vi "PLC_comm.vi"() -> ()   [LabVIEW 2017]
uses:
  <vilib>/Utility/error.llb/DialogType.ctl
  Control/PLC_Comm_State.ctl
  <vilib>/DATA AHEAD/SP7/typedefs/PLC Type.ctl
  <vilib>/DATA AHEAD/SP7/typedefs/S7 Connection.ctl
  f53d9a16-31ea-4c58-9ec6-4ab155e6634a.vi
  b767813d-b0bc-4642-82b7-59e8eeaf8486.vi
  cf2a4f70-d875-4391-b4be-4b1ea527ec99.vi
  f2e501b8-8033-40fd-b99e-90a89dd29cf5.vi
  a17ecfbb-e8aa-4e6f-9723-a9b27e8c0652.vi
  adc7d8b8-ea76-443b-992e-07ffa118bf03.vi
  3deaaee4-0312-4209-8b7c-ccc637c44985.vi
  <vilib>/addons/database/Connection.llb/DB Tools Open Connec (String).vi
  <vilib>/DATA AHEAD/SP7/functions/write/write Dint array.vi
  Global/DATA LOG.vi
  <vilib>/DATA AHEAD/SP7/functions/read/read String.vi
  <vilib>/DATA AHEAD/SP7/functions/read/read Dint array.vi
  Global/Global 1.vi
  <vilib>/DATA AHEAD/SP7/functions/write/writeString.vi
  <vilib>/DATA AHEAD/SP7/functions/read/read real array.vi
  <vilib>/addons/database/NI_Database_API.lvlib
  <vilib>/DATA AHEAD/SP7/SP7.lvlib
  84f8396c-11e3-4f6e-927f-d6cb52f8486f.vi
  edb3f7e3-deb4-4efd-b63a-82a20ab466dd.vi
  737c4a97-5810-4f09-bfe1-7e6a970161fd.vi
  98a23aa7-5d76-4ce5-89a1-7ffa2d6e86d6.vi
  065602cd-1ec6-46a4-aff5-3b00a0c776c3.vi
panel:
  out "error out 4":errorcluster
  out "error out 3":errorcluster
  out "IP1 8":string
  out "PLC 8":bool
  out "IP1 7":string
  out "PLC 7":bool
  out "IP1 6":string
  out "PLC 6":bool
  out "IP1 5":string
  out "PLC 5":bool
  out "PLC 4":bool
  out "PLC 3":bool
  out "PLC 1":bool
  out "IP1 4":string
  out "IP1 3":string
  out "IP1 2":string
  out "IP1":string
  in  "stop":bool
  out "error out":errorcluster
  in  "error in (no error)":errorcluster
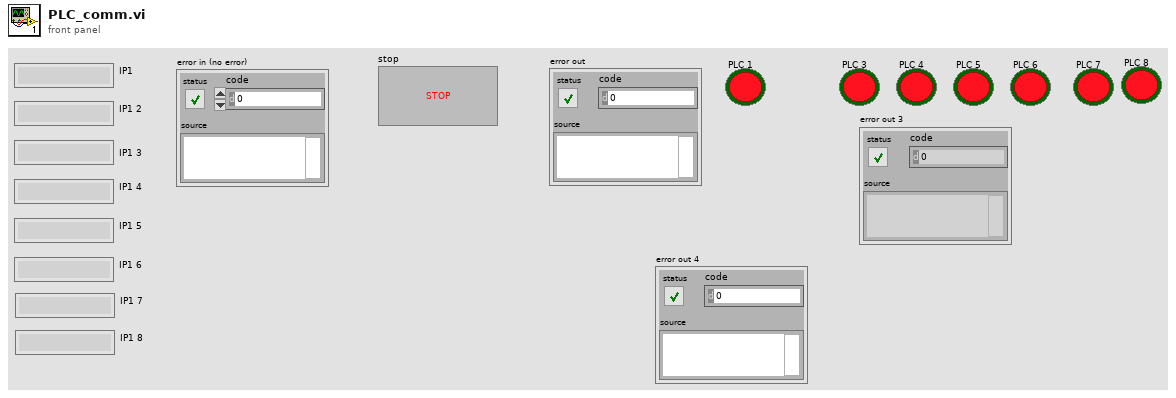
[diagram p1: front panel]
types:
  T1 = typedef "PLC_Comm_State.ctl" = enum16{"Int", "Connect", "Write", "Write2", "Write3", "Read", "Read2", "Read3", "Error", "Disconnect"}
  T2 = typedef "DialogType.ctl" = u16
  T3 = typedef "NI_Database_API.lvlib/Conn ObjectReference.ctl" = refnum<k1>
  T4 = typedef "SP7.lvlib/PLC Type.ctl" = enum16{"S7 200", "S7 300/400", "S7 1200", "S7 1500", "LOGO!8"}
  T5 = typedef "SP7.lvlib/S7 Connection.ctl" = cluster{"TCP Connection Ref":refnum<k5>, "IP address":string, "timeout ms":i32, "Connected?":bool, "PLC Type":T4, "Rack S7 400":u8, "Slot S7 400":u8, "PDU Size":u16, "connection semaphore":T6}
  T6 = typedef "Semaphore RefNum" = refnum<k1>
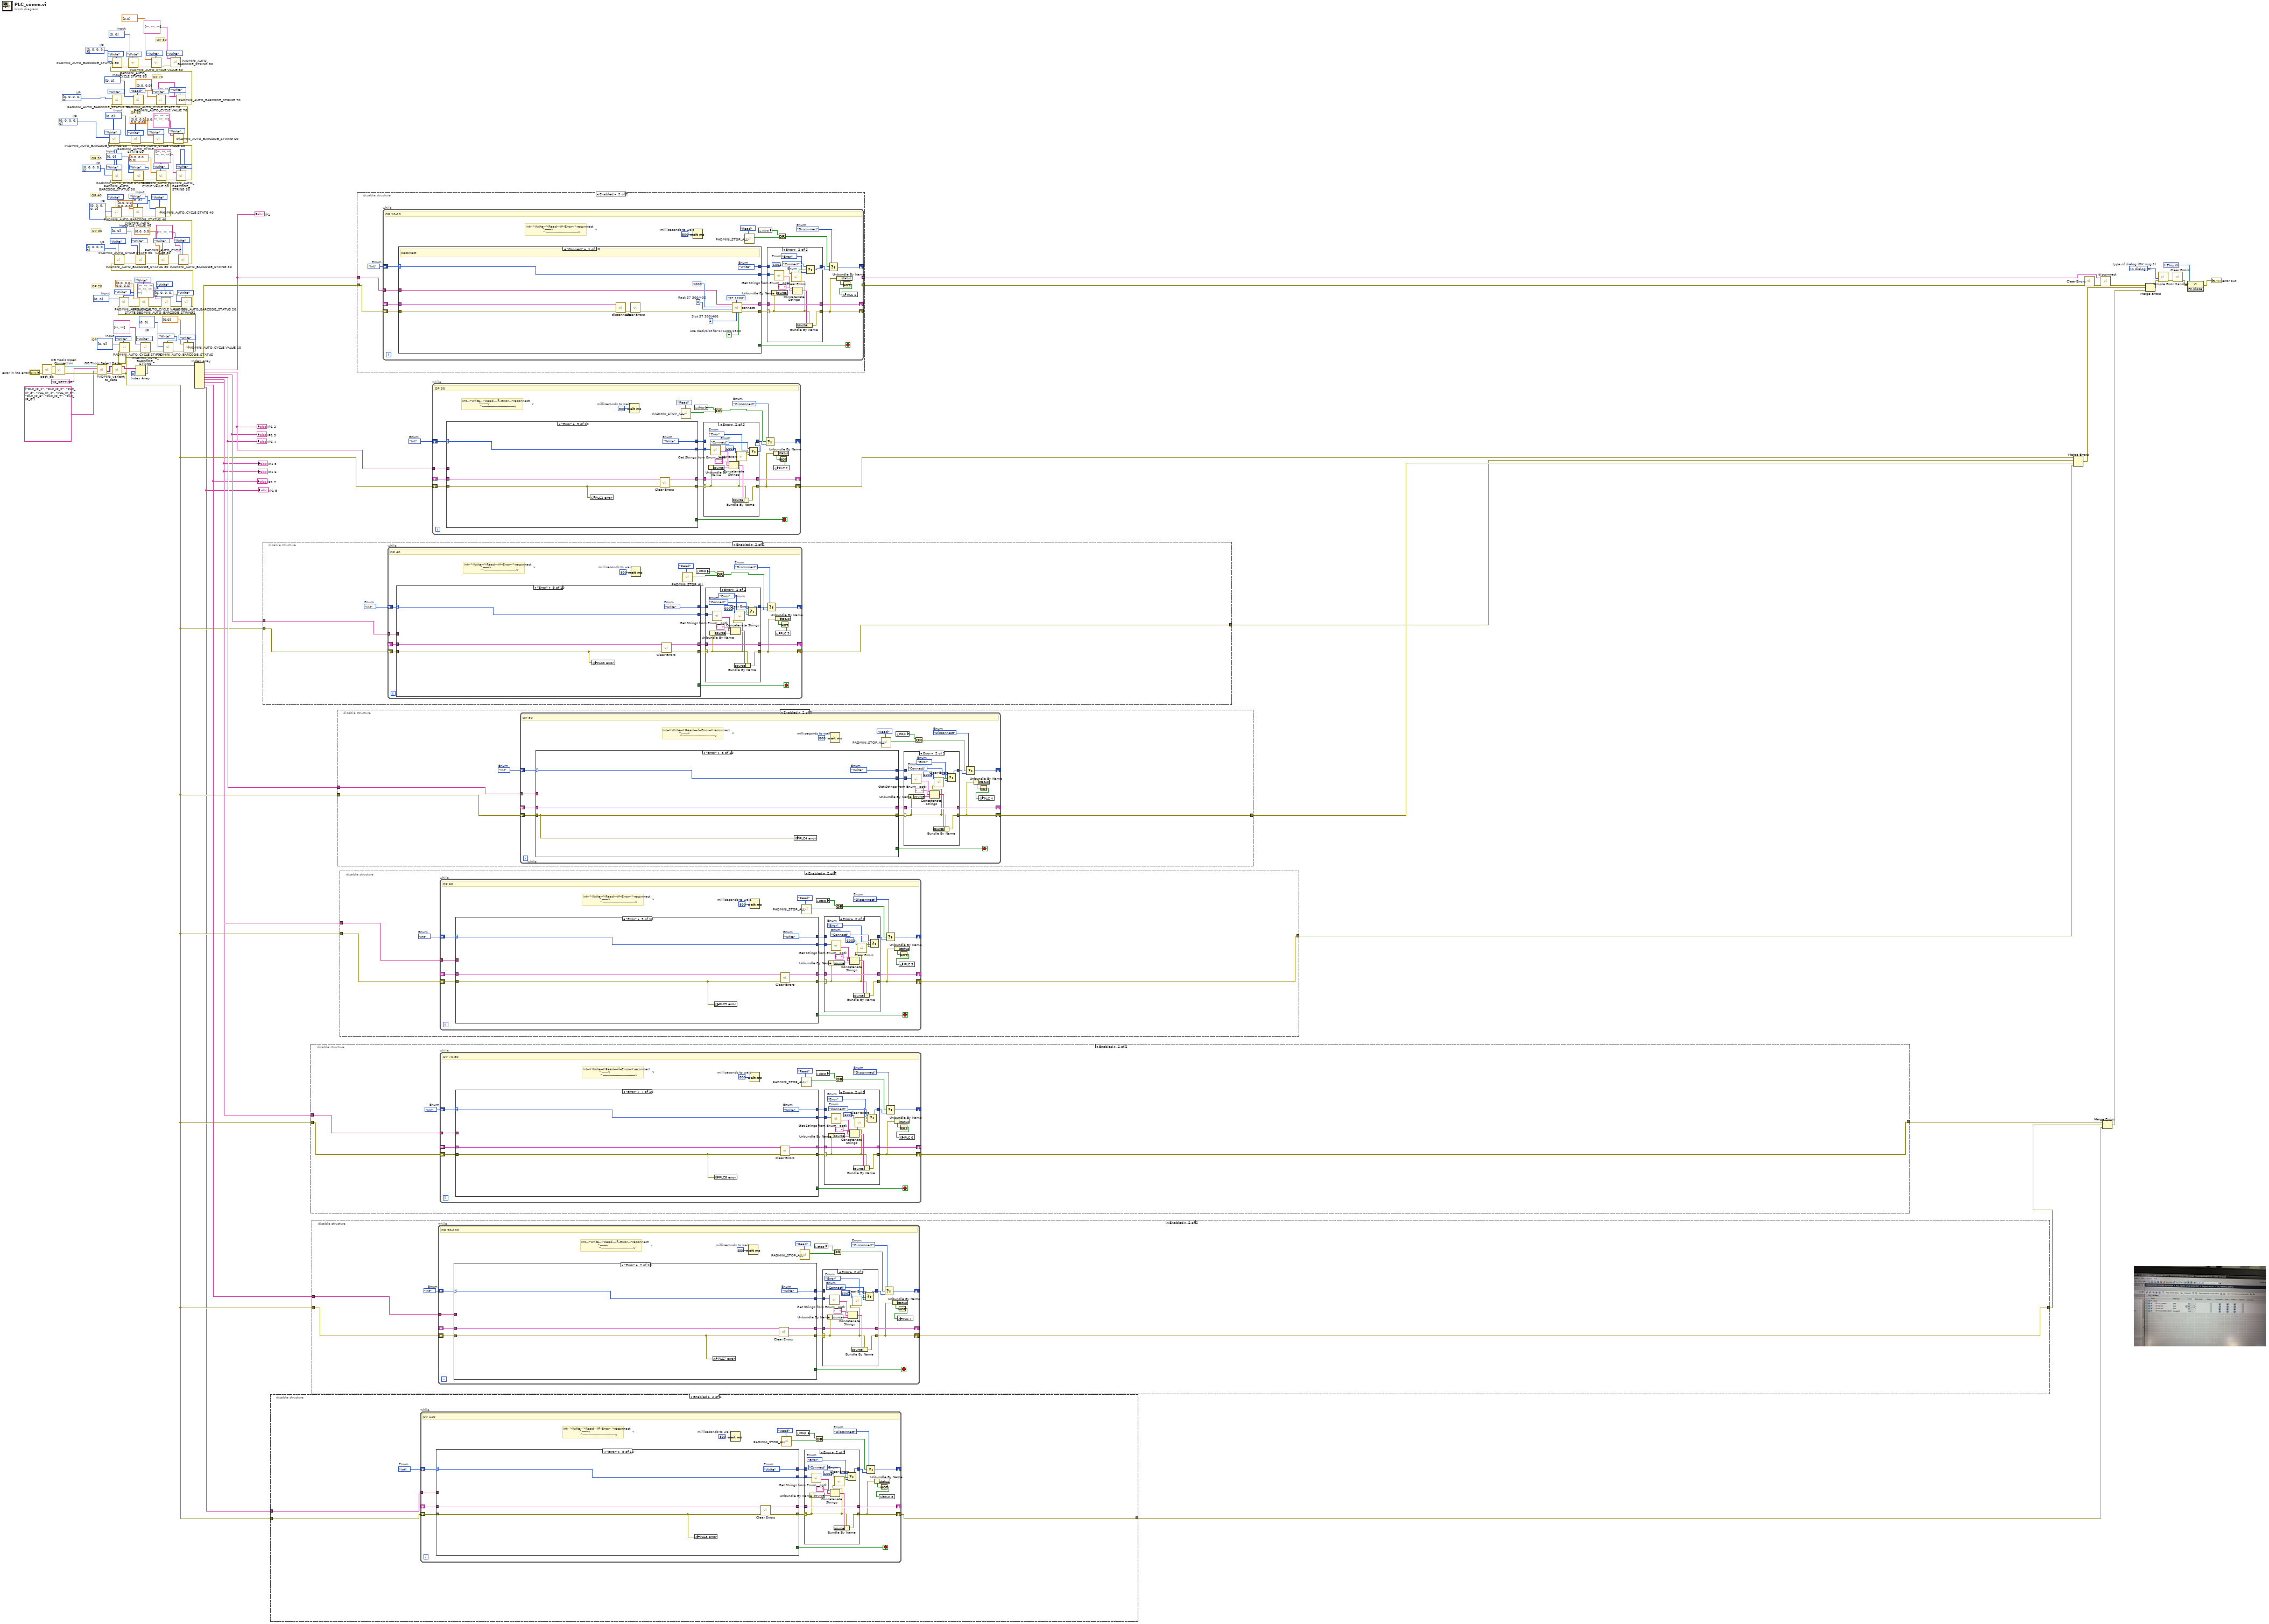
[diagram p0: block diagram]
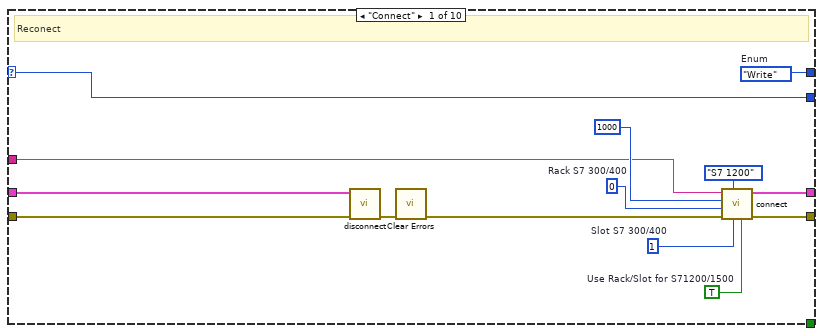
[diagram p3: hidden frame]
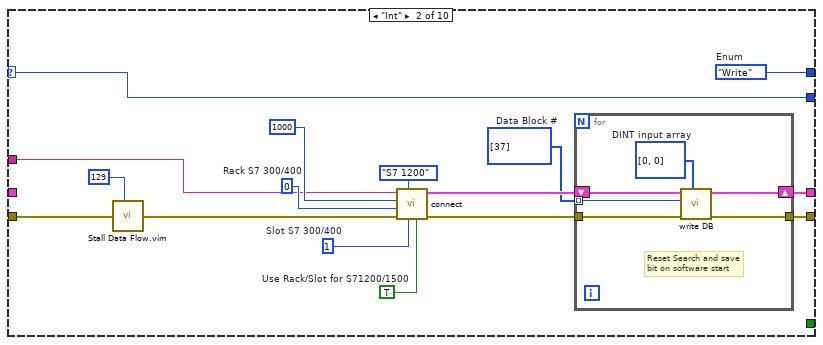
[diagram p4: hidden frame]
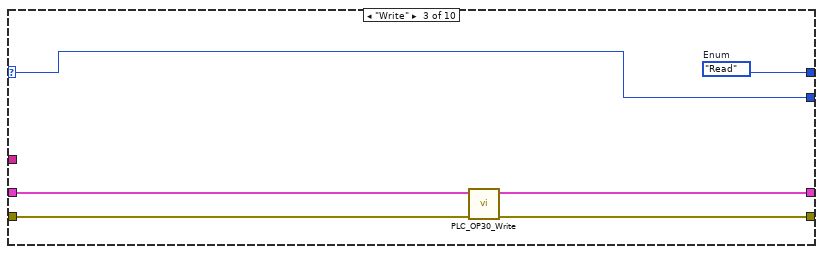
[diagram p5: hidden frame]
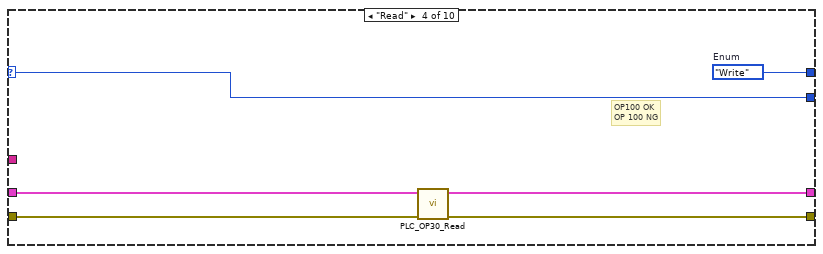
[diagram p6: hidden frame]
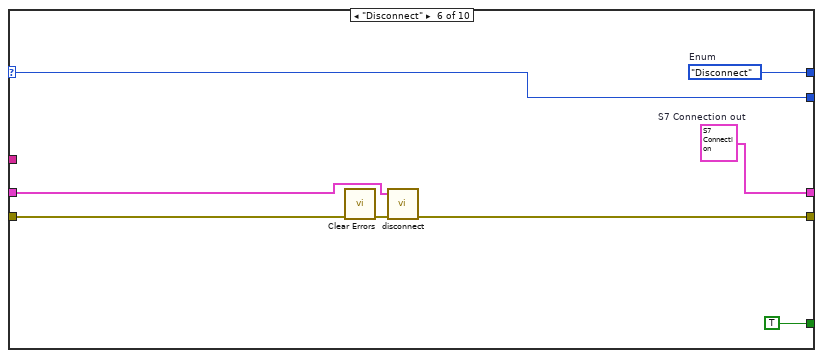
[diagram p7: hidden frame]
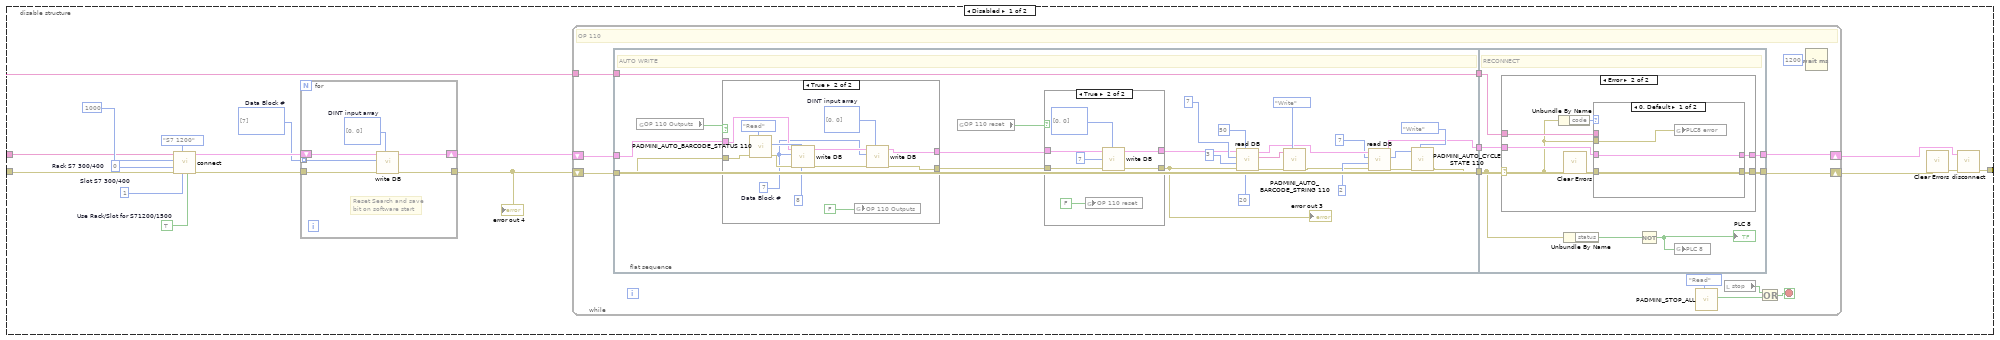
[diagram p12: hidden frame]
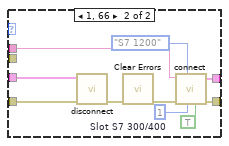
[diagram p16: hidden frame]
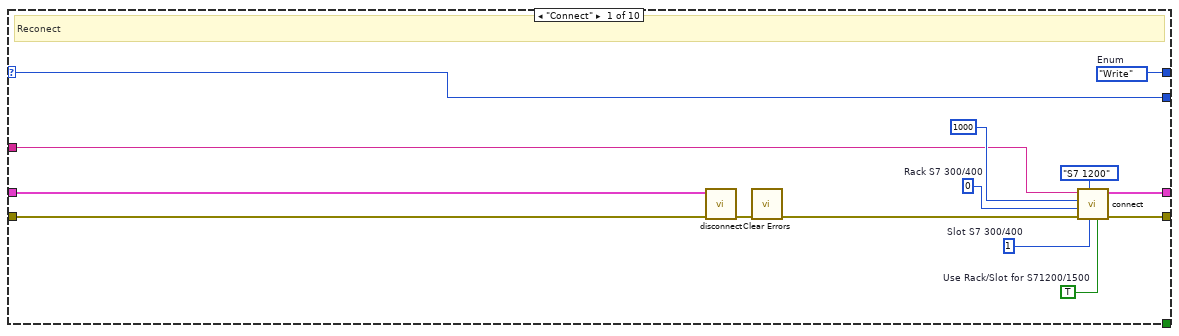
[diagram p18: hidden frame]
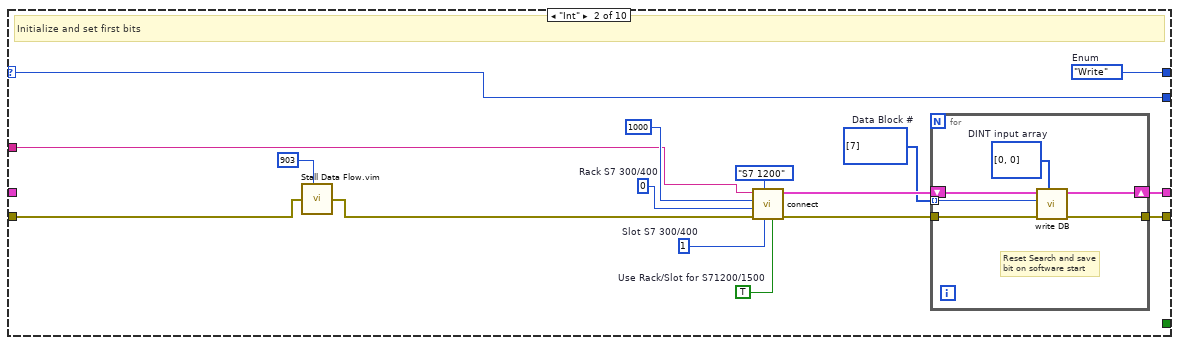
[diagram p19: hidden frame]
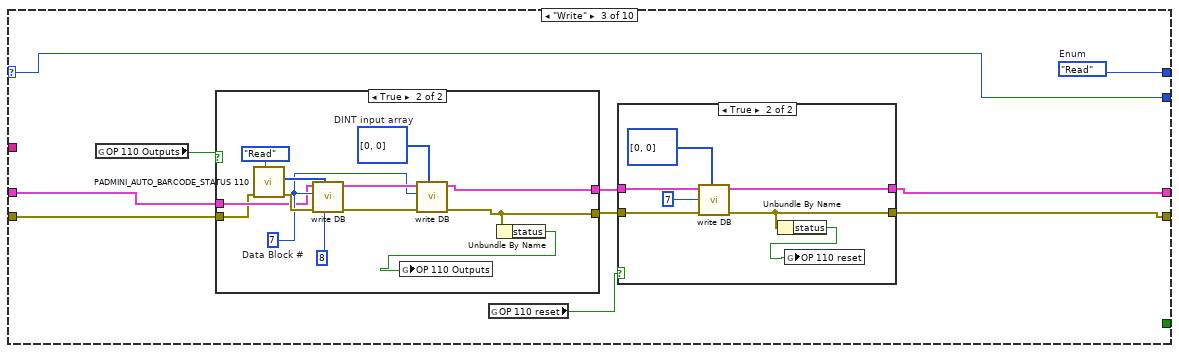
[diagram p20: hidden frame]
diagram:
  w1 = PLC_Comm_State."Int"  # Enum
  w10 = T2 0 items=["no dialog", "OK message", "continue or stop message", "OK message + warnings", "continue/stop + warnings"]  # type of dialog (OK msg:1)
  w12 = i32[] [0, 0, 0, 0, 0]  # I/P
  w13 = i32[] [0, 0]  # Input
  w15 = i32[] [0, 0]  # Input
  w16 = i32[] [0, 0]  # Input
  w18 = i32[] [0, 0]  # Input
  w14 = i32[] [0, 0, 0, 0, 0]  # I/P
  w17 = i32[] [0, 0, 0, 0, 0]  # I/P
  w19 = i32[] [0, 0, 0, 0, 0]  # I/P
  w20 = i32[] [0, 0, 0, 0, 0]  # I/P
  w21 = i32[] [0, 0]  # Input
  w22 = i32[] [0, 0]  # Input
  w23 = i32[] [0, 0, 0, 0, 0]  # I/P
  w24 = i32[] [0, 0, 0, 0, 0]  # I/P
  w25 = i32[] [0, 0]  # Input
  w26 = i32[] [0, 0]  # I/P
  w27 = i32[] [0, 0]  # Input
  # "OP 80"
  # "OP 70"
  # "OP 60"
  # "OP 50"
  # "OP 40"
  # "OP 30"
  # "OP 20"
  # "OP 10"
  n1 = call "path_db.vi"("error in"="error in (no error)") -> ("error out"=w128:errorcluster, "resulting string"=w133:string)  [unwired: 9 in]
  n2 = call-poly <vilib>:"DB Tools Open Connection.vi"("error in (no error)"=w128, "connection information"=w133) -> ("error out"=w132:errorcluster, "connection reference"=w131:T3)  [unwired: 6 in]
  n3 = call <vilib>:"DB Tools Select Data.vi"("error in (no error)"=w132, "columns"=string[] ["PLC_IP_1", "PLC_IP_2", "PLC_IP_3", "PLC_IP_4", "PLC_IP_5", "PLC_IP_6", "PLC_IP_7", "PLC_IP_8"], "table"="IP_SETTING", "connection reference"=w131) -> ("error out"=w130:errorcluster, "data"=w129:variant[][])  [unwired: 2 in, 1 out]
  n4 = call "PADMINI_varient_to_data.vi"("error in (no error)"=w130, "data"=w129) -> ("error out"=w9:errorcluster, "Array"=w124:string[][])  [unwired: 8 in]
  n5 = call "PADMINI_AUTO_CYCLE STATE.vi"("Enum"=enum16{"Read", "Write"}."Write", "error in (no error)"=w9, "Input"=w27) -> ("error out"=w114:errorcluster)  [unwired: 7 in, 1 out]
  n6 = Index Array(array=w124, index (row)=0) -> (element=w123:string[])  [unwired: 1 in]
  n7 = call "PADMINI_AUTO_BARCODE_STRING.vi"("Enum"=enum16{"Read", "Write"}."Write", "error in (no error)"=w114, "Input"=string[] ["", ""]) -> ("error out"=w111:errorcluster)  [unwired: 7 in, 1 out]
  n8 = call "PADMINI_AUTO_BARCODE_STATUS.vi"("Enum"=enum16{"Read", "Write"}."Write", "error in (no error)"=w111, "I/P"=w26) -> ("error out"=w109:errorcluster)  [unwired: 7 in, 1 out]
  n9 = call "PADMINI_AUTO_CYCLE VALUE 10.vi"("Enum"=enum16{"Read", "Write"}."Write", "error in (no error)"=w109, "Input"=dbl[] [0.0]) -> ("error out"=w103:errorcluster)  [unwired: 7 in, 1 out]
  n10 = call "PADMINI_AUTO_CYCLE STATE 20.vi"("Enum"=enum16{"Read", "Write"}."Write", "error in (no error)"=w103, "Input"=w13) -> ("error out"=w101:errorcluster)  [unwired: 7 in, 1 out]
  n11 = call "PADMINI_AUTO_CYCLE VALUE 20.vi"("Enum"=enum16{"Read", "Write"}."Write", "error in (no error)"=w101, "Input"=dbl[] [0.0, 0.0, 0.0, 0.0]) -> ("error out"=w97:errorcluster)  [unwired: 7 in, 1 out]
  n12 = call "PADMINI_AUTO_BARCODE_STRING2.vi"("Enum"=enum16{"Read", "Write"}."Write", "error in (no error)"=w97, "Input"=string[] ["", "", "", "", "", "", ""]) -> ("error out"=w95:errorcluster)  [unwired: 7 in, 1 out]
  n13 = call "PADMINI_AUTO_BARCODE_STATUS 20.vi"("Enum"=enum16{"Read", "Write"}."Write", "error in (no error)"=w95, "I/P"=w12) -> ("error out"=w93:errorcluster)  [unwired: 7 in, 1 out]
  n14 = call "PADMINI_AUTO_BARCODE_STATUS 30.vi"("Enum"=enum16{"Read", "Write"}."Write", "error in (no error)"=w93, "I/P"=w14) -> ("error out"=w90:errorcluster)  [unwired: 7 in, 1 out]
  n15 = call "PADMINI_AUTO_CYCLE STATE 30.vi"("Enum"=enum16{"Read", "Write"}."Write", "error in (no error)"=w90, "Input"=w15) -> ("error out"=w89:errorcluster)  [unwired: 7 in, 1 out]
  n16 = call "PADMINI_AUTO_CYCLE VALUE 30.vi"("Enum"=enum16{"Read", "Write"}."Write", "error in (no error)"=w89, "Input"=dbl[] [0.0, 0.0]) -> ("error out"=w86:errorcluster)  [unwired: 7 in, 1 out]
  n17 = call "PADMINI_AUTO_BARCODE_STRING 30.vi"("Enum"=enum16{"Read", "Write"}."Write", "error in (no error)"=w86, "Input"=string[] ["", "", ""]) -> ("error out"=w76:errorcluster)  [unwired: 7 in, 1 out]
  n18 = call "PADMINI_AUTO_BARCODE_STATUS 40.vi"("Enum"=enum16{"Read", "Write"}."Write", "error in (no error)"=w76, "I/P"=w17) -> ("error out"=w75:errorcluster)  [unwired: 7 in, 1 out]
  n19 = call "PADMINI_AUTO_CYCLE VALUE 40.vi"("Enum"=enum16{"Read", "Write"}."Write", "error in (no error)"=w75, "Input"=dbl[] [0.0, 0.0, 0.0, 0.0]) -> ("error out"=w74:errorcluster)  [unwired: 7 in, 1 out]
  n20 = call "PADMINI_AUTO_CYCLE STATE 40.vi"("Enum"=enum16{"Read", "Write"}."Write", "error in (no error)"=w74, "Input"=w16) -> ("error out"=w73:errorcluster)  [unwired: 7 in, 1 out]
  n21 = call "PADMINI_AUTO_BARCODE_STATUS 50.vi"("Enum"=enum16{"Read", "Write"}."Write", "error in (no error)"=w73, "I/P"=w19) -> ("error out"=w65:errorcluster)  [unwired: 7 in, 1 out]
  n22 = call "PADMINI_AUTO_CYCLE STATE 50.vi"("Enum"=enum16{"Read", "Write"}."Write", "error in (no error)"=w65, "Input"=w18) -> ("error out"=w69:errorcluster)  [unwired: 7 in, 1 out]
  n23 = call "PADMINI_AUTO_CYCLE VALUE 50.vi"("Enum"=enum16{"Read", "Write"}."Write", "error in (no error)"=w69, "Input"=dbl[] [0.0, 0.0, 0.0]) -> ("error out"=w66:errorcluster)  [unwired: 7 in, 1 out]
  n24 = call "PADMINI_AUTO_BARCODE_STRING 50.vi"("Enum"=enum16{"Read", "Write"}."Write", "error in (no error)"=w66, "Input"=string[] ["", "", "", "", "", ""]) -> ("error out"=w51:errorcluster)  [unwired: 7 in, 1 out]
  n25 = call "PADMINI_AUTO_BARCODE_STATUS 60.vi"("Enum"=enum16{"Read", "Write"}."Write", "error in (no error)"=w51, "I/P"=w20) -> ("error out"=w55:errorcluster)  [unwired: 7 in, 1 out]
  n26 = call "PADMINI_AUTO_CYCLE STATE 60.vi"("Enum"=enum16{"Read", "Write"}."Write", "error in (no error)"=w55, "Input"=w21) -> ("error out"=w57:errorcluster)  [unwired: 7 in, 1 out]
  n27 = call "PADMINI_AUTO_CYCLE VALUE 60.vi"("Enum"=enum16{"Read", "Write"}."Write", "error in (no error)"=w57, "Input"=dbl[] [0.0, 0.0, 0.0, 0.0, 0.0]) -> ("error out"=w60:errorcluster)  [unwired: 7 in, 1 out]
  n28 = call "PADMINI_AUTO_BARCODE_STRING 60.vi"("Enum"=enum16{"Read", "Write"}."Write", "error in (no error)"=w60, "Input"=string[] ["", "", "", "", "", ""]) -> ("error out"=w34:errorcluster)  [unwired: 7 in, 1 out]
  n29 = call "PADMINI_AUTO_BARCODE_STATUS 70.vi"("Enum"=enum16{"Read", "Write"}."Write", "error in (no error)"=w34, "I/P"=w23) -> ("error out"=w37:errorcluster)  [unwired: 7 in, 1 out]
  n30 = call "PADMINI_AUTO_CYCLE STATE 70.vi"("Enum"=enum16{"Read", "Write"}."Read", "error in (no error)"=w37, "Input"=w22) -> ("error out"=w49:errorcluster)  [unwired: 7 in, 1 out]
  n31 = call "PADMINI_AUTO_CYCLE VALUE 70.vi"("Enum"=enum16{"Read", "Write"}."Write", "error in (no error)"=w49, "Input"=dbl[] [0.0, 0.0]) -> ("error out"=w46:errorcluster)  [unwired: 7 in, 1 out]
  n32 = call "PADMINI_AUTO_BARCODE_STRING 70.vi"("Enum"=enum16{"Read", "Write"}."Write", "error in (no error)"=w46, "Input"=string[] ["", ""]) -> ("error out"=w31:errorcluster)  [unwired: 7 in, 1 out]
  n33 = call "PADMINI_AUTO_BARCODE_STATUS 80.vi"("Enum"=enum16{"Read", "Write"}."Write", "error in (no error)"=w31, "I/P"=w24) -> ("error out"=w38:errorcluster)  [unwired: 7 in, 1 out]
  n34 = call "PADMINI_AUTO_CYCLE STATE 80.vi"("Enum"=enum16{"Read", "Write"}."Write", "error in (no error)"=w38, "Input"=w25) -> ("error out"=w42:errorcluster)  [unwired: 7 in, 1 out]
  n35 = call "PADMINI_AUTO_CYCLE VALUE 80.vi"("Enum"=enum16{"Read", "Write"}."Write", "error in (no error)"=w42, "Input"=sgl[] [0.0]) -> ("error out"=w45:errorcluster)  [unwired: 7 in, 1 out]
  n36 = call "PADMINI_AUTO_BARCODE_STRING 80.vi"("Enum"=enum16{"Read", "Write"}."Write", "error in (no error)"=w45, "Input"=string[] ["", "", ""]) -> ()  [unwired: 7 in, 2 out]
  n37 = Index Array(array=w123) -> (element #1=w82:string, element #2=w83:string, element #3=w81:string, element #4=w71:string, element #5=w61:string, element #6=w30:string, element #7=w29:string, element #8=w8:string)  [unwired: 8 in]
  "IP1" <- w82
  "IP1 2" <- w83
  "IP1 3" <- w81
  "IP1 4" <- w71
  "IP1 5" <- w61
  "IP1 6" <- w30
  "IP1 7" <- w29
  "IP1 8" <- w8
  n38 = disable-structure shown="Enabled" {
    disable-tunnel: w81 -> [w148 w270]
    disable-tunnel: w9 -> [w139 w269]
    disable-tunnel: [w134 w268] -> w3
    frame Disabled {
      w136 = TRUE  # Use Rack/Slot for S71200/1500
      w137 = u8 0  # Rack S7 300/400
      w138 = u8 1  # Slot S7 300/400
      w144 = i32[] [0, 0]  # DINT input array
      # "Reset Search and save \nbit on software start"
      n39 = call <vilib>:"connect.vi"("Use Rack/Slot for S71200/1500"=w136, "Slot S7 300/400"=w138, "PLC Type"=PLC_Type."S7 1200" ("PLC Type 2"), "error in (no error)"=w139, "Rack S7 300/400"=w137, "timeout [ms]"=1000 ("timeout [ms] 2"), "IP address"=w148) -> ("error out"=w141:errorcluster, "S7 Connection out"=w140:T5)  [unwired: 3 in]
      n40 = call-poly <vilib>:"write DB.vi"("DINT input array"=w144, "error in (no error)"=w141, "Data Block #"=u16 56, "S7 Connection in"=w140) -> ("error out"=w143:errorcluster, "S7 Connection out"=w142:T5)  [unwired: 4 in, 2 out]
      n41 = while {
        shift-right: [w153] -> w146
        shift-left: w142 -> [w163]
        shift-right: [w161] -> w147
        shift-left: w143 -> [w162]
        tunnel: w148 -> [w152]
        stop <- w155 stop-if-true
        # "OP 40"
        n42 = flat-sequence {
          tunnel: [w165] -> w159
          tunnel: [w168] -> w154
          tunnel: w162 -> [w213]
          tunnel: w163 -> [w212]
          tunnel: w152 -> [w200]
          tunnel: [w200] -> w151
          tunnel: [w241] -> w161
          tunnel: [w240] -> w153
          tunnel: w159 -> [w243]
          tunnel: w154 -> [w242]
          tunnel: w151 -> [w239]
          frame #0 {
            w193 = u16 57 ("Data Block #")
            w164 = u16 56 ("Data Block #")
            # "AUTO WRITE"
            n43 = global read "DATA LOG.vi" "OP 40 Outputs"() -> (w211:bool)
            n44 = case shown="True" w211 {
              tunnel: w212 -> [w224 w237]
              tunnel: [w225 w229] -> w198
              tunnel: [w224 w231] -> w199
              tunnel: w213 -> [w225 w234]
              frame False {
              }
              frame True {
                w238 = u16 57  # Data Block #
                n45 = call "PADMINI_AUTO_BARCODE_STATUS 40.vi"("Enum"=enum16{"Read", "Write"}."Read", "error in (no error)"=w234) -> ("error out"=w233:errorcluster, "O/P"=w235:i32[])  [unwired: 8 in]
                n46 = global write "DATA LOG.vi" "OP 40 Outputs"(FALSE) -> ()
                n47 = call-poly <vilib>:"write DB.vi"("DINT input array"=w235, "error in (no error)"=w233, "Data Block #"=w238, "S7 Connection in"=w237) -> ("error out"=w228:errorcluster, "S7 Connection out"=w230:T5)  [unwired: 4 in, 2 out]
                n48 = call-poly <vilib>:"write DB.vi"("DINT input array"=i32[] [0], "error in (no error)"=w228, "Data Block #"=u16 56, "S7 Connection in"=w230) -> ("error out"=w229:errorcluster, "S7 Connection out"=w231:T5)  [unwired: 4 in, 2 out]
              }
            }
            n49 = global read "DATA LOG.vi" "OP 40 reset"() -> (w197:bool)
            n50 = global read "DATA LOG.vi" "Auto Cycle On"() -> (w175:bool)
            n51 = case shown="True" w197 {
              tunnel: w198 -> [w214 w223]
              tunnel: [w214 w222] -> w186
              tunnel: w199 -> [w215 w221]
              tunnel: [w215 w220] -> w187
              frame False {
              }
              frame True {
                n52 = global write "DATA LOG.vi" "OP 40 reset"(FALSE) -> ()
                n53 = call-poly <vilib>:"write DB.vi"("Item offset [byte]"=u16 4 ("Data Block #"), "DINT input array"=i32[] [0], "error in (no error)"=w223, "Data Block #"=u16 56, "S7 Connection in"=w221) -> ("error out"=w222:errorcluster, "S7 Connection out"=w220:T5)  [unwired: 3 in, 2 out]
              }
            }
            n54 = Boolean To (0,1)(Boolean=w175) -> (0, 1=w174:i16)
            n55 = Build Array(w174) -> (w173:i16[])
            n56 = global read "Global 1.vi" "Filtered BARCODE selected"() -> (w196:string[])
            n57 = call-poly <vilib>:"write DB.vi"("Item offset [byte]"=u32 20, "DINT input array"=w173, "error in (no error)"=w186, "Data Block #"=w193, "S7 Connection in"=w187) -> ("error out"=w191:errorcluster, "S7 Connection out"=w190:T5)  [unwired: 3 in, 2 out]
            n58 = call-poly <vilib>:"write DB.vi"("Item offset [byte]"=u32 24, "Input STRINGS"=w196, "error in (no error)"=w191, "String length reserved in DB (default=254)"=u16 15, "Data Block #"=w193, "S7 Connection in"=w190) -> ("error out"=w188:errorcluster, "S7 Connection out"=w189:T5)  [unwired: 2 in, 2 out]
            n59 = call-poly <vilib>:"read DB.vi"("Item offset [byte]"=u32 8, "error in (no error)"=w188, "items #"=u16 4 ("Items # [byte]"), "Data Block #"=w164, "S7 Connection in"=w189) -> ("error out"=w203:errorcluster, "REAL result array"=w201:sgl[], "S7 Connection out"=w209:T5)  [unwired: 4 in]
            n60 = call "PADMINI_AUTO_CYCLE VALUE 40.vi"("Enum"=enum16{"Read", "Write"}."Write", "error in (no error)"=w203, "Input"=w201) -> ("error out"=w202:errorcluster)  [unwired: 7 in, 1 out]
            n61 = call-poly <vilib>:"read DB.vi"("Item offset [byte]"=u32 24, "String length reserved in DB (default=254)"=u16 50, "error in (no error)"=w202, "items #"=u16 1 ("Items # [byte]"), "Data Block #"=w164, "S7 Connection in"=w209) -> ("error out"=w185:errorcluster, "STRING result Array"=w178:string[], "S7 Connection out"=w183:T5)  [unwired: 2 in, 1 out]
            n62 = call-poly <vilib>:"read DB.vi"("Item offset [byte]"=u32 76, "String length reserved in DB (default=254)"=u16 10, "error in (no error)"=w185, "items #"=u16 4 ("Items # [byte]"), "Data Block #"=w164, "S7 Connection in"=w183) -> ("error out"=w184:errorcluster, "STRING result Array"=w177:string[], "S7 Connection out"=w166:T5)  [unwired: 2 in, 1 out]
            n63 = Build Array (concatenate)(w178, w177) -> (w176:string[])
            n64 = call "PADMINI_AUTO_BARCODE_STRING 40.vi"("Enum"=enum16{"Read", "Write"}."Write", "error in (no error)"=w184, "Input"=w176) -> ("error out"=w167:errorcluster)  [unwired: 7 in, 1 out]
            n65 = call-poly <vilib>:"read DB.vi"("error in (no error)"=w167, "items #"=u16 2 ("Items # [byte]"), "Data Block #"=w164, "S7 Connection in"=w166) -> ("error out"=w172:errorcluster, "DINT result array"=w171:i32[], "S7 Connection out"=w165:T5)  [unwired: 5 in]
            n66 = call "PADMINI_AUTO_CYCLE STATE 40.vi"("Enum"=enum16{"Read", "Write"}."Write", "error in (no error)"=w172, "Input"=w171) -> ("error out"=w168:errorcluster)  [unwired: 7 in, 1 out]
          }
          frame #1 {
            # "RECONNECT"
            n67 = case shown="Error" w242 {
              selector: w242 -> [w247 w248]
              tunnel: [w246 w252] -> w240
              tunnel: [w247 w253] -> w241
              tunnel: w243 -> [w246 w251]
              tunnel: w239 -> [_ w250]
              frame No Error {
              }
              frame Error {
                n68 = Unbundle By Name(w248) -> ("code"=w249:i32)
                n69 = call <vilib>:"Clear Errors.vi"("error in (no error)"=w248) -> ("error out"=w254:errorcluster)  [unwired: 5 in, 1 out]
                n70 = case shown="0, Default" w249 {
                  tunnel: w254 -> [w256 w267]
                  tunnel: [w256 w265] -> w253
                  tunnel: [w257 w264] -> w252
                  tunnel: w251 -> [w257 w261]
                  tunnel: w250 -> [_ w260]
                  tunnel: w248 -> [w255 _]
                  frame 0, Default {
                    n71 = global write "Global 1.vi" "PLC3 error"(w255) -> ()
                  }
                  frame 1 {
                    n72 = call <vilib>:"disconnect.vi"("error in (no error)"=w267, "S7 Connection in"=w261) -> ("error out"=w266:errorcluster)  [unwired: 8 in, 1 out]
                    n73 = call <vilib>:"Clear Errors.vi"("error in (no error)"=w266) -> ("error out"=w263:errorcluster)  [unwired: 5 in, 1 out]
                    n74 = call <vilib>:"connect.vi"("Use Rack/Slot for S71200/1500"=TRUE, "Slot S7 300/400"=u8 1, "PLC Type"=PLC_Type."S7 1200" ("PLC Type 2"), "error in (no error)"=w263, "IP address"=w260) -> ("error out"=w265:errorcluster, "S7 Connection out"=w264:T5)  [unwired: 5 in]
                  }
                }
              }
            }
            n75 = Unbundle By Name(w242) -> ("status"=w245:bool)
            n76 = Not(x=w245) -> (.not. x?=w244:bool)
            "PLC 3" <- w244
            n77 = global write "Global 1.vi" "PLC 3"(w244) -> ()
          }
        }
        n78 = call "PADMINI_STOP_ALL.vi"("Enum"=enum16{"Read", "Write"}."Read") -> ("Boolean 2"=w157:bool)  [unwired: 9 in, 1 out]
        n79 = local read "stop"() -> (w156:bool)
        n80 = Or(x=w156, y=w157) -> (x .or. y?=w155:bool)
        n81 = Wait (ms)(milliseconds to wait=u32 1200) -> ()  [unwired: 1 out]
      }
      n82 = call <vilib>:"Clear Errors.vi"("error in (no error)"=w147) -> ("error out"=w135:errorcluster)  [unwired: 5 in, 1 out]
      n83 = call <vilib>:"disconnect.vi"("error in (no error)"=w135, "S7 Connection in"=w146) -> ("error out"=w134:errorcluster)  [unwired: 8 in, 1 out]
    }
    frame Enabled {
      w271 = PLC_Comm_State."Int"  # Enum
      n84 = while {
        shift-right: [w282] -> _
        shift-left: w271 -> [w291]
        shift-right: [w272] -> w268
        shift-left: w269 -> [w290]
        shift-right: [w285] -> _
        shift-left: _ -> [w289]
        tunnel: w270 -> [w288]
        stop <- w283 stop-if-true
        w279 = PLC_Comm_State."Disconnect"  # Enum
        w287 = u32 800  # milliseconds to wait
        # "Int-->Write-->Read---if--Error-->reconnect\n               ^------v                                       v\n                ^------------------------------v"
        # "OP 40"
        n85 = case shown="\"Error\"" w291 {
          selector: w291 -> [w310 w328 w366 w419 w431 w435 _ _ _ _]
          tunnel: [w315 w330 w347 w394 w432 w440 w442 w445 w447 w449] -> w292
          tunnel: [w316 w326 w345 w392 w433 w437 w443 w444 w446 w448] -> w284
          tunnel: w290 -> [w313 w324 w348 w395 w429 w438 w442 w445 w447 w449]
          tunnel: w289 -> [w311 _ w346 w393 w433 w439 w443 w444 w446 w448]
          tunnel: w288 -> [w317 w329 _ _ _ _ _ _ _ _]
          tunnel: [w309 w327 w365 w418 w430 w434 _ _ _ _] -> w286
          tunnel: [_ _ _ _ _ TRUE _ _ _ _] -> w283
          tunnel: [w310 w328 w366 w419 w431 w435 _ _ _ _] -> w280
          frame "Connect" {
            w309 = PLC_Comm_State."Write"  # Enum
            w322 = TRUE  # Use Rack/Slot for S71200/1500
            w321 = u8 1  # Slot S7 300/400
            w319 = u8 0  # Rack S7 300/400
            # "Reconect"
            n86 = call <vilib>:"disconnect.vi"("error in (no error)"=w313, "S7 Connection in"=w311) -> ("error out"=w314:errorcluster)  [unwired: 8 in, 1 out]
            n87 = call <vilib>:"Clear Errors.vi"("error in (no error)"=w314) -> ("error out"=w312:errorcluster)  [unwired: 5 in, 1 out]
            n88 = call <vilib>:"connect.vi"("Use Rack/Slot for S71200/1500"=w322, "Slot S7 300/400"=w321, "PLC Type"=PLC_Type."S7 1200" ("PLC Type 2"), "error in (no error)"=w312, "Rack S7 300/400"=w319, "timeout [ms]"=1000 ("timeout [ms] 2"), "IP address"=w317) -> ("error out"=w315:errorcluster, "S7 Connection out"=w316:T5)  [unwired: 3 in]
          }
          frame "Int" {
            w327 = PLC_Comm_State."Write"  # Enum
            w331 = TRUE  # Use Rack/Slot for S71200/1500
            w332 = u8 1  # Slot S7 300/400
            w333 = u8 0  # Rack S7 300/400
            w334 = u16[] [56]  # Data Block #
            n89 = call "Stall Data Flow.vim"("value in"=w324, "milliseconds to wait"=u32 258) -> ("value out"=w323:errorcluster)  [unwired: 1 out]
            n90 = call <vilib>:"connect.vi"("Use Rack/Slot for S71200/1500"=w331, "Slot S7 300/400"=w332, "PLC Type"=PLC_Type."S7 1200" ("PLC Type 2"), "error in (no error)"=w323, "Rack S7 300/400"=w333, "timeout [ms]"=1000 ("timeout [ms] 2"), "IP address"=w329) -> ("error out"=w336:errorcluster, "S7 Connection out"=w335:T5)  [unwired: 3 in]
            n91 = for {
              tunnel: w334 -> [w344] mode=indexing
              shift-right: [w342] -> w326
              shift-left: w335 -> [w340]
              tunnel: w336 -> [w341]
              tunnel: [w339] -> w330
              w343 = i32[] [0, 0]  # DINT input array
              # "Reset Search and save \nbit on software start"
              n92 = call-poly <vilib>:"write DB.vi"("DINT input array"=w343, "error in (no error)"=w341, "Data Block #"=w344, "S7 Connection in"=w340) -> ("error out"=w339:errorcluster, "S7 Connection out"=w342:T5)  [unwired: 4 in, 2 out]
            }
          }
          frame "Write" {
            w350 = u16 57 ("Data Block #")
            w365 = PLC_Comm_State."Read"  # Enum
            n93 = global read "DATA LOG.vi" "OP 40 Outputs"() -> (w364:bool)
            n94 = case shown="True" w364 {
              tunnel: w346 -> [w377 w379]
              tunnel: [w378 w381] -> w362
              tunnel: [w377 w386] -> w363
              tunnel: w348 -> [w378 w388]
              frame False {
              }
              frame True {
                w391 = u16 57  # Data Block #
                n95 = call "PADMINI_AUTO_BARCODE_STATUS 40.vi"("Enum"=enum16{"Read", "Write"}."Read", "error in (no error)"=w388) -> ("error out"=w387:errorcluster, "O/P"=w389:i32[])  [unwired: 8 in]
                n96 = call-poly <vilib>:"write DB.vi"("DINT input array"=w389, "error in (no error)"=w387, "Data Block #"=w391, "S7 Connection in"=w379) -> ("error out"=w384:errorcluster, "S7 Connection out"=w385:T5)  [unwired: 4 in, 2 out]
                n97 = call-poly <vilib>:"write DB.vi"("DINT input array"=i32[] [0], "error in (no error)"=w384, "Data Block #"=u16 56, "S7 Connection in"=w385) -> ("error out"=w381:errorcluster, "S7 Connection out"=w386:T5)  [unwired: 4 in, 2 out]
                n98 = Unbundle By Name(w381) -> ("status"=w380:bool)
                n99 = global write "DATA LOG.vi" "OP 40 Outputs"(w380) -> ()
              }
            }
            n100 = global read "DATA LOG.vi" "OP 40 reset"() -> (w361:bool)
            n101 = case shown="True" w361 {
              tunnel: w362 -> [w367 w376]
              tunnel: [w367 w371] -> w356
              tunnel: w363 -> [w368 w375]
              tunnel: [w368 w369] -> w357
              frame False {
              }
              frame True {
                n102 = call-poly <vilib>:"write DB.vi"("Item offset [byte]"=u16 4 ("Data Block #"), "DINT input array"=i32[] [0], "error in (no error)"=w376, "Data Block #"=u16 56, "S7 Connection in"=w375) -> ("error out"=w371:errorcluster, "S7 Connection out"=w369:T5)  [unwired: 3 in, 2 out]
                n103 = Unbundle By Name(w371) -> ("status"=w370:bool)
                n104 = global write "DATA LOG.vi" "OP 40 reset"(w370) -> ()
              }
            }
            n105 = global read "DATA LOG.vi" "Auto Cycle On"() -> (w355:bool)
            n106 = global read "Global 1.vi" "Filtered BARCODE selected"() -> (w360:string[])
            n107 = Boolean To (0,1)(Boolean=w355) -> (0, 1=w354:i16)
            n108 = Build Array(w354) -> (w353:i16[])
            n109 = call-poly <vilib>:"write DB.vi"("Item offset [byte]"=u32 20, "DINT input array"=w353, "error in (no error)"=w356, "Data Block #"=w350, "S7 Connection in"=w357) -> ("error out"=w359:errorcluster, "S7 Connection out"=w358:T5)  [unwired: 3 in, 2 out]
            n110 = call-poly <vilib>:"write DB.vi"("Item offset [byte]"=u32 24, "Input STRINGS"=w360, "error in (no error)"=w359, "String length reserved in DB (default=254)"=u16 15, "Data Block #"=w350, "S7 Connection in"=w358) -> ("error out"=w347:errorcluster, "S7 Connection out"=w345:T5)  [unwired: 2 in, 2 out]
          }
          frame "Read" {
            w404 = u16 56 ("Data Block #")
            w418 = PLC_Comm_State."Write"  # Enum
            n111 = call-poly <vilib>:"read DB.vi"("Item offset [byte]"=u32 8, "error in (no error)"=w395, "items #"=u16 4 ("Items # [byte]"), "Data Block #"=w404, "S7 Connection in"=w393) -> ("error out"=w414:errorcluster, "REAL result array"=w417:sgl[], "S7 Connection out"=w415:T5)  [unwired: 4 in]
            n112 = call-poly <vilib>:"read DB.vi"("Item offset [byte]"=u32 24, "String length reserved in DB (default=254)"=u16 50, "error in (no error)"=w414, "items #"=u16 1 ("Items # [byte]"), "Data Block #"=w404, "S7 Connection in"=w415) -> ("error out"=w413:errorcluster, "STRING result Array"=w410:string[], "S7 Connection out"=w411:T5)  [unwired: 2 in, 1 out]
            n113 = call-poly <vilib>:"read DB.vi"("Item offset [byte]"=u32 76, "String length reserved in DB (default=254)"=u16 10, "error in (no error)"=w413, "items #"=u16 4 ("Items # [byte]"), "Data Block #"=w404, "S7 Connection in"=w411) -> ("error out"=w412:errorcluster, "STRING result Array"=w409:string[], "S7 Connection out"=w406:T5)  [unwired: 2 in, 1 out]
            n114 = Build Array (concatenate)(w410, w409) -> (w416:string[])
            n115 = call-poly <vilib>:"read DB.vi"("error in (no error)"=w412, "items #"=u16 2 ("Items # [byte]"), "Data Block #"=w404, "S7 Connection in"=w406) -> ("error out"=w408:errorcluster, "DINT result array"=w407:i32[], "S7 Connection out"=w392:T5)  [unwired: 5 in]
            n116 = case shown="No Error" w408 {
              selector: w408 -> [w423 w428]
              tunnel: w407 -> [w427 _]
              tunnel: w416 -> [w425 _]
              tunnel: w417 -> [w421 _]
              tunnel: [w420 w428] -> w394
              frame No Error {
                w422 = enum16{"Read", "Write"}."Write" ("Enum")
                n117 = call "PADMINI_AUTO_CYCLE VALUE 40.vi"("Enum"=w422, "error in (no error)"=w423, "Input"=w421) -> ("error out"=w424:errorcluster)  [unwired: 7 in, 1 out]
                n118 = call "PADMINI_AUTO_BARCODE_STRING 40.vi"("Enum"=w422, "error in (no error)"=w424, "Input"=w425) -> ("error out"=w426:errorcluster)  [unwired: 7 in, 1 out]
                n119 = call "PADMINI_AUTO_CYCLE STATE 40.vi"("Enum"=w422, "error in (no error)"=w426, "Input"=w427) -> ("error out"=w420:errorcluster)  [unwired: 7 in, 1 out]
              }
              frame Error {
              }
            }
          }
          frame "Error" {
            w430 = PLC_Comm_State."Write"  # Enum
            n120 = global write "Global 1.vi" "PLC3 error"(w429) -> ()
            n121 = call <vilib>:"Clear Errors.vi"("error in (no error)"=w429) -> ("error out"=w432:errorcluster)  [unwired: 5 in, 1 out]
          }
          frame "Disconnect" {
            w434 = PLC_Comm_State."Disconnect"  # Enum
            w437 = T5 {"TCP Connection Ref"=refnum, "IP address"="", "timeout ms"=5000, "Connected?"=FALSE, "PLC Type"=enum."S7 1200", "Rack S7 400"=0, "Slot S7 400"=0, "PDU Size"=0, "connection semaphore"=refnum}  # S7 Connection out
            n122 = call <vilib>:"Clear Errors.vi"("error in (no error)"=w438) -> ("error out"=w441:errorcluster)  [unwired: 5 in, 1 out]
            n123 = call <vilib>:"disconnect.vi"("error in (no error)"=w441, "S7 Connection in"=w439) -> ("error out"=w440:errorcluster)  [unwired: 8 in, 1 out]
          }
          frame "Write2" {
            # "No Use"
          }
          frame "Write3" {
            # "No Use"
          }
          frame "Read2" {
            # "No Use"
          }
          frame "Read3" {
            # "No Use"
          }
        }
        n124 = Wait (ms)(milliseconds to wait=w287) -> ()  [unwired: 1 out]
        n125 = call "PADMINI_STOP_ALL.vi"("Enum"=enum16{"Read", "Write"}."Read") -> ("Boolean 2"=w278:bool)  [unwired: 9 in, 1 out]
        n126 = local read "stop"() -> (w277:bool)
        n127 = case shown="Error" w292 {
          selector: w292 -> [w295 w298]
          tunnel: [w295 w302] -> w272
          tunnel: [w294 w297] -> w281
          tunnel: w286 -> [w294 _]
          tunnel: [w293 w308] -> w285
          tunnel: w284 -> [w293 w308]
          tunnel: w280 -> [_ w306]
          frame No Error {
          }
          frame Error {
            w299 = PLC_Comm_State."Connect"  # Enum
            w296 = PLC_Comm_State."Error"  # Enum
            n128 = Unbundle By Name(w298) -> ("source"=w307:string)
            n129 = call <userlib>:"Get Strings from Enum__ogtk.vi"("Enum"=w306) -> ("String Value"=w305:string)  [unwired: 7 in, 3 out]
            n130 = Concatenate Strings(w305, "    " ("string"), w307) -> (w303:string)
            n131 = Bundle By Name(cluster=w298, "source"=w303) -> (w302:errorcluster)
            n132 = call <vilib>:"Clear Errors.vi"("error in (no error)"=w298, "specific error code to clear (0: all)"=6002) -> ("specific error cleared?"=w301:bool)  [unwired: 4 in, 1 out]
            n133 = Select(t=w299, s=w301, f=w296) -> (s? t:f=w297:T1)
          }
        }
        n134 = Or(x=w277, y=w278) -> (x .or. y?=w275:bool)
        n135 = Select(t=w279, s=w275, f=w281) -> (s? t:f=w282:T1)
        n136 = Unbundle By Name(w272) -> ("status"=w274:bool)
        n137 = Not(x=w274) -> (.not. x?=w273:bool)
        n138 = global write "Global 1.vi" "PLC 3"(w273) -> ()
      }
    }
  }
  n139 = disable-structure shown="Enabled" {
    disable-tunnel: w9 -> [w459 w564]
    disable-tunnel: w8 -> [w457 w565]
    disable-tunnel: [w453 w563] -> w7
    frame Disabled {
      w450 = TRUE  # Use Rack/Slot for S71200/1500
      w451 = u8 1  # Slot S7 300/400
      w452 = u8 0  # Rack S7 300/400
      w458 = u16[] [7]  # Data Block #
      n140 = call <vilib>:"connect.vi"("Use Rack/Slot for S71200/1500"=w450, "Slot S7 300/400"=w451, "PLC Type"=PLC_Type."S7 1200" ("PLC Type 2"), "error in (no error)"=w459, "Rack S7 300/400"=w452, "timeout [ms]"=1000 ("timeout [ms] 2"), "IP address"=w457) -> ("error out"=w461:errorcluster, "S7 Connection out"=w460:T5)  [unwired: 3 in]
      n141 = for {
        tunnel: w458 -> [w471] mode=indexing
        shift-right: [w469] -> w464
        shift-left: w460 -> [w466]
        tunnel: w461 -> [w467]
        tunnel: [w468] -> w465
        w470 = i32[] [0, 0]  # DINT input array
        # "Reset Search and save \nbit on software start"
        n142 = call-poly <vilib>:"write DB.vi"("DINT input array"=w470, "error in (no error)"=w467, "Data Block #"=w471, "S7 Connection in"=w466) -> ("error out"=w468:errorcluster, "S7 Connection out"=w469:T5)  [unwired: 4 in, 2 out]
      }
      "error out 4" <- w465
      n143 = while {
        shift-right: [w474] -> w454
        shift-left: w464 -> [w484]
        shift-right: [w482] -> w455
        shift-left: w465 -> [w483]
        tunnel: w457 -> [w473]
        stop <- w476 stop-if-true
        # "OP 110"
        n144 = flat-sequence {
          tunnel: [w488] -> w480
          tunnel: [w489] -> w475
          tunnel: w483 -> [w507]
          tunnel: w484 -> [w508]
          tunnel: w473 -> [w509]
          tunnel: [w509] -> w472
          tunnel: [w536] -> w482
          tunnel: [w535] -> w474
          tunnel: w480 -> [w538]
          tunnel: w475 -> [w537]
          tunnel: w472 -> [w534]
          frame #0 {
            # "AUTO WRITE"
            n145 = global read "DATA LOG.vi" "OP 110 Outputs"() -> (w506:bool)
            n146 = case shown="True" w506 {
              tunnel: [w519 w524] -> w498
              tunnel: [w520 w525] -> w497
              tunnel: w507 -> [w519 w529]
              tunnel: w508 -> [w520 w528]
              frame False {
              }
              frame True {
                w521 = i32[] [0, 0]  # DINT input array
                w522 = u16 7  # Data Block #
                n147 = call "PADMINI_AUTO_BARCODE_STATUS 110.vi"("Enum"=enum16{"Read", "Write"}."Read", "error in (no error)"=w529) -> ("error out"=w531:errorcluster, "O/P"=w532:i32[])  [unwired: 8 in]
                n148 = call-poly <vilib>:"write DB.vi"("Item offset [byte]"=u32 8, "DINT input array"=w532, "error in (no error)"=w531, "Data Block #"=w522, "S7 Connection in"=w528) -> ("error out"=w523:errorcluster, "S7 Connection out"=w526:T5)  [unwired: 3 in, 2 out]
                n149 = global write "DATA LOG.vi" "OP 110 Outputs"(FALSE) -> ()
                n150 = call-poly <vilib>:"write DB.vi"("DINT input array"=w521, "error in (no error)"=w523, "Data Block #"=w522, "S7 Connection in"=w526) -> ("error out"=w524:errorcluster, "S7 Connection out"=w525:T5)  [unwired: 4 in, 2 out]
              }
            }
            n151 = global read "DATA LOG.vi" "OP 110 reset"() -> (w495:bool)
            n152 = case shown="True" w495 {
              tunnel: w498 -> [w510 w518]
              tunnel: [w510 w517] -> w499
              tunnel: w497 -> [w511 w516]
              tunnel: [w511 w515] -> w496
              frame False {
              }
              frame True {
                n153 = global write "DATA LOG.vi" "OP 110 reset"(FALSE) -> ()
                n154 = call-poly <vilib>:"write DB.vi"("DINT input array"=i32[] [0, 0], "error in (no error)"=w518, "Data Block #"=u16 7, "S7 Connection in"=w516) -> ("error out"=w517:errorcluster, "S7 Connection out"=w515:T5)  [unwired: 4 in, 2 out]
              }
            }
            "error out 3" <- w499
            n155 = call-poly <vilib>:"read DB.vi"("Item offset [byte]"=u32 20, "String length reserved in DB (default=254)"=u16 50, "error in (no error)"=w499, "items #"=u16 3 ("Items # [byte]"), "Data Block #"=u16 7, "S7 Connection in"=w496) -> ("error out"=w501:errorcluster, "STRING result Array"=w502:string[], "S7 Connection out"=w487:T5)  [unwired: 2 in, 1 out]
            n156 = call "PADMINI_AUTO_BARCODE_STRING 110.vi"("Enum"=enum16{"Read", "Write"}."Write", "error in (no error)"=w501, "Input"=w502) -> ("error out"=w490:errorcluster)  [unwired: 7 in, 1 out]
            n157 = call-poly <vilib>:"read DB.vi"("error in (no error)"=w490, "items #"=u16 2 ("Items # [byte]"), "Data Block #"=u16 7, "S7 Connection in"=w487) -> ("error out"=w494:errorcluster, "DINT result array"=w493:i32[], "S7 Connection out"=w488:T5)  [unwired: 5 in]
            n158 = call "PADMINI_AUTO_CYCLE STATE 110.vi"("Enum"=enum16{"Read", "Write"}."Write", "error in (no error)"=w494, "Input"=w493) -> ("error out"=w489:errorcluster)  [unwired: 7 in, 1 out]
          }
          frame #1 {
            # "RECONNECT"
            n159 = case shown="Error" w537 {
              selector: w537 -> [w542 w543]
              tunnel: [w541 w547] -> w535
              tunnel: [w542 w548] -> w536
              tunnel: w538 -> [w541 w546]
              tunnel: w534 -> [_ w545]
              frame No Error {
              }
              frame Error {
                n160 = Unbundle By Name(w543) -> ("code"=w544:i32)
                n161 = call <vilib>:"Clear Errors.vi"("error in (no error)"=w543) -> ("error out"=w549:errorcluster)  [unwired: 5 in, 1 out]
                n162 = case shown="0, Default" w544 {
                  tunnel: w549 -> [w551 w562]
                  tunnel: [w551 w560] -> w548
                  tunnel: [w552 w559] -> w547
                  tunnel: w546 -> [w552 w556]
                  tunnel: w545 -> [_ w555]
                  tunnel: w543 -> [w550 _]
                  frame 0, Default {
                    n163 = global write "Global 1.vi" "PLC8 error"(w550) -> ()
                  }
                  frame 1, 66 {
                    w554 = u8 1  # Slot S7 300/400
                    n164 = call <vilib>:"disconnect.vi"("error in (no error)"=w562, "S7 Connection in"=w556) -> ("error out"=w561:errorcluster)  [unwired: 8 in, 1 out]
                    n165 = call <vilib>:"Clear Errors.vi"("error in (no error)"=w561) -> ("error out"=w558:errorcluster)  [unwired: 5 in, 1 out]
                    n166 = call <vilib>:"connect.vi"("Use Rack/Slot for S71200/1500"=TRUE, "Slot S7 300/400"=w554, "PLC Type"=PLC_Type."S7 1200" ("PLC Type 2"), "error in (no error)"=w558, "IP address"=w555) -> ("error out"=w560:errorcluster, "S7 Connection out"=w559:T5)  [unwired: 5 in]
                  }
                }
              }
            }
            n167 = Unbundle By Name(w537) -> ("status"=w540:bool)
            n168 = Not(x=w540) -> (.not. x?=w539:bool)
            "PLC 8" <- w539
            n169 = global write "Global 1.vi" "PLC 8"(w539) -> ()
          }
        }
        n170 = call "PADMINI_STOP_ALL.vi"("Enum"=enum16{"Read", "Write"}."Read") -> ("Boolean 2"=w478:bool)  [unwired: 9 in, 1 out]
        n171 = local read "stop"() -> (w477:bool)
        n172 = Or(x=w477, y=w478) -> (x .or. y?=w476:bool)
        n173 = Wait (ms)(milliseconds to wait=u32 1200) -> ()  [unwired: 1 out]
      }
      n174 = call <vilib>:"Clear Errors.vi"("error in (no error)"=w455) -> ("error out"=w456:errorcluster)  [unwired: 5 in, 1 out]
      n175 = call <vilib>:"disconnect.vi"("error in (no error)"=w456, "S7 Connection in"=w454) -> ("error out"=w453:errorcluster)  [unwired: 8 in, 1 out]
    }
    frame Enabled {
      w566 = PLC_Comm_State."Int"  # Enum
      n176 = while {
        shift-right: [w578] -> _
        shift-left: w566 -> [w586]
        shift-right: [w570] -> w563
        shift-left: w564 -> [w585]
        shift-right: [w581] -> _
        shift-left: _ -> [w584]
        tunnel: w565 -> [w567]
        stop <- w579 stop-if-true
        w575 = PLC_Comm_State."Disconnect"  # Enum
        w583 = u32 800  # milliseconds to wait
        # "Int-->Write-->Read---if--Error-->reconnect\n               ^------v                                       v\n                ^------------------------------v"
        # "OP 110"
        n177 = case shown="\"Error\"" w586 {
          selector: w586 -> [w606 w623 w649 w690 w700 w704 _ _ _ _]
          tunnel: [w611 w625 w642 w676 w701 w709 w711 w714 w716 w718] -> w587
          tunnel: [w612 w624 w643 w677 w702 w706 w712 w713 w715 w717] -> w580
          tunnel: w585 -> [w609 w619 w640 w674 w698 w707 w711 w714 w716 w718]
          tunnel: w584 -> [w607 _ w641 w675 w702 w708 w712 w713 w715 w717]
          tunnel: [w605 w622 w648 w689 w699 w703 _ _ _ _] -> w582
          tunnel: [_ _ _ _ _ TRUE _ _ _ _] -> w579
          tunnel: [w606 w623 w649 w690 w700 w704 _ _ _ _] -> w576
          tunnel: w567 -> [w604 w621 _ _ _ _ _ _ _ _]
          frame "Connect" {
            w605 = PLC_Comm_State."Write"  # Enum
            w617 = TRUE  # Use Rack/Slot for S71200/1500
            w616 = u8 1  # Slot S7 300/400
            w614 = u8 0  # Rack S7 300/400
            # "Reconect"
            n178 = call <vilib>:"disconnect.vi"("error in (no error)"=w609, "S7 Connection in"=w607) -> ("error out"=w610:errorcluster)  [unwired: 8 in, 1 out]
            n179 = call <vilib>:"Clear Errors.vi"("error in (no error)"=w610) -> ("error out"=w608:errorcluster)  [unwired: 5 in, 1 out]
            n180 = call <vilib>:"connect.vi"("Use Rack/Slot for S71200/1500"=w617, "Slot S7 300/400"=w616, "PLC Type"=PLC_Type."S7 1200" ("PLC Type 2"), "error in (no error)"=w608, "Rack S7 300/400"=w614, "timeout [ms]"=1000 ("timeout [ms] 2"), "IP address"=w604) -> ("error out"=w611:errorcluster, "S7 Connection out"=w612:T5)  [unwired: 3 in]
          }
          frame "Int" {
            w622 = PLC_Comm_State."Write"  # Enum
            w626 = TRUE  # Use Rack/Slot for S71200/1500
            w627 = u8 1  # Slot S7 300/400
            w628 = u8 0  # Rack S7 300/400
            w629 = u16[] [7]  # Data Block #
            # "Initialize and set first bits"
            n181 = call "Stall Data Flow.vim"("value in"=w619, "milliseconds to wait"=u32 903) -> ("value out"=w618:errorcluster)  [unwired: 1 out]
            n182 = call <vilib>:"connect.vi"("Use Rack/Slot for S71200/1500"=w626, "Slot S7 300/400"=w627, "PLC Type"=PLC_Type."S7 1200" ("PLC Type 2"), "error in (no error)"=w618, "Rack S7 300/400"=w628, "timeout [ms]"=1000 ("timeout [ms] 2"), "IP address"=w621) -> ("error out"=w631:errorcluster, "S7 Connection out"=w630:T5)  [unwired: 3 in]
            n183 = for {
              tunnel: w629 -> [w639] mode=indexing
              shift-right: [w637] -> w624
              shift-left: w630 -> [w635]
              tunnel: w631 -> [w636]
              tunnel: [w634] -> w625
              w638 = i32[] [0, 0]  # DINT input array
              # "Reset Search and save \nbit on software start"
              n184 = call-poly <vilib>:"write DB.vi"("DINT input array"=w638, "error in (no error)"=w636, "Data Block #"=w639, "S7 Connection in"=w635) -> ("error out"=w634:errorcluster, "S7 Connection out"=w637:T5)  [unwired: 4 in, 2 out]
            }
          }
          frame "Write" {
            w648 = PLC_Comm_State."Read"  # Enum
            n185 = global read "DATA LOG.vi" "OP 110 Outputs"() -> (w647:bool)
            n186 = case shown="True" w647 {
              tunnel: [w659 w664] -> w646
              tunnel: [w660 w668] -> w645
              tunnel: w641 -> [w660 w662]
              tunnel: w640 -> [w659 w661]
              frame False {
              }
              frame True {
                w665 = i32[] [0, 0]  # DINT input array
                w666 = u16 7  # Data Block #
                n187 = call "PADMINI_AUTO_BARCODE_STATUS 110.vi"("Enum"=enum16{"Read", "Write"}."Read", "error in (no error)"=w661) -> ("error out"=w671:errorcluster, "O/P"=w672:i32[])  [unwired: 8 in]
                n188 = call-poly <vilib>:"write DB.vi"("Item offset [byte]"=u32 8, "DINT input array"=w672, "error in (no error)"=w671, "Data Block #"=w666, "S7 Connection in"=w662) -> ("error out"=w667:errorcluster, "S7 Connection out"=w669:T5)  [unwired: 3 in, 2 out]
                n189 = call-poly <vilib>:"write DB.vi"("DINT input array"=w665, "error in (no error)"=w667, "Data Block #"=w666, "S7 Connection in"=w669) -> ("error out"=w664:errorcluster, "S7 Connection out"=w668:T5)  [unwired: 4 in, 2 out]
                n190 = Unbundle By Name(w664) -> ("status"=w663:bool)
                n191 = global write "DATA LOG.vi" "OP 110 Outputs"(w663) -> ()
              }
            }
            n192 = global read "DATA LOG.vi" "OP 110 reset"() -> (w644:bool)
            n193 = case shown="True" w644 {
              tunnel: w646 -> [w650 w658]
              tunnel: [w650 w653] -> w642
              tunnel: w645 -> [w651 w657]
              tunnel: [w651 w656] -> w643
              frame False {
              }
              frame True {
                n194 = call-poly <vilib>:"write DB.vi"("DINT input array"=i32[] [0, 0], "error in (no error)"=w658, "Data Block #"=u16 7, "S7 Connection in"=w657) -> ("error out"=w653:errorcluster, "S7 Connection out"=w656:T5)  [unwired: 4 in, 2 out]
                n195 = Unbundle By Name(w653) -> ("status"=w652:bool)
                n196 = global write "DATA LOG.vi" "OP 110 reset"(w652) -> ()
              }
            }
          }
          frame "Read" {
            w689 = PLC_Comm_State."Write"  # Enum
            n197 = call-poly <vilib>:"read DB.vi"("Item offset [byte]"=u32 20, "String length reserved in DB (default=254)"=u16 50, "error in (no error)"=w674, "items #"=u16 3 ("Items # [byte]"), "Data Block #"=u16 7, "S7 Connection in"=w675) -> ("error out"=w687:errorcluster, "STRING result Array"=w688:string[], "S7 Connection out"=w684:T5)  [unwired: 2 in, 1 out]
            n198 = call-poly <vilib>:"read DB.vi"("error in (no error)"=w687, "items #"=u16 2 ("Items # [byte]"), "Data Block #"=u16 7, "S7 Connection in"=w684) -> ("error out"=w686:errorcluster, "DINT result array"=w685:i32[], "S7 Connection out"=w677:T5)  [unwired: 5 in]
            n199 = case shown="Error" w686 {
              selector: w686 -> [w695 w697]
              tunnel: w685 -> [w696 _]
              tunnel: w688 -> [w692 _]
              tunnel: [w691 w697] -> w676
              frame No Error {
                w693 = enum16{"Read", "Write"}."Write" ("Enum")
                n200 = call "PADMINI_AUTO_BARCODE_STRING 110.vi"("Enum"=w693, "error in (no error)"=w695, "Input"=w692) -> ("error out"=w694:errorcluster)  [unwired: 7 in, 1 out]
                n201 = call "PADMINI_AUTO_CYCLE STATE 110.vi"("Enum"=w693, "error in (no error)"=w694, "Input"=w696) -> ("error out"=w691:errorcluster)  [unwired: 7 in, 1 out]
              }
              frame Error {
              }
            }
          }
          frame "Error" {
            w699 = PLC_Comm_State."Write"  # Enum
            n202 = global write "Global 1.vi" "PLC8 error"(w698) -> ()
            n203 = call <vilib>:"Clear Errors.vi"("error in (no error)"=w698) -> ("error out"=w701:errorcluster)  [unwired: 5 in, 1 out]
          }
          frame "Disconnect" {
            w703 = PLC_Comm_State."Disconnect"  # Enum
            w706 = T5 {"TCP Connection Ref"=refnum, "IP address"="", "timeout ms"=5000, "Connected?"=FALSE, "PLC Type"=enum."S7 1200", "Rack S7 400"=0, "Slot S7 400"=0, "PDU Size"=0, "connection semaphore"=refnum}  # S7 Connection out
            n204 = call <vilib>:"Clear Errors.vi"("error in (no error)"=w707) -> ("error out"=w710:errorcluster)  [unwired: 5 in, 1 out]
            n205 = call <vilib>:"disconnect.vi"("error in (no error)"=w710, "S7 Connection in"=w708) -> ("error out"=w709:errorcluster)  [unwired: 8 in, 1 out]
          }
          frame "Write2" {
            # "No Use"
          }
          frame "Write3" {
            # "No Use"
          }
          frame "Read2" {
            # "No Use"
          }
          frame "Read3" {
            # "No Use"
          }
        }
        n206 = Wait (ms)(milliseconds to wait=w583) -> ()  [unwired: 1 out]
        n207 = call "PADMINI_STOP_ALL.vi"("Enum"=enum16{"Read", "Write"}."Read") -> ("Boolean 2"=w574:bool)  [unwired: 9 in, 1 out]
        n208 = local read "stop"() -> (w569:bool)
        n209 = case shown="Error" w587 {
          selector: w587 -> [w590 w591]
          tunnel: [w590 w597] -> w570
          tunnel: [w589 w593] -> w577
          tunnel: w582 -> [w589 _]
          tunnel: [w588 w603] -> w581
          tunnel: w580 -> [w588 w603]
          tunnel: w576 -> [_ w601]
          frame No Error {
          }
          frame Error {
            w594 = PLC_Comm_State."Connect"  # Enum
            w592 = PLC_Comm_State."Error"  # Enum
            n210 = Unbundle By Name(w591) -> ("source"=w602:string)
            n211 = call <userlib>:"Get Strings from Enum__ogtk.vi"("Enum"=w601) -> ("String Value"=w600:string)  [unwired: 7 in, 3 out]
            n212 = Concatenate Strings(w600, "    " ("string"), w602) -> (w598:string)
            n213 = Bundle By Name(cluster=w591, "source"=w598) -> (w597:errorcluster)
            n214 = call <vilib>:"Clear Errors.vi"("error in (no error)"=w591, "specific error code to clear (0: all)"=6002) -> ("specific error cleared?"=w596:bool)  [unwired: 4 in, 1 out]
            n215 = Select(t=w594, s=w596, f=w592) -> (s? t:f=w593:T1)
          }
        }
        n216 = Or(x=w569, y=w574) -> (x .or. y?=w572:bool)
        n217 = Select(t=w575, s=w572, f=w577) -> (s? t:f=w578:T1)
        n218 = Unbundle By Name(w570) -> ("status"=w571:bool)
        n219 = Not(x=w571) -> (.not. x?=w568:bool)
        n220 = global write "Global 1.vi" "PLC 8"(w568) -> ()
      }
    }
  }
  n221 = disable-structure shown="Enabled" {
    disable-tunnel: w30 -> [w730 w944]
    disable-tunnel: w9 -> [w724 w943]
    disable-tunnel: [w719 w941] -> w5
    frame Disabled {
      w721 = TRUE  # Use Rack/Slot for S71200/1500
      w722 = u8 1  # Slot S7 300/400
      w723 = u8 0  # Rack S7 300/400
      n222 = call <vilib>:"connect.vi"("Use Rack/Slot for S71200/1500"=w721, "Slot S7 300/400"=w722, "PLC Type"=PLC_Type."S7 1200" ("PLC Type 2"), "error in (no error)"=w724, "Rack S7 300/400"=w723, "timeout [ms]"=1000 ("timeout [ms] 2"), "IP address"=w730) -> ("error out"=w725:errorcluster, "S7 Connection out"=w726:T5)  [unwired: 3 in]
      n223 = for {
        tunnel: u16[] [80, 82] ("Data Block #") -> [w740] mode=indexing
        shift-right: [w738] -> w727
        shift-left: w726 -> [w735]
        tunnel: w725 -> [w736]
        tunnel: [w737] -> w728
        w739 = i32[] [0, 0]  # DINT input array
        # "Reset Search and save \nbit on software start"
        n224 = call-poly <vilib>:"write DB.vi"("DINT input array"=w739, "error in (no error)"=w736, "Data Block #"=w740, "S7 Connection in"=w735) -> ("error out"=w737:errorcluster, "S7 Connection out"=w738:T5)  [unwired: 4 in, 2 out]
      }
      n225 = while {
        shift-right: [w743] -> w731
        shift-left: w727 -> [w753]
        shift-right: [w751] -> w732
        shift-left: w728 -> [w752]
        tunnel: w730 -> [w742]
        stop <- w745 stop-if-true
        # "OP 70 - 80"
        n226 = flat-sequence {
          tunnel: [w755] -> w749
          tunnel: [w759] -> w744
          tunnel: w752 -> [w861]
          tunnel: w753 -> [w860]
          tunnel: w742 -> [w848]
          tunnel: [w848] -> w741
          tunnel: [w914] -> w751
          tunnel: [w913] -> w743
          tunnel: w749 -> [w916]
          tunnel: w744 -> [w915]
          tunnel: w741 -> [w912]
          frame #0 {
            w780 = u32 500  # milliseconds to wait
            w807 = u16 83 ("Data Block #")
            w830 = u16 81 ("Data Block #")
            w791 = u16 82 ("Data Block #")
            w767 = u16 80 ("Data Block #")
            # "AUTO WRITE"
            n227 = global read "DATA LOG.vi" "OP 70 Outputs"() -> (w859:bool)
            n228 = case shown="True" w859 {
              tunnel: w860 -> [w897 w910]
              tunnel: [w898 w901] -> w835
              tunnel: [w897 w902] -> w834
              tunnel: w861 -> [w898 w907]
              frame False {
              }
              frame True {
                w911 = u16 81  # Data Block #
                n229 = call "PADMINI_AUTO_BARCODE_STATUS 70.vi"("Enum"=enum16{"Read", "Write"}."Read", "error in (no error)"=w907) -> ("error out"=w906:errorcluster, "O/P"=w908:i32[])  [unwired: 8 in]
                n230 = global write "DATA LOG.vi" "OP 70 Outputs"(FALSE) -> ()
                n231 = call-poly <vilib>:"write DB.vi"("DINT input array"=w908, "error in (no error)"=w906, "Data Block #"=w911, "S7 Connection in"=w910) -> ("error out"=w899:errorcluster, "S7 Connection out"=w900:T5)  [unwired: 4 in, 2 out]
                n232 = call-poly <vilib>:"write DB.vi"("DINT input array"=i32[] [0] ("Data Byte"), "error in (no error)"=w899, "Data Block #"=u16 80, "S7 Connection in"=w900) -> ("error out"=w901:errorcluster, "S7 Connection out"=w902:T5)  [unwired: 4 in, 2 out]
              }
            }
            n233 = global read "DATA LOG.vi" "OP 70 reset"() -> (w836:bool)
            n234 = global read "DATA LOG.vi" "Auto Cycle On"() -> (w784:bool)
            n235 = case shown="True" w836 {
              tunnel: w835 -> [w872 w881]
              tunnel: [w872 w880] -> w825
              tunnel: w834 -> [w873 w879]
              tunnel: [w873 w878] -> w826
              frame False {
              }
              frame True {
                n236 = global write "DATA LOG.vi" "OP 70 reset"(FALSE) -> ()
                n237 = call-poly <vilib>:"write DB.vi"("Item offset [byte]"=u16 4 ("Data Block #"), "DINT input array"=i32[] [0], "error in (no error)"=w881, "Data Block #"=u16 80, "S7 Connection in"=w879) -> ("error out"=w880:errorcluster, "S7 Connection out"=w878:T5)  [unwired: 3 in, 2 out]
              }
            }
            n238 = Boolean To (0,1)(Boolean=w784) -> (0, 1=w783:i16)
            n239 = Build Array(w783) -> (w782:i16[])
            n240 = call "Stall Data Flow.vim"("value in"=w825, "milliseconds to wait"=w780) -> ("value out"=w781:errorcluster)  [unwired: 1 out]
            n241 = global read "Global 1.vi" "Filtered BARCODE selected"() -> (w827:string[])
            n242 = call-poly <vilib>:"write DB.vi"("Item offset [byte]"=u32 20, "DINT input array"=w782, "error in (no error)"=w781, "Data Block #"=w830, "S7 Connection in"=w826) -> ("error out"=w832:errorcluster, "S7 Connection out"=w833:T5)  [unwired: 3 in, 2 out]
            n243 = call-poly <vilib>:"write DB.vi"("Item offset [byte]"=u32 24, "Input STRINGS"=w827, "error in (no error)"=w832, "String length reserved in DB (default=254)"=u16 15, "Data Block #"=w830, "S7 Connection in"=w833) -> ("error out"=w823:errorcluster, "S7 Connection out"=w824:T5)  [unwired: 2 in, 2 out]
            n244 = call "Stall Data Flow.vim"("value in"=w823, "milliseconds to wait"=u32 300) -> ("value out"=w779:errorcluster)  [unwired: 1 out]
            n245 = call-poly <vilib>:"read DB.vi"("Item offset [byte]"=u32 8, "error in (no error)"=w779, "items #"=u16 2 ("Items # [byte]"), "Data Block #"=w767, "S7 Connection in"=w824) -> ("error out"=w851:errorcluster, "REAL result array"=w849:sgl[], "S7 Connection out"=w857:T5)  [unwired: 4 in]
            n246 = call "PADMINI_AUTO_CYCLE VALUE 70.vi"("Enum"=enum16{"Read", "Write"}."Write", "error in (no error)"=w851, "Input"=w849) -> ("error out"=w850:errorcluster)  [unwired: 7 in, 1 out]
            n247 = call "Stall Data Flow.vim"("value in"=w850, "milliseconds to wait"=u32 0) -> ("value out"=w777:errorcluster)  [unwired: 1 out]
            n248 = call-poly <vilib>:"read DB.vi"("Item offset [byte]"=u32 16, "String length reserved in DB (default=254)"=u16 50, "error in (no error)"=w777, "items #"=u16 1 ("Items # [byte]"), "Data Block #"=w767, "S7 Connection in"=w857) -> ("error out"=w816:errorcluster, "STRING result Array"=w815:string[], "S7 Connection out"=w817:T5)  [unwired: 2 in, 1 out]
            n249 = call-poly <vilib>:"read DB.vi"("Item offset [byte]"=u32 68, "String length reserved in DB (default=254)"=u16 10, "error in (no error)"=w816, "items #"=u16 1 ("Items # [byte]"), "Data Block #"=w767, "S7 Connection in"=w817) -> ("error out"=w818:errorcluster, "STRING result Array"=w819:string[], "S7 Connection out"=w766:T5)  [unwired: 2 in, 1 out]
            n250 = Build Array (concatenate)(w815, w819) -> (w813:string[])
            n251 = call "PADMINI_AUTO_BARCODE_STRING 70.vi"("Enum"=enum16{"Read", "Write"}."Write", "error in (no error)"=w818, "Input"=w813) -> ("error out"=w764:errorcluster)  [unwired: 7 in, 1 out]
            n252 = call-poly <vilib>:"read DB.vi"("error in (no error)"=w764, "items #"=u16 2 ("Items # [byte]"), "Data Block #"=w767, "S7 Connection in"=w766) -> ("error out"=w769:errorcluster, "DINT result array"=w771:i32[], "S7 Connection out"=w765:T5)  [unwired: 5 in]
            n253 = call "PADMINI_AUTO_CYCLE STATE 70.vi"("Enum"=enum16{"Read", "Write"}."Write", "error in (no error)"=w769, "Input"=w771) -> ("error out"=w754:errorcluster)  [unwired: 7 in, 1 out]
            n254 = global read "DATA LOG.vi" "OP 80 Outputs"() -> (w837:bool)
            n255 = case shown="True" w837 {
              tunnel: [w883 w886] -> w812
              tunnel: [w882 w887] -> w789
              tunnel: w754 -> [w883 w893]
              tunnel: w765 -> [w882 w890]
              frame False {
              }
              frame True {
                w896 = u16 83  # Data Block #
                n256 = call "PADMINI_AUTO_BARCODE_STATUS 80.vi"("Enum"=enum16{"Read", "Write"}."Read", "error in (no error)"=w893) -> ("error out"=w892:errorcluster, "O/P"=w894:i32[])  [unwired: 8 in]
                n257 = global write "DATA LOG.vi" "OP 80 Outputs"(FALSE) -> ()
                n258 = call-poly <vilib>:"write DB.vi"("DINT input array"=w894, "error in (no error)"=w892, "Data Block #"=w896, "S7 Connection in"=w890) -> ("error out"=w884:errorcluster, "S7 Connection out"=w885:T5)  [unwired: 4 in, 2 out]
                n259 = call-poly <vilib>:"write DB.vi"("DINT input array"=i32[] [0] ("Data Byte"), "error in (no error)"=w884, "Data Block #"=u16 82, "S7 Connection in"=w885) -> ("error out"=w886:errorcluster, "S7 Connection out"=w887:T5)  [unwired: 4 in, 2 out]
              }
            }
            n260 = global read "DATA LOG.vi" "OP 80 reset"() -> (w811:bool)
            n261 = global read "DATA LOG.vi" "Auto Cycle On"() -> (w787:bool)
            n262 = case shown="True" w811 {
              tunnel: w812 -> [w863 w871]
              tunnel: [w863 w866] -> _
              tunnel: [w863 w866] -> w801
              tunnel: w789 -> [w862 w865]
              tunnel: [w862 w864] -> w788
              frame False {
              }
              frame True {
                n263 = global write "DATA LOG.vi" "OP 80 reset"(FALSE) -> ()
                n264 = call-poly <vilib>:"write DB.vi"("Item offset [byte]"=u16 4 ("Data Block #"), "DINT input array"=i32[] [0], "error in (no error)"=w871, "Data Block #"=u16 82, "S7 Connection in"=w865) -> ("error out"=w866:errorcluster, "S7 Connection out"=w864:T5)  [unwired: 3 in, 2 out]
              }
            }
            n265 = Boolean To (0,1)(Boolean=w787) -> (0, 1=w786:i16)
            n266 = Build Array(w786) -> (w785:i16[])
            n267 = global read "Global 1.vi" "Filtered BARCODE selected"() -> (w804:string[])
            n268 = call-poly <vilib>:"write DB.vi"("Item offset [byte]"=u32 20, "DINT input array"=w785, "error in (no error)"=w801, "Data Block #"=w807, "S7 Connection in"=w788) -> ("error out"=w809:errorcluster, "S7 Connection out"=w810:T5)  [unwired: 3 in, 2 out]
            n269 = call-poly <vilib>:"write DB.vi"("Item offset [byte]"=u32 24, "Input STRINGS"=w804, "error in (no error)"=w809, "String length reserved in DB (default=254)"=u16 15, "Data Block #"=w807, "S7 Connection in"=w810) -> ("error out"=w802:errorcluster, "S7 Connection out"=w803:T5)  [unwired: 2 in, 2 out]
            n270 = call-poly <vilib>:"read DB.vi"("Item offset [byte]"=u32 8, "error in (no error)"=w802, "items #"=u16 1 ("Items # [byte]"), "Data Block #"=w791, "S7 Connection in"=w803) -> ("error out"=w845:errorcluster, "REAL result array"=w847:sgl[], "S7 Connection out"=w839:T5)  [unwired: 4 in]
            n271 = call "PADMINI_AUTO_CYCLE VALUE 80.vi"("Enum"=enum16{"Read", "Write"}."Write", "error in (no error)"=w845, "Input"=w847) -> ("error out"=w846:errorcluster)  [unwired: 7 in, 1 out]
            n272 = call "Stall Data Flow.vim"("value in"=w846, "milliseconds to wait"=u32 300) -> ("value out"=w775:errorcluster)  [unwired: 1 out]
            n273 = call-poly <vilib>:"read DB.vi"("Item offset [byte]"=u32 12, "String length reserved in DB (default=254)"=u16 50, "error in (no error)"=w775, "items #"=u16 1 ("Items # [byte]"), "Data Block #"=w791, "S7 Connection in"=w839) -> ("error out"=w796:errorcluster, "STRING result Array"=w794:string[], "S7 Connection out"=w792:T5)  [unwired: 2 in, 1 out]
            n274 = call "Stall Data Flow.vim"("value in"=w796, "milliseconds to wait"=u32 300) -> ("value out"=w773:errorcluster)  [unwired: 1 out]
            n275 = call-poly <vilib>:"read DB.vi"("Item offset [byte]"=u32 64, "String length reserved in DB (default=254)"=u16 10, "error in (no error)"=w773, "items #"=u16 2 ("Items # [byte]"), "Data Block #"=w791, "S7 Connection in"=w792) -> ("error out"=w795:errorcluster, "STRING result Array"=w800:string[], "S7 Connection out"=w756:T5)  [unwired: 2 in, 1 out]
            n276 = Build Array (concatenate)(w794, w800) -> (w793:string[])
            n277 = call "PADMINI_AUTO_BARCODE_STRING 80.vi"("Enum"=enum16{"Read", "Write"}."Write", "error in (no error)"=w795, "Input"=w793) -> ("error out"=w758:errorcluster)  [unwired: 7 in, 1 out]
            n278 = call-poly <vilib>:"read DB.vi"("error in (no error)"=w758, "items #"=u16 2 ("Items # [byte]"), "Data Block #"=u16 82, "S7 Connection in"=w756) -> ("error out"=w762:errorcluster, "DINT result array"=w760:i32[], "S7 Connection out"=w755:T5)  [unwired: 5 in]
            n279 = call "PADMINI_AUTO_CYCLE STATE 80.vi"("Enum"=enum16{"Read", "Write"}."Write", "error in (no error)"=w762, "Input"=w760) -> ("error out"=w759:errorcluster)  [unwired: 7 in, 1 out]
          }
          frame #1 {
            # "RECONNECT"
            n280 = case shown="Error" w915 {
              selector: w915 -> [w920 w921]
              tunnel: [w919 w925] -> w913
              tunnel: [w920 w926] -> w914
              tunnel: w916 -> [w919 w924]
              tunnel: w912 -> [_ w923]
              frame No Error {
              }
              frame Error {
                n281 = Unbundle By Name(w921) -> ("code"=w922:i32)
                n282 = call <vilib>:"Clear Errors.vi"("error in (no error)"=w921) -> ("error out"=w927:errorcluster)  [unwired: 5 in, 1 out]
                n283 = case shown="1, 66" w922 {
                  tunnel: w927 -> [w929 w940]
                  tunnel: [w929 w938] -> w926
                  tunnel: [w930 w937] -> w925
                  tunnel: w924 -> [w930 w934]
                  tunnel: w923 -> [_ w933]
                  tunnel: w921 -> [w928 _]
                  frame 0, Default {
                    n284 = global write "Global 1.vi" "PLC6 error"(w928) -> ()
                  }
                  frame 1, 66 {
                    n285 = call <vilib>:"disconnect.vi"("error in (no error)"=w940, "S7 Connection in"=w934) -> ("error out"=w939:errorcluster)  [unwired: 8 in, 1 out]
                    n286 = call <vilib>:"Clear Errors.vi"("error in (no error)"=w939) -> ("error out"=w936:errorcluster)  [unwired: 5 in, 1 out]
                    n287 = call <vilib>:"connect.vi"("Use Rack/Slot for S71200/1500"=TRUE, "Slot S7 300/400"=u8 1, "PLC Type"=PLC_Type."S7 1200" ("PLC Type 2"), "error in (no error)"=w936, "IP address"=w933) -> ("error out"=w938:errorcluster, "S7 Connection out"=w937:T5)  [unwired: 5 in]
                  }
                }
              }
            }
            n288 = Unbundle By Name(w915) -> ("status"=w918:bool)
            n289 = Not(x=w918) -> (.not. x?=w917:bool)
            "PLC 6" <- w917
            n290 = global write "Global 1.vi" "PLC 6"(w917) -> ()
          }
        }
        n291 = call "PADMINI_STOP_ALL.vi"("Enum"=enum16{"Read", "Write"}."Read") -> ("Boolean 2"=w747:bool)  [unwired: 9 in, 1 out]
        n292 = local read "stop"() -> (w746:bool)
        n293 = Or(x=w746, y=w747) -> (x .or. y?=w745:bool)
        n294 = Wait (ms)(milliseconds to wait=u32 1000) -> ()  [unwired: 1 out]
      }
      n295 = call <vilib>:"Clear Errors.vi"("error in (no error)"=w732) -> ("error out"=w720:errorcluster)  [unwired: 5 in, 1 out]
      n296 = call <vilib>:"disconnect.vi"("error in (no error)"=w720, "S7 Connection in"=w731) -> ("error out"=w719:errorcluster)  [unwired: 8 in, 1 out]
    }
    frame Enabled {
      w942 = PLC_Comm_State."Int"  # Enum
      n297 = while {
        shift-right: [w956] -> _
        shift-left: w942 -> [w964]
        shift-right: [w948] -> w941
        shift-left: w943 -> [w963]
        shift-right: [w959] -> _
        shift-left: _ -> [w962]
        tunnel: w944 -> [w945]
        stop <- w957 stop-if-true
        w953 = PLC_Comm_State."Disconnect"  # Enum
        w961 = u32 800  # milliseconds to wait
        # "Int-->Write-->Read---if--Error-->reconnect\n               ^------v                                       v\n                ^------------------------------v"
        # "OP 70-80"
        n298 = case shown="\"Error\"" w964 {
          selector: w964 -> [w984 w1002 w1039 w1091 w1145 w1182 w1195 w1199 _ _]
          tunnel: [w989 w1004 w1019 w1073 w1119 w1158 w1196 w1204 w1207 w1209] -> w965
          tunnel: [w990 w1003 w1018 w1074 w1118 w1157 w1197 w1201 w1206 w1208] -> w958
          tunnel: w963 -> [w987 w998 w1020 w1072 w1120 w1155 w1193 w1202 w1207 w1209]
          tunnel: w962 -> [w985 _ w1021 w1071 w1121 w1156 w1197 w1203 w1206 w1208]
          tunnel: [w983 w1001 w1038 w1092 w1144 w1183 w1194 w1198 _ _] -> w960
          tunnel: [_ _ _ _ _ _ _ TRUE _ _] -> w957
          tunnel: [w984 w1002 w1039 w1091 w1145 w1182 w1195 w1199 _ _] -> w954
          tunnel: w945 -> [w982 w1000 _ _ _ _ _ _ _ _]
          frame "Connect" {
            w983 = PLC_Comm_State."Write"  # Enum
            w995 = TRUE  # Use Rack/Slot for S71200/1500
            w994 = u8 1  # Slot S7 300/400
            w992 = u8 0  # Rack S7 300/400
            # "Reconect"
            n299 = call <vilib>:"disconnect.vi"("error in (no error)"=w987, "S7 Connection in"=w985) -> ("error out"=w988:errorcluster)  [unwired: 8 in, 1 out]
            n300 = call <vilib>:"Clear Errors.vi"("error in (no error)"=w988) -> ("error out"=w986:errorcluster)  [unwired: 5 in, 1 out]
            n301 = call <vilib>:"connect.vi"("Use Rack/Slot for S71200/1500"=w995, "Slot S7 300/400"=w994, "PLC Type"=PLC_Type."S7 1200" ("PLC Type 2"), "error in (no error)"=w986, "Rack S7 300/400"=w992, "timeout [ms]"=1000 ("timeout [ms] 2"), "IP address"=w982) -> ("error out"=w989:errorcluster, "S7 Connection out"=w990:T5)  [unwired: 3 in]
          }
          frame "Int" {
            w1001 = PLC_Comm_State."Write"  # Enum
            w1005 = TRUE  # Use Rack/Slot for S71200/1500
            w1006 = u8 1  # Slot S7 300/400
            w1007 = u8 0  # Rack S7 300/400
            # "Initialize and set first bits"
            n302 = call "Stall Data Flow.vim"("value in"=w998, "milliseconds to wait"=u32 645) -> ("value out"=w997:errorcluster)  [unwired: 1 out]
            n303 = call <vilib>:"connect.vi"("Use Rack/Slot for S71200/1500"=w1005, "Slot S7 300/400"=w1006, "PLC Type"=PLC_Type."S7 1200" ("PLC Type 2"), "error in (no error)"=w997, "Rack S7 300/400"=w1007, "timeout [ms]"=1000 ("timeout [ms] 2"), "IP address"=w1000) -> ("error out"=w1009:errorcluster, "S7 Connection out"=w1008:T5)  [unwired: 3 in]
            n304 = for {
              tunnel: u16[] [80, 82] ("Data Block #") -> [w1017] mode=indexing
              shift-right: [w1015] -> w1003
              shift-left: w1008 -> [w1013]
              tunnel: w1009 -> [w1014]
              tunnel: [w1012] -> w1004
              w1016 = i32[] [0, 0]  # DINT input array
              # "Reset Search and save \nbit on software start"
              n305 = call-poly <vilib>:"write DB.vi"("DINT input array"=w1016, "error in (no error)"=w1014, "Data Block #"=w1017, "S7 Connection in"=w1013) -> ("error out"=w1012:errorcluster, "S7 Connection out"=w1015:T5)  [unwired: 4 in, 2 out]
            }
          }
          frame "Write" {
            w1023 = u16 81 ("Data Block #")
            w1038 = PLC_Comm_State."Write2"  # Enum
            # "OP 70 Write"
            n306 = global read "DATA LOG.vi" "OP 70 Outputs"() -> (w1037:bool)
            n307 = case shown="True" w1037 {
              tunnel: w1021 -> [w1053 w1066]
              tunnel: [w1054 w1055] -> w1035
              tunnel: [w1053 w1059] -> w1034
              tunnel: w1020 -> [w1054 w1063]
              frame False {
              }
              frame True {
                w1067 = u16 81  # Data Block #
                n308 = call "PADMINI_AUTO_BARCODE_STATUS 70.vi"("Enum"=enum16{"Read", "Write"}."Read", "error in (no error)"=w1063) -> ("error out"=w1062:errorcluster, "O/P"=w1064:i32[])  [unwired: 8 in]
                n309 = call-poly <vilib>:"write DB.vi"("DINT input array"=w1064, "error in (no error)"=w1062, "Data Block #"=w1067, "S7 Connection in"=w1066) -> ("error out"=w1057:errorcluster, "S7 Connection out"=w1058:T5)  [unwired: 4 in, 2 out]
                n310 = call-poly <vilib>:"write DB.vi"("DINT input array"=i32[] [0] ("Data Byte"), "error in (no error)"=w1057, "Data Block #"=u16 80, "S7 Connection in"=w1058) -> ("error out"=w1056:errorcluster, "S7 Connection out"=w1059:T5)  [unwired: 4 in, 2 out]
                n311 = case shown="No Error" w1056 {
                  selector: w1056 -> [w1068 w1070]
                  tunnel: [w1068 w1070] -> w1055
                  frame No Error {
                    n312 = global write "DATA LOG.vi" "OP 70 Outputs"(FALSE) -> ()
                  }
                  frame Error {
                  }
                }
              }
            }
            n313 = global read "DATA LOG.vi" "OP 70 reset"() -> (w1036:bool)
            n314 = global read "DATA LOG.vi" "Auto Cycle On"() -> (w1028:bool)
            n315 = case shown="True" w1036 {
              tunnel: w1035 -> [w1040 w1049]
              tunnel: [w1040 w1042] -> w1029
              tunnel: w1034 -> [w1041 w1048]
              tunnel: [w1041 w1047] -> w1030
              frame False {
              }
              frame True {
                n316 = call-poly <vilib>:"write DB.vi"("Item offset [byte]"=u16 4 ("Data Block #"), "DINT input array"=i32[] [0], "error in (no error)"=w1049, "Data Block #"=u16 80, "S7 Connection in"=w1048) -> ("error out"=w1043:errorcluster, "S7 Connection out"=w1047:T5)  [unwired: 3 in, 2 out]
                n317 = case shown="No Error" w1043 {
                  selector: w1043 -> [w1050 w1052]
                  tunnel: [w1050 w1052] -> w1042
                  frame No Error {
                    n318 = global write "DATA LOG.vi" "OP 70 reset"(FALSE) -> ()
                  }
                  frame Error {
                  }
                }
              }
            }
            n319 = Boolean To (0,1)(Boolean=w1028) -> (0, 1=w1027:i16)
            n320 = Build Array(w1027) -> (w1026:i16[])
            n321 = global read "Global 1.vi" "Filtered BARCODE selected"() -> (w1031:string[])
            n322 = call-poly <vilib>:"write DB.vi"("Item offset [byte]"=u32 20, "DINT input array"=w1026, "error in (no error)"=w1029, "Data Block #"=w1023, "S7 Connection in"=w1030) -> ("error out"=w1032:errorcluster, "S7 Connection out"=w1033:T5)  [unwired: 3 in, 2 out]
            n323 = call-poly <vilib>:"write DB.vi"("Item offset [byte]"=u32 24, "Input STRINGS"=w1031, "error in (no error)"=w1032, "String length reserved in DB (default=254)"=u16 15, "Data Block #"=w1023, "S7 Connection in"=w1033) -> ("error out"=w1019:errorcluster, "S7 Connection out"=w1018:T5)  [unwired: 2 in, 2 out]
          }
          frame "Write2" {
            w1076 = u16 83 ("Data Block #")
            w1092 = PLC_Comm_State."Read"  # Enum
            # "op 80 wirte 2"
            n324 = global read "DATA LOG.vi" "OP 80 Outputs"() -> (w1090:bool)
            n325 = case shown="True" w1090 {
              tunnel: [w1104 w1106] -> w1089
              tunnel: [w1103 w1109] -> w1083
              tunnel: w1072 -> [w1104 w1114]
              tunnel: w1071 -> [w1103 w1112]
              frame False {
              }
              frame True {
                w1117 = u16 83  # Data Block #
                n326 = call "PADMINI_AUTO_BARCODE_STATUS 80.vi"("Enum"=enum16{"Read", "Write"}."Read", "error in (no error)"=w1114) -> ("error out"=w1113:errorcluster, "O/P"=w1115:i32[])  [unwired: 8 in]
                n327 = call-poly <vilib>:"write DB.vi"("DINT input array"=w1115, "error in (no error)"=w1113, "Data Block #"=w1117, "S7 Connection in"=w1112) -> ("error out"=w1107:errorcluster, "S7 Connection out"=w1108:T5)  [unwired: 4 in, 2 out]
                n328 = call-poly <vilib>:"write DB.vi"("DINT input array"=i32[] [0] ("Data Byte"), "error in (no error)"=w1107, "Data Block #"=u16 82, "S7 Connection in"=w1108) -> ("error out"=w1106:errorcluster, "S7 Connection out"=w1109:T5)  [unwired: 4 in, 2 out]
                n329 = Unbundle By Name(w1106) -> ("status"=w1105:bool)
                n330 = global write "DATA LOG.vi" "OP 80 Outputs"(w1105) -> ()
              }
            }
            n331 = global read "DATA LOG.vi" "OP 80 reset"() -> (w1088:bool)
            n332 = case shown="True" w1088 {
              tunnel: w1089 -> [w1094 w1102]
              tunnel: [w1094 w1096] -> _
              tunnel: [w1094 w1096] -> w1084
              tunnel: w1083 -> [w1093 w1098]
              tunnel: [w1093 w1097] -> w1082
              frame False {
              }
              frame True {
                n333 = call-poly <vilib>:"write DB.vi"("Item offset [byte]"=u16 4 ("Data Block #"), "DINT input array"=i32[] [0], "error in (no error)"=w1102, "Data Block #"=u16 82, "S7 Connection in"=w1098) -> ("error out"=w1096:errorcluster, "S7 Connection out"=w1097:T5)  [unwired: 3 in, 2 out]
                n334 = Unbundle By Name(w1096) -> ("status"=w1095:bool)
                n335 = global write "DATA LOG.vi" "OP 80 reset"(w1095) -> ()
              }
            }
            n336 = global read "DATA LOG.vi" "Auto Cycle On"() -> (w1081:bool)
            n337 = Boolean To (0,1)(Boolean=w1081) -> (0, 1=w1080:i16)
            n338 = Build Array(w1080) -> (w1079:i16[])
            n339 = global read "Global 1.vi" "Filtered BARCODE selected"() -> (w1085:string[])
            n340 = call-poly <vilib>:"write DB.vi"("Item offset [byte]"=u32 20, "DINT input array"=w1079, "error in (no error)"=w1084, "Data Block #"=w1076, "S7 Connection in"=w1082) -> ("error out"=w1086:errorcluster, "S7 Connection out"=w1087:T5)  [unwired: 3 in, 2 out]
            n341 = call-poly <vilib>:"write DB.vi"("Item offset [byte]"=u32 24, "Input STRINGS"=w1085, "error in (no error)"=w1086, "String length reserved in DB (default=254)"=u16 15, "Data Block #"=w1076, "S7 Connection in"=w1087) -> ("error out"=w1073:errorcluster, "S7 Connection out"=w1074:T5)  [unwired: 2 in, 2 out]
          }
          frame "Read" {
            w1130 = u16 80 ("Data Block #")
            w1144 = PLC_Comm_State."Read2"  # Enum
            # "OP70 read"
            n342 = call-poly <vilib>:"read DB.vi"("Item offset [byte]"=u32 8, "error in (no error)"=w1120, "items #"=u16 2 ("Items # [byte]"), "Data Block #"=w1130, "S7 Connection in"=w1121) -> ("error out"=w1140:errorcluster, "REAL result array"=w1143:sgl[], "S7 Connection out"=w1141:T5)  [unwired: 4 in]
            n343 = call-poly <vilib>:"read DB.vi"("Item offset [byte]"=u32 16, "String length reserved in DB (default=254)"=u16 50, "error in (no error)"=w1140, "items #"=u16 1 ("Items # [byte]"), "Data Block #"=w1130, "S7 Connection in"=w1141) -> ("error out"=w1136:errorcluster, "STRING result Array"=w1135:string[], "S7 Connection out"=w1137:T5)  [unwired: 2 in, 1 out]
            n344 = call-poly <vilib>:"read DB.vi"("Item offset [byte]"=u32 68, "String length reserved in DB (default=254)"=u16 10, "error in (no error)"=w1136, "items #"=u16 1 ("Items # [byte]"), "Data Block #"=w1130, "S7 Connection in"=w1137) -> ("error out"=w1138:errorcluster, "STRING result Array"=w1139:string[], "S7 Connection out"=w1132:T5)  [unwired: 2 in, 1 out]
            n345 = Build Array (concatenate)(w1135, w1139) -> (w1142:string[])
            n346 = call-poly <vilib>:"read DB.vi"("error in (no error)"=w1138, "items #"=u16 2 ("Items # [byte]"), "Data Block #"=w1130, "S7 Connection in"=w1132) -> ("error out"=w1133:errorcluster, "DINT result array"=w1134:i32[], "S7 Connection out"=w1118:T5)  [unwired: 5 in]
            n347 = case shown="No Error" w1133 {
              selector: w1133 -> [w1148 w1154]
              tunnel: w1134 -> [w1153 _]
              tunnel: w1142 -> [w1152 _]
              tunnel: w1143 -> [w1149 _]
              tunnel: [w1147 w1154] -> w1119
              frame No Error {
                w1151 = enum16{"Read", "Write"}."Write" ("Enum")
                n348 = call "PADMINI_AUTO_BARCODE_STRING 70.vi"("Enum"=w1151, "error in (no error)"=w1148, "Input"=w1152) -> ("error out"=w1150:errorcluster)  [unwired: 7 in, 1 out]
                n349 = call "PADMINI_AUTO_CYCLE VALUE 70.vi"("Enum"=w1151, "error in (no error)"=w1150, "Input"=w1149) -> ("error out"=w1146:errorcluster)  [unwired: 7 in, 1 out]
                n350 = call "PADMINI_AUTO_CYCLE STATE 70.vi"("Enum"=w1151, "error in (no error)"=w1146, "Input"=w1153) -> ("error out"=w1147:errorcluster)  [unwired: 7 in, 1 out]
              }
              frame Error {
              }
            }
          }
          frame "Read2" {
            w1164 = u16 82 ("Data Block #")
            w1183 = PLC_Comm_State."Write"  # Enum
            # "Op80 Read2"
            n351 = call-poly <vilib>:"read DB.vi"("Item offset [byte]"=u32 8, "error in (no error)"=w1155, "items #"=u16 1 ("Items # [byte]"), "Data Block #"=w1164, "S7 Connection in"=w1156) -> ("error out"=w1170:errorcluster, "REAL result array"=w1181:sgl[], "S7 Connection out"=w1171:T5)  [unwired: 4 in]
            n352 = call-poly <vilib>:"read DB.vi"("Item offset [byte]"=u32 12, "String length reserved in DB (default=254)"=u16 50, "error in (no error)"=w1170, "items #"=u16 1 ("Items # [byte]"), "Data Block #"=w1164, "S7 Connection in"=w1171) -> ("error out"=w1173:errorcluster, "STRING result Array"=w1175:string[], "S7 Connection out"=w1176:T5)  [unwired: 2 in, 1 out]
            n353 = call-poly <vilib>:"read DB.vi"("Item offset [byte]"=u32 64, "String length reserved in DB (default=254)"=u16 10, "error in (no error)"=w1173, "items #"=u16 2 ("Items # [byte]"), "Data Block #"=w1164, "S7 Connection in"=w1176) -> ("error out"=w1174:errorcluster, "STRING result Array"=w1172:string[], "S7 Connection out"=w1179:T5)  [unwired: 2 in, 1 out]
            n354 = Build Array (concatenate)(w1175, w1172) -> (w1180:string[])
            n355 = call-poly <vilib>:"read DB.vi"("error in (no error)"=w1174, "items #"=u16 2 ("Items # [byte]"), "Data Block #"=u16 82, "S7 Connection in"=w1179) -> ("error out"=w1177:errorcluster, "DINT result array"=w1178:i32[], "S7 Connection out"=w1157:T5)  [unwired: 5 in]
            n356 = case shown="No Error" w1177 {
              selector: w1177 -> [w1186 w1192]
              tunnel: w1178 -> [w1191 _]
              tunnel: w1180 -> [w1189 _]
              tunnel: w1181 -> [w1188 _]
              tunnel: [w1184 w1192] -> w1158
              frame No Error {
                w1187 = enum16{"Read", "Write"}."Write" ("Enum")
                n357 = call "PADMINI_AUTO_CYCLE VALUE 80.vi"("Enum"=w1187, "error in (no error)"=w1186, "Input"=w1188) -> ("error out"=w1190:errorcluster)  [unwired: 7 in, 1 out]
                n358 = call "PADMINI_AUTO_BARCODE_STRING 80.vi"("Enum"=w1187, "error in (no error)"=w1190, "Input"=w1189) -> ("error out"=w1185:errorcluster)  [unwired: 7 in, 1 out]
                n359 = call "PADMINI_AUTO_CYCLE STATE 80.vi"("Enum"=w1187, "error in (no error)"=w1185, "Input"=w1191) -> ("error out"=w1184:errorcluster)  [unwired: 7 in, 1 out]
              }
              frame Error {
              }
            }
          }
          frame "Error" {
            w1194 = PLC_Comm_State."Write"  # Enum
            n360 = global write "Global 1.vi" "PLC6 error"(w1193) -> ()
            n361 = call <vilib>:"Clear Errors.vi"("error in (no error)"=w1193) -> ("error out"=w1196:errorcluster)  [unwired: 5 in, 1 out]
          }
          frame "Disconnect" {
            w1198 = PLC_Comm_State."Disconnect"  # Enum
            w1201 = T5 {"TCP Connection Ref"=refnum, "IP address"="", "timeout ms"=5000, "Connected?"=FALSE, "PLC Type"=enum."S7 1200", "Rack S7 400"=0, "Slot S7 400"=0, "PDU Size"=0, "connection semaphore"=refnum}  # S7 Connection out
            n362 = call <vilib>:"Clear Errors.vi"("error in (no error)"=w1202) -> ("error out"=w1205:errorcluster)  [unwired: 5 in, 1 out]
            n363 = call <vilib>:"disconnect.vi"("error in (no error)"=w1205, "S7 Connection in"=w1203) -> ("error out"=w1204:errorcluster)  [unwired: 8 in, 1 out]
          }
          frame "Write3" {
            # "No Use"
          }
          frame "Read3" {
            # "No Use"
          }
        }
        n364 = Wait (ms)(milliseconds to wait=w961) -> ()  [unwired: 1 out]
        n365 = call "PADMINI_STOP_ALL.vi"("Enum"=enum16{"Read", "Write"}."Read") -> ("Boolean 2"=w952:bool)  [unwired: 9 in, 1 out]
        n366 = local read "stop"() -> (w947:bool)
        n367 = case shown="Error" w965 {
          selector: w965 -> [w968 w969]
          tunnel: [w968 w975] -> w948
          tunnel: [w967 w971] -> w955
          tunnel: w960 -> [w967 _]
          tunnel: [w966 w981] -> w959
          tunnel: w958 -> [w966 w981]
          tunnel: w954 -> [_ w979]
          frame No Error {
          }
          frame Error {
            w972 = PLC_Comm_State."Connect"  # Enum
            w970 = PLC_Comm_State."Error"  # Enum
            n368 = Unbundle By Name(w969) -> ("source"=w980:string)
            n369 = call <userlib>:"Get Strings from Enum__ogtk.vi"("Enum"=w979) -> ("String Value"=w978:string)  [unwired: 7 in, 3 out]
            n370 = Concatenate Strings(w978, "    " ("string"), w980) -> (w976:string)
            n371 = Bundle By Name(cluster=w969, "source"=w976) -> (w975:errorcluster)
            n372 = call <vilib>:"Clear Errors.vi"("error in (no error)"=w969, "specific error code to clear (0: all)"=6002) -> ("specific error cleared?"=w974:bool)  [unwired: 4 in, 1 out]
            n373 = Select(t=w972, s=w974, f=w970) -> (s? t:f=w971:T1)
          }
        }
        n374 = Or(x=w947, y=w952) -> (x .or. y?=w950:bool)
        n375 = Select(t=w953, s=w950, f=w955) -> (s? t:f=w956:T1)
        n376 = Unbundle By Name(w948) -> ("status"=w949:bool)
        n377 = Not(x=w949) -> (.not. x?=w946:bool)
        n378 = global write "Global 1.vi" "PLC 6"(w946) -> ()
      }
    }
  }
  n379 = disable-structure shown="Enabled" {
    disable-tunnel: w29 -> [w1222 w1422]
    disable-tunnel: [w1221 w1420] -> w2
    disable-tunnel: w9 -> [w1215 w1421]
    frame Disabled {
      w1212 = TRUE  # Use Rack/Slot for S71200/1500
      w1213 = u8 1  # Slot S7 300/400
      w1214 = u8 0  # Rack S7 300/400
      n380 = call <vilib>:"connect.vi"("Use Rack/Slot for S71200/1500"=w1212, "Slot S7 300/400"=w1213, "PLC Type"=PLC_Type."S7 1200" ("PLC Type 2"), "error in (no error)"=w1215, "Rack S7 300/400"=w1214, "timeout [ms]"=1000 ("timeout [ms] 2"), "IP address"=w1222) -> ("error out"=w1217:errorcluster, "S7 Connection out"=w1216:T5)  [unwired: 3 in]
      n381 = for {
        tunnel: u16[] [69, 71] ("Data Block #") -> [w1230] mode=indexing
        shift-right: [w1228] -> w1219
        shift-left: w1216 -> [w1225]
        tunnel: w1217 -> [w1226]
        tunnel: [w1227] -> w1218
        w1229 = i32[] [0, 0]  # DINT input array
        # "Reset Search and save \nbit on software start"
        n382 = call-poly <vilib>:"write DB.vi"("DINT input array"=w1229, "error in (no error)"=w1226, "Data Block #"=w1230, "S7 Connection in"=w1225) -> ("error out"=w1227:errorcluster, "S7 Connection out"=w1228:T5)  [unwired: 4 in, 2 out]
      }
      n383 = while {
        shift-right: [w1233] -> w1210
        shift-left: w1219 -> [w1243]
        shift-right: [w1241] -> w1221
        shift-left: w1218 -> [w1242]
        tunnel: w1222 -> [w1232]
        stop <- w1235 stop-if-true
        # "OP 90 - 100"
        n384 = flat-sequence {
          tunnel: [w1245] -> w1239
          tunnel: [w1315] -> w1234
          tunnel: w1242 -> [w1340]
          tunnel: w1243 -> [w1339]
          tunnel: w1232 -> [w1327]
          tunnel: [w1327] -> w1231
          tunnel: [w1393] -> w1241
          tunnel: [w1392] -> w1233
          tunnel: w1239 -> [w1395]
          tunnel: w1234 -> [w1394]
          tunnel: w1231 -> [w1391]
          frame #0 {
            w1284 = u16 72 ("Data Block #")
            w1308 = u16 70 ("Data Block #")
            w1244 = u16 71 ("Data Block #")
            w1252 = u16 69 ("Data Block #")
            # "AUTO WRITE"
            n385 = global read "DATA LOG.vi" "OP 90 Outputs"() -> (w1338:bool)
            n386 = case shown="True" w1338 {
              tunnel: w1339 -> [w1376 w1389]
              tunnel: [w1377 w1378] -> w1313
              tunnel: [w1376 w1379] -> w1314
              tunnel: w1340 -> [w1377 w1386]
              frame False {
              }
              frame True {
                w1390 = u16 70  # Data Block #
                n387 = call "PADMINI_AUTO_BARCODE_STATUS 90.vi"("Enum"=enum16{"Read", "Write"}."Read", "error in (no error)"=w1386) -> ("error out"=w1385:errorcluster, "O/P"=w1387:i32[])  [unwired: 8 in]
                n388 = global write "DATA LOG.vi" "OP 90 Outputs"(FALSE) -> ()
                n389 = call-poly <vilib>:"write DB.vi"("DINT input array"=w1387, "error in (no error)"=w1385, "Data Block #"=w1390, "S7 Connection in"=w1389) -> ("error out"=w1381:errorcluster, "S7 Connection out"=w1380:T5)  [unwired: 4 in, 2 out]
                n390 = call-poly <vilib>:"write DB.vi"("DINT input array"=i32[] [0] ("Data Byte"), "error in (no error)"=w1381, "Data Block #"=u16 69, "S7 Connection in"=w1380) -> ("error out"=w1378:errorcluster, "S7 Connection out"=w1379:T5)  [unwired: 4 in, 2 out]
              }
            }
            n391 = global read "DATA LOG.vi" "OP 90 reset"() -> (w1312:bool)
            n392 = case shown="True" w1312 {
              tunnel: w1313 -> [w1351 w1360]
              tunnel: [w1351 w1359] -> w1301
              tunnel: w1314 -> [w1352 w1358]
              tunnel: [w1352 w1357] -> w1302
              frame False {
              }
              frame True {
                n393 = global write "DATA LOG.vi" "OP 90 reset"(FALSE) -> ()
                n394 = call-poly <vilib>:"write DB.vi"("Item offset [byte]"=u16 4 ("Data Block #"), "DINT input array"=i32[] [0], "error in (no error)"=w1360, "Data Block #"=u16 69, "S7 Connection in"=w1358) -> ("error out"=w1359:errorcluster, "S7 Connection out"=w1357:T5)  [unwired: 3 in, 2 out]
              }
            }
            n395 = global read "DATA LOG.vi" "Auto Cycle On"() -> (w1267:bool)
            n396 = Boolean To (0,1)(Boolean=w1267) -> (0, 1=w1266:i16)
            n397 = Build Array(w1266) -> (w1265:i16[])
            n398 = global read "Global 1.vi" "Filtered BARCODE selected"() -> (w1311:string[])
            n399 = call-poly <vilib>:"write DB.vi"("Item offset [byte]"=u32 20, "DINT input array"=w1265, "error in (no error)"=w1301, "Data Block #"=w1308, "S7 Connection in"=w1302) -> ("error out"=w1306:errorcluster, "S7 Connection out"=w1305:T5)  [unwired: 3 in, 2 out]
            n400 = call-poly <vilib>:"write DB.vi"("Item offset [byte]"=u32 24, "Input STRINGS"=w1311, "error in (no error)"=w1306, "String length reserved in DB (default=254)"=u16 15, "Data Block #"=w1308, "S7 Connection in"=w1305) -> ("error out"=w1303:errorcluster, "S7 Connection out"=w1304:T5)  [unwired: 2 in, 2 out]
            n401 = call-poly <vilib>:"read DB.vi"("Item offset [byte]"=u32 8, "error in (no error)"=w1303, "items #"=u16 2 ("Items # [byte]"), "Data Block #"=w1252, "S7 Connection in"=w1304) -> ("error out"=w1330:errorcluster, "REAL result array"=w1328:sgl[], "S7 Connection out"=w1336:T5)  [unwired: 4 in]
            n402 = call "PADMINI_AUTO_CYCLE VALUE 90.vi"("Enum"=enum16{"Read", "Write"}."Write", "error in (no error)"=w1330, "Input"=w1328) -> ("error out"=w1329:errorcluster)  [unwired: 7 in, 1 out]
            n403 = call-poly <vilib>:"read DB.vi"("Item offset [byte]"=u32 16, "String length reserved in DB (default=254)"=u16 50, "error in (no error)"=w1329, "items #"=u16 1 ("Items # [byte]"), "Data Block #"=w1252, "S7 Connection in"=w1336) -> ("error out"=w1300:errorcluster, "STRING result Array"=w1293:string[], "S7 Connection out"=w1299:T5)  [unwired: 2 in, 1 out]
            n404 = call-poly <vilib>:"read DB.vi"("Item offset [byte]"=u32 68, "String length reserved in DB (default=254)"=u16 10, "error in (no error)"=w1300, "items #"=u16 3 ("Items # [byte]"), "Data Block #"=w1252, "S7 Connection in"=w1299) -> ("error out"=w1298:errorcluster, "STRING result Array"=w1292:string[], "S7 Connection out"=w1255:T5)  [unwired: 2 in, 1 out]
            n405 = Build Array (concatenate)(w1293, w1292) -> (w1291:string[])
            n406 = call "PADMINI_AUTO_BARCODE_STRING 90.vi"("Enum"=enum16{"Read", "Write"}."Write", "error in (no error)"=w1298, "Input"=w1291) -> ("error out"=w1254:errorcluster)  [unwired: 7 in, 1 out]
            n407 = call-poly <vilib>:"read DB.vi"("error in (no error)"=w1254, "items #"=u16 2 ("Items # [byte]"), "Data Block #"=w1252, "S7 Connection in"=w1255) -> ("error out"=w1258:errorcluster, "DINT result array"=w1260:i32[], "S7 Connection out"=w1256:T5)  [unwired: 5 in]
            n408 = call "PADMINI_AUTO_CYCLE STATE 90.vi"("Enum"=enum16{"Read", "Write"}."Write", "error in (no error)"=w1258, "Input"=w1260) -> ("error out"=w1253:errorcluster)  [unwired: 7 in, 1 out]
            n409 = global read "DATA LOG.vi" "OP 100 Outputs"() -> (w1316:bool)
            n410 = case shown="True" w1316 {
              tunnel: w1256 -> [w1361 w1374]
              tunnel: [w1362 w1365] -> w1289
              tunnel: [w1361 w1366] -> w1290
              tunnel: w1253 -> [w1362 w1371]
              frame False {
              }
              frame True {
                w1375 = u16 72  # Data Block #
                n411 = call "PADMINI_AUTO_BARCODE_STATUS 100.vi"("Enum"=enum16{"Read", "Write"}."Read", "error in (no error)"=w1371) -> ("error out"=w1370:errorcluster, "O/P"=w1372:i32[])  [unwired: 8 in]
                n412 = global write "DATA LOG.vi" "OP 100 Outputs"(FALSE) -> ()
                n413 = call-poly <vilib>:"write DB.vi"("DINT input array"=w1372, "error in (no error)"=w1370, "Data Block #"=w1375, "S7 Connection in"=w1374) -> ("error out"=w1364:errorcluster, "S7 Connection out"=w1363:T5)  [unwired: 4 in, 2 out]
                n414 = call-poly <vilib>:"write DB.vi"("DINT input array"=i32[] [0] ("Data Byte"), "error in (no error)"=w1364, "Data Block #"=u16 71, "S7 Connection in"=w1363) -> ("error out"=w1365:errorcluster, "S7 Connection out"=w1366:T5)  [unwired: 4 in, 2 out]
              }
            }
            n415 = global read "DATA LOG.vi" "OP 100 reset"() -> (w1288:bool)
            n416 = case shown="True" w1288 {
              tunnel: w1289 -> [w1341 w1350]
              tunnel: [w1341 w1349] -> w1280
              tunnel: w1290 -> [w1342 w1348]
              tunnel: [w1342 w1347] -> w1279
              frame False {
              }
              frame True {
                n417 = global write "DATA LOG.vi" "OP 100 reset"(FALSE) -> ()
                n418 = call-poly <vilib>:"write DB.vi"("Item offset [byte]"=u16 4 ("Data Block #"), "DINT input array"=i32[] [0], "error in (no error)"=w1350, "Data Block #"=u16 71, "S7 Connection in"=w1348) -> ("error out"=w1349:errorcluster, "S7 Connection out"=w1347:T5)  [unwired: 3 in, 2 out]
              }
            }
            n419 = global read "DATA LOG.vi" "Auto Cycle On"() -> (w1264:bool)
            n420 = Boolean To (0,1)(Boolean=w1264) -> (0, 1=w1263:i16)
            n421 = Build Array(w1263) -> (w1262:i16[])
            n422 = global read "Global 1.vi" "Filtered BARCODE selected"() -> (w1281:string[])
            n423 = call-poly <vilib>:"write DB.vi"("Item offset [byte]"=u32 20, "DINT input array"=w1262, "error in (no error)"=w1280, "Data Block #"=w1284, "S7 Connection in"=w1279) -> ("error out"=w1286:errorcluster, "S7 Connection out"=w1287:T5)  [unwired: 3 in, 2 out]
            n424 = call-poly <vilib>:"write DB.vi"("Item offset [byte]"=u32 24, "Input STRINGS"=w1281, "error in (no error)"=w1286, "String length reserved in DB (default=254)"=u16 15, "Data Block #"=w1284, "S7 Connection in"=w1287) -> ("error out"=w1277:errorcluster, "S7 Connection out"=w1278:T5)  [unwired: 2 in, 2 out]
            n425 = call-poly <vilib>:"read DB.vi"("Item offset [byte]"=u32 8, "error in (no error)"=w1277, "items #"=u16 11 ("Items # [byte]"), "Data Block #"=w1244, "S7 Connection in"=w1278) -> ("error out"=w1324:errorcluster, "REAL result array"=w1326:sgl[], "S7 Connection out"=w1318:T5)  [unwired: 4 in]
            n426 = call "PADMINI_AUTO_CYCLE VALUE 100.vi"("Enum"=enum16{"Read", "Write"}."Write", "error in (no error)"=w1324, "Input"=w1326) -> ("error out"=w1325:errorcluster)  [unwired: 7 in, 1 out]
            n427 = call-poly <vilib>:"read DB.vi"("Item offset [byte]"=u32 52, "String length reserved in DB (default=254)"=u16 50, "error in (no error)"=w1325, "items #"=u16 1 ("Items # [byte]"), "Data Block #"=w1244, "S7 Connection in"=w1318) -> ("error out"=w1274:errorcluster, "STRING result Array"=w1272:string[], "S7 Connection out"=w1273:T5)  [unwired: 2 in, 1 out]
            n428 = call-poly <vilib>:"read DB.vi"("Item offset [byte]"=u32 104, "String length reserved in DB (default=254)"=u16 10, "error in (no error)"=w1274, "items #"=u16 2 ("Items # [byte]"), "Data Block #"=w1244, "S7 Connection in"=w1273) -> ("error out"=w1275:errorcluster, "STRING result Array"=w1270:string[], "S7 Connection out"=w1246:T5)  [unwired: 2 in, 1 out]
            n429 = Build Array (concatenate)(w1272, w1270) -> (w1271:string[])
            n430 = call "PADMINI_AUTO_BARCODE_STRING 100.vi"("Enum"=enum16{"Read", "Write"}."Write", "error in (no error)"=w1275, "Input"=w1271) -> ("error out"=w1247:errorcluster)  [unwired: 7 in, 1 out]
            n431 = call-poly <vilib>:"read DB.vi"("error in (no error)"=w1247, "items #"=u16 2 ("Items # [byte]"), "Data Block #"=w1244, "S7 Connection in"=w1246) -> ("error out"=w1250:errorcluster, "DINT result array"=w1251:i32[], "S7 Connection out"=w1245:T5)  [unwired: 5 in]
            n432 = call "PADMINI_AUTO_CYCLE STATE 100.vi"("Enum"=enum16{"Read", "Write"}."Write", "error in (no error)"=w1250, "Input"=w1251) -> ("error out"=w1315:errorcluster)  [unwired: 7 in, 1 out]
          }
          frame #1 {
            # "RECONNECT"
            n433 = case shown="Error" w1394 {
              selector: w1394 -> [w1399 w1400]
              tunnel: [w1398 w1404] -> w1392
              tunnel: [w1399 w1405] -> w1393
              tunnel: w1395 -> [w1398 w1403]
              tunnel: w1391 -> [_ w1402]
              frame No Error {
              }
              frame Error {
                n434 = Unbundle By Name(w1400) -> ("code"=w1401:i32)
                n435 = call <vilib>:"Clear Errors.vi"("error in (no error)"=w1400) -> ("error out"=w1406:errorcluster)  [unwired: 5 in, 1 out]
                n436 = case shown="1, 66" w1401 {
                  tunnel: w1406 -> [w1408 w1419]
                  tunnel: [w1408 w1417] -> w1405
                  tunnel: [w1409 w1416] -> w1404
                  tunnel: w1403 -> [w1409 w1413]
                  tunnel: w1402 -> [_ w1412]
                  tunnel: w1400 -> [w1407 _]
                  frame 0, Default {
                    n437 = global write "Global 1.vi" "PLC7 error"(w1407) -> ()
                  }
                  frame 1, 66 {
                    n438 = call <vilib>:"disconnect.vi"("error in (no error)"=w1419, "S7 Connection in"=w1413) -> ("error out"=w1418:errorcluster)  [unwired: 8 in, 1 out]
                    n439 = call <vilib>:"Clear Errors.vi"("error in (no error)"=w1418) -> ("error out"=w1415:errorcluster)  [unwired: 5 in, 1 out]
                    n440 = call <vilib>:"connect.vi"("Use Rack/Slot for S71200/1500"=TRUE, "Slot S7 300/400"=u8 1, "PLC Type"=PLC_Type."S7 1200" ("PLC Type 2"), "error in (no error)"=w1415, "IP address"=w1412) -> ("error out"=w1417:errorcluster, "S7 Connection out"=w1416:T5)  [unwired: 5 in]
                  }
                }
              }
            }
            n441 = Unbundle By Name(w1394) -> ("status"=w1397:bool)
            n442 = Not(x=w1397) -> (.not. x?=w1396:bool)
            "PLC 7" <- w1396
            n443 = global write "Global 1.vi" "PLC 7"(w1396) -> ()
          }
        }
        n444 = call "PADMINI_STOP_ALL.vi"("Enum"=enum16{"Read", "Write"}."Read") -> ("Boolean 2"=w1237:bool)  [unwired: 9 in, 1 out]
        n445 = local read "stop"() -> (w1236:bool)
        n446 = Or(x=w1236, y=w1237) -> (x .or. y?=w1235:bool)
        n447 = Wait (ms)(milliseconds to wait=u32 1200) -> ()  [unwired: 1 out]
      }
      n448 = call <vilib>:"Clear Errors.vi"() -> ("error out"=w1211:errorcluster)  [unwired: 6 in, 1 out]
      n449 = call <vilib>:"disconnect.vi"("error in (no error)"=w1211, "S7 Connection in"=w1210) -> ()  [unwired: 8 in, 2 out]
    }
    frame Enabled {
      w1423 = PLC_Comm_State."Int"  # Enum
      n450 = while {
        shift-right: [w1435] -> _
        shift-left: w1423 -> [w1443]
        shift-right: [w1427] -> w1420
        shift-left: w1421 -> [w1442]
        shift-right: [w1438] -> _
        shift-left: _ -> [w1441]
        tunnel: w1422 -> [w1424]
        stop <- w1436 stop-if-true
        w1432 = PLC_Comm_State."Disconnect"  # Enum
        w1440 = u32 800  # milliseconds to wait
        # "Int-->Write-->Read---if--Error-->reconnect\n               ^------v                                       v\n                ^------------------------------v"
        # "OP 90-100"
        n451 = case shown="\"Error\"" w1443 {
          selector: w1443 -> [w1463 w1481 w1518 w1564 w1618 w1654 w1667 w1671 _ _]
          tunnel: [w1468 w1483 w1500 w1545 w1594 w1630 w1668 w1676 w1679 w1681] -> w1444
          tunnel: [w1469 w1482 w1499 w1544 w1595 w1631 w1669 w1673 w1678 w1680] -> w1437
          tunnel: w1442 -> [w1466 w1477 w1497 w1547 w1598 w1629 w1665 w1674 w1679 w1681]
          tunnel: w1441 -> [w1464 _ w1498 w1546 w1599 w1628 w1669 w1675 w1678 w1680]
          tunnel: [w1462 w1480 w1517 w1565 w1617 w1655 w1666 w1670 _ _] -> w1439
          tunnel: [_ _ _ _ _ _ _ TRUE _ _] -> w1436
          tunnel: [w1463 w1481 w1518 w1564 w1618 w1654 w1667 w1671 _ _] -> w1433
          tunnel: w1424 -> [w1461 w1479 _ _ _ _ _ _ _ _]
          frame "Connect" {
            w1462 = PLC_Comm_State."Write"  # Enum
            w1474 = TRUE  # Use Rack/Slot for S71200/1500
            w1473 = u8 1  # Slot S7 300/400
            w1471 = u8 0  # Rack S7 300/400
            # "Reconect"
            n452 = call <vilib>:"disconnect.vi"("error in (no error)"=w1466, "S7 Connection in"=w1464) -> ("error out"=w1467:errorcluster)  [unwired: 8 in, 1 out]
            n453 = call <vilib>:"Clear Errors.vi"("error in (no error)"=w1467) -> ("error out"=w1465:errorcluster)  [unwired: 5 in, 1 out]
            n454 = call <vilib>:"connect.vi"("Use Rack/Slot for S71200/1500"=w1474, "Slot S7 300/400"=w1473, "PLC Type"=PLC_Type."S7 1200" ("PLC Type 2"), "error in (no error)"=w1465, "Rack S7 300/400"=w1471, "timeout [ms]"=1000 ("timeout [ms] 2"), "IP address"=w1461) -> ("error out"=w1468:errorcluster, "S7 Connection out"=w1469:T5)  [unwired: 3 in]
          }
          frame "Int" {
            w1480 = PLC_Comm_State."Write"  # Enum
            w1484 = TRUE  # Use Rack/Slot for S71200/1500
            w1485 = u8 1  # Slot S7 300/400
            w1486 = u8 0  # Rack S7 300/400
            # "Initialize and set first bits"
            n455 = call "Stall Data Flow.vim"("value in"=w1477, "milliseconds to wait"=u32 774) -> ("value out"=w1476:errorcluster)  [unwired: 1 out]
            n456 = call <vilib>:"connect.vi"("Use Rack/Slot for S71200/1500"=w1484, "Slot S7 300/400"=w1485, "PLC Type"=PLC_Type."S7 1200" ("PLC Type 2"), "error in (no error)"=w1476, "Rack S7 300/400"=w1486, "timeout [ms]"=1000 ("timeout [ms] 2"), "IP address"=w1479) -> ("error out"=w1488:errorcluster, "S7 Connection out"=w1487:T5)  [unwired: 3 in]
            n457 = for {
              tunnel: u16[] [69, 71] ("Data Block #") -> [w1496] mode=indexing
              shift-right: [w1494] -> w1482
              shift-left: w1487 -> [w1492]
              tunnel: w1488 -> [w1493]
              tunnel: [w1491] -> w1483
              w1495 = i32[] [0, 0]  # DINT input array
              # "Reset Search and save \nbit on software start"
              n458 = call-poly <vilib>:"write DB.vi"("DINT input array"=w1495, "error in (no error)"=w1493, "Data Block #"=w1496, "S7 Connection in"=w1492) -> ("error out"=w1491:errorcluster, "S7 Connection out"=w1494:T5)  [unwired: 4 in, 2 out]
            }
          }
          frame "Write" {
            w1502 = u16 70 ("Data Block #")
            w1517 = PLC_Comm_State."Write2"  # Enum
            # "OP 90 Write"
            n459 = global read "DATA LOG.vi" "OP 90 Outputs"() -> (w1510:bool)
            n460 = case shown="True" w1510 {
              tunnel: [w1529 w1534] -> w1511
              tunnel: [w1530 w1535] -> w1512
              tunnel: w1498 -> [w1530 w1532]
              tunnel: w1497 -> [w1529 w1531]
              frame False {
              }
              frame True {
                w1543 = u16 70  # Data Block #
                n461 = call "PADMINI_AUTO_BARCODE_STATUS 90.vi"("Enum"=enum16{"Read", "Write"}."Read", "error in (no error)"=w1531) -> ("error out"=w1540:errorcluster, "O/P"=w1541:i32[])  [unwired: 8 in]
                n462 = call-poly <vilib>:"write DB.vi"("DINT input array"=w1541, "error in (no error)"=w1540, "Data Block #"=w1543, "S7 Connection in"=w1532) -> ("error out"=w1537:errorcluster, "S7 Connection out"=w1536:T5)  [unwired: 4 in, 2 out]
                n463 = call-poly <vilib>:"write DB.vi"("DINT input array"=i32[] [0] ("Data Byte"), "error in (no error)"=w1537, "Data Block #"=u16 69, "S7 Connection in"=w1536) -> ("error out"=w1534:errorcluster, "S7 Connection out"=w1535:T5)  [unwired: 4 in, 2 out]
                n464 = Unbundle By Name(w1534) -> ("status"=w1533:bool)
                n465 = global write "DATA LOG.vi" "OP 90 Outputs"(w1533) -> ()
              }
            }
            n466 = global read "DATA LOG.vi" "Auto Cycle On"() -> (w1506:bool)
            n467 = global read "DATA LOG.vi" "OP 90 reset"() -> (w1516:bool)
            n468 = Boolean To (0,1)(Boolean=w1506) -> (0, 1=w1505:i16)
            n469 = case shown="True" w1516 {
              tunnel: w1511 -> [w1519 w1525]
              tunnel: w1512 -> [w1520 w1524]
              tunnel: [w1520 w1523] -> w1513
              tunnel: [w1519 w1522] -> w1514
              frame False {
              }
              frame True {
                n470 = call-poly <vilib>:"write DB.vi"("Item offset [byte]"=u16 4 ("Data Block #"), "DINT input array"=i32[] [0], "error in (no error)"=w1525, "Data Block #"=u16 69, "S7 Connection in"=w1524) -> ("error out"=w1522:errorcluster, "S7 Connection out"=w1523:T5)  [unwired: 3 in, 2 out]
                n471 = Unbundle By Name(w1522) -> ("status"=w1521:bool)
                n472 = global write "DATA LOG.vi" "OP 90 reset"(w1521) -> ()
              }
            }
            n473 = Build Array(w1505) -> (w1515:i16[])
            n474 = global read "Global 1.vi" "Filtered BARCODE selected"() -> (w1509:string[])
            n475 = call-poly <vilib>:"write DB.vi"("Item offset [byte]"=u32 20, "DINT input array"=w1515, "error in (no error)"=w1514, "Data Block #"=w1502, "S7 Connection in"=w1513) -> ("error out"=w1508:errorcluster, "S7 Connection out"=w1507:T5)  [unwired: 3 in, 2 out]
            n476 = call-poly <vilib>:"write DB.vi"("Item offset [byte]"=u32 24, "Input STRINGS"=w1509, "error in (no error)"=w1508, "String length reserved in DB (default=254)"=u16 15, "Data Block #"=w1502, "S7 Connection in"=w1507) -> ("error out"=w1500:errorcluster, "S7 Connection out"=w1499:T5)  [unwired: 2 in, 2 out]
          }
          frame "Write2" {
            w1549 = u16 72 ("Data Block #")
            w1565 = PLC_Comm_State."Read"  # Enum
            # "op 100 wirte 2"
            n477 = global read "DATA LOG.vi" "OP 100 Outputs"() -> (w1563:bool)
            n478 = case shown="True" w1563 {
              tunnel: w1546 -> [w1576 w1589]
              tunnel: [w1577 w1579] -> w1561
              tunnel: [w1576 w1582] -> w1562
              tunnel: w1547 -> [w1577 w1586]
              frame False {
              }
              frame True {
                w1590 = u16 72  # Data Block #
                n479 = call "PADMINI_AUTO_BARCODE_STATUS 100.vi"("Enum"=enum16{"Read", "Write"}."Read", "error in (no error)"=w1586) -> ("error out"=w1585:errorcluster, "O/P"=w1587:i32[])  [unwired: 8 in]
                n480 = call-poly <vilib>:"write DB.vi"("DINT input array"=w1587, "error in (no error)"=w1585, "Data Block #"=w1590, "S7 Connection in"=w1589) -> ("error out"=w1581:errorcluster, "S7 Connection out"=w1580:T5)  [unwired: 4 in, 2 out]
                n481 = call-poly <vilib>:"write DB.vi"("DINT input array"=i32[] [0] ("Data Byte"), "error in (no error)"=w1581, "Data Block #"=u16 71, "S7 Connection in"=w1580) -> ("error out"=w1579:errorcluster, "S7 Connection out"=w1582:T5)  [unwired: 4 in, 2 out]
                n482 = Unbundle By Name(w1579) -> ("status"=w1578:bool)
                n483 = global write "DATA LOG.vi" "OP 100 Outputs"(w1578) -> ()
              }
            }
            n484 = global read "DATA LOG.vi" "OP 100 reset"() -> (w1560:bool)
            n485 = case shown="True" w1560 {
              tunnel: w1561 -> [w1566 w1575]
              tunnel: [w1566 w1569] -> w1556
              tunnel: w1562 -> [w1567 w1574]
              tunnel: [w1567 w1573] -> w1555
              frame False {
              }
              frame True {
                n486 = call-poly <vilib>:"write DB.vi"("Item offset [byte]"=u16 4 ("Data Block #"), "DINT input array"=i32[] [0], "error in (no error)"=w1575, "Data Block #"=u16 71, "S7 Connection in"=w1574) -> ("error out"=w1569:errorcluster, "S7 Connection out"=w1573:T5)  [unwired: 3 in, 2 out]
                n487 = Unbundle By Name(w1569) -> ("status"=w1568:bool)
                n488 = global write "DATA LOG.vi" "OP 100 reset"(w1568) -> ()
              }
            }
            n489 = global read "DATA LOG.vi" "Auto Cycle On"() -> (w1554:bool)
            n490 = global read "Global 1.vi" "Filtered BARCODE selected"() -> (w1557:string[])
            n491 = Boolean To (0,1)(Boolean=w1554) -> (0, 1=w1553:i16)
            n492 = Build Array(w1553) -> (w1552:i16[])
            n493 = call-poly <vilib>:"write DB.vi"("Item offset [byte]"=u32 20, "DINT input array"=w1552, "error in (no error)"=w1556, "Data Block #"=w1549, "S7 Connection in"=w1555) -> ("error out"=w1558:errorcluster, "S7 Connection out"=w1559:T5)  [unwired: 3 in, 2 out]
            n494 = call-poly <vilib>:"write DB.vi"("Item offset [byte]"=u32 24, "Input STRINGS"=w1557, "error in (no error)"=w1558, "String length reserved in DB (default=254)"=u16 15, "Data Block #"=w1549, "S7 Connection in"=w1559) -> ("error out"=w1545:errorcluster, "S7 Connection out"=w1544:T5)  [unwired: 2 in, 2 out]
          }
          frame "Read" {
            w1608 = u16 69 ("Data Block #")
            w1617 = PLC_Comm_State."Read2"  # Enum
            # "OP90 read"
            n495 = call-poly <vilib>:"read DB.vi"("Item offset [byte]"=u32 8, "error in (no error)"=w1598, "items #"=u16 2 ("Items # [byte]"), "Data Block #"=w1608, "S7 Connection in"=w1599) -> ("error out"=w1615:errorcluster, "REAL result array"=w1591:sgl[], "S7 Connection out"=w1616:T5)  [unwired: 4 in]
            n496 = call-poly <vilib>:"read DB.vi"("Item offset [byte]"=u32 16, "String length reserved in DB (default=254)"=u16 50, "error in (no error)"=w1615, "items #"=u16 1 ("Items # [byte]"), "Data Block #"=w1608, "S7 Connection in"=w1616) -> ("error out"=w1614:errorcluster, "STRING result Array"=w1612:string[], "S7 Connection out"=w1613:T5)  [unwired: 2 in, 1 out]
            n497 = call-poly <vilib>:"read DB.vi"("Item offset [byte]"=u32 68, "String length reserved in DB (default=254)"=u16 10, "error in (no error)"=w1614, "items #"=u16 3 ("Items # [byte]"), "Data Block #"=w1608, "S7 Connection in"=w1613) -> ("error out"=w1592:errorcluster, "STRING result Array"=w1611:string[], "S7 Connection out"=w1610:T5)  [unwired: 2 in, 1 out]
            n498 = Build Array (concatenate)(w1612, w1611) -> (w1597:string[])
            n499 = call-poly <vilib>:"read DB.vi"("error in (no error)"=w1592, "items #"=u16 2 ("Items # [byte]"), "Data Block #"=w1608, "S7 Connection in"=w1610) -> ("error out"=w1593:errorcluster, "DINT result array"=w1596:i32[], "S7 Connection out"=w1595:T5)  [unwired: 5 in]
            n500 = case shown="No Error" w1593 {
              selector: w1593 -> [w1621 w1627]
              tunnel: w1596 -> [w1626 _]
              tunnel: w1597 -> [w1625 _]
              tunnel: [w1620 w1627] -> w1594
              tunnel: w1591 -> [w1619 _]
              frame No Error {
                w1624 = enum16{"Read", "Write"}."Write" ("Enum")
                n501 = call "PADMINI_AUTO_CYCLE VALUE 90.vi"("Enum"=w1624, "error in (no error)"=w1621, "Input"=w1619) -> ("error out"=w1623:errorcluster)  [unwired: 7 in, 1 out]
                n502 = call "PADMINI_AUTO_BARCODE_STRING 90.vi"("Enum"=w1624, "error in (no error)"=w1623, "Input"=w1625) -> ("error out"=w1622:errorcluster)  [unwired: 7 in, 1 out]
                n503 = call "PADMINI_AUTO_CYCLE STATE 90.vi"("Enum"=w1624, "error in (no error)"=w1622, "Input"=w1626) -> ("error out"=w1620:errorcluster)  [unwired: 7 in, 1 out]
              }
              frame Error {
              }
            }
          }
          frame "Read2" {
            w1640 = u16 71 ("Data Block #")
            w1655 = PLC_Comm_State."Write"  # Enum
            # "Op100 Read2"
            n504 = call-poly <vilib>:"read DB.vi"("Item offset [byte]"=u32 8, "error in (no error)"=w1629, "items #"=u16 11 ("Items # [byte]"), "Data Block #"=w1640, "S7 Connection in"=w1628) -> ("error out"=w1651:errorcluster, "REAL result array"=w1653:sgl[], "S7 Connection out"=w1650:T5)  [unwired: 4 in]
            n505 = call-poly <vilib>:"read DB.vi"("Item offset [byte]"=u32 52, "String length reserved in DB (default=254)"=u16 50, "error in (no error)"=w1651, "items #"=u16 1 ("Items # [byte]"), "Data Block #"=w1640, "S7 Connection in"=w1650) -> ("error out"=w1648:errorcluster, "STRING result Array"=w1646:string[], "S7 Connection out"=w1647:T5)  [unwired: 2 in, 1 out]
            n506 = call-poly <vilib>:"read DB.vi"("Item offset [byte]"=u32 104, "String length reserved in DB (default=254)"=u16 10, "error in (no error)"=w1648, "items #"=u16 2 ("Items # [byte]"), "Data Block #"=w1640, "S7 Connection in"=w1647) -> ("error out"=w1649:errorcluster, "STRING result Array"=w1645:string[], "S7 Connection out"=w1642:T5)  [unwired: 2 in, 1 out]
            n507 = Build Array (concatenate)(w1646, w1645) -> (w1652:string[])
            n508 = call-poly <vilib>:"read DB.vi"("error in (no error)"=w1649, "items #"=u16 2 ("Items # [byte]"), "Data Block #"=w1640, "S7 Connection in"=w1642) -> ("error out"=w1643:errorcluster, "DINT result array"=w1644:i32[], "S7 Connection out"=w1631:T5)  [unwired: 5 in]
            n509 = case shown="No Error" w1643 {
              selector: w1643 -> [w1660 w1664]
              tunnel: w1644 -> [w1663 _]
              tunnel: w1652 -> [w1658 _]
              tunnel: w1653 -> [w1657 _]
              tunnel: [w1656 w1664] -> w1630
              frame No Error {
                w1659 = enum16{"Read", "Write"}."Write" ("Enum")
                n510 = call "PADMINI_AUTO_CYCLE VALUE 100.vi"("Enum"=w1659, "error in (no error)"=w1660, "Input"=w1657) -> ("error out"=w1661:errorcluster)  [unwired: 7 in, 1 out]
                n511 = call "PADMINI_AUTO_BARCODE_STRING 100.vi"("Enum"=w1659, "error in (no error)"=w1661, "Input"=w1658) -> ("error out"=w1662:errorcluster)  [unwired: 7 in, 1 out]
                n512 = call "PADMINI_AUTO_CYCLE STATE 100.vi"("Enum"=w1659, "error in (no error)"=w1662, "Input"=w1663) -> ("error out"=w1656:errorcluster)  [unwired: 7 in, 1 out]
              }
              frame Error {
              }
            }
          }
          frame "Error" {
            w1666 = PLC_Comm_State."Write"  # Enum
            n513 = global write "Global 1.vi" "PLC7 error"(w1665) -> ()
            n514 = call <vilib>:"Clear Errors.vi"("error in (no error)"=w1665) -> ("error out"=w1668:errorcluster)  [unwired: 5 in, 1 out]
          }
          frame "Disconnect" {
            w1670 = PLC_Comm_State."Disconnect"  # Enum
            w1673 = T5 {"TCP Connection Ref"=refnum, "IP address"="", "timeout ms"=5000, "Connected?"=FALSE, "PLC Type"=enum."S7 1200", "Rack S7 400"=0, "Slot S7 400"=0, "PDU Size"=0, "connection semaphore"=refnum}  # S7 Connection out
            n515 = call <vilib>:"Clear Errors.vi"("error in (no error)"=w1674) -> ("error out"=w1677:errorcluster)  [unwired: 5 in, 1 out]
            n516 = call <vilib>:"disconnect.vi"("error in (no error)"=w1677, "S7 Connection in"=w1675) -> ("error out"=w1676:errorcluster)  [unwired: 8 in, 1 out]
          }
          frame "Write3" {
            # "No Use"
          }
          frame "Read3" {
            # "No Use"
          }
        }
        n517 = Wait (ms)(milliseconds to wait=w1440) -> ()  [unwired: 1 out]
        n518 = call "PADMINI_STOP_ALL.vi"("Enum"=enum16{"Read", "Write"}."Read") -> ("Boolean 2"=w1431:bool)  [unwired: 9 in, 1 out]
        n519 = local read "stop"() -> (w1426:bool)
        n520 = case shown="Error" w1444 {
          selector: w1444 -> [w1447 w1448]
          tunnel: [w1447 w1454] -> w1427
          tunnel: [w1446 w1450] -> w1434
          tunnel: w1439 -> [w1446 _]
          tunnel: [w1445 w1460] -> w1438
          tunnel: w1437 -> [w1445 w1460]
          tunnel: w1433 -> [_ w1458]
          frame No Error {
          }
          frame Error {
            w1451 = PLC_Comm_State."Connect"  # Enum
            w1449 = PLC_Comm_State."Error"  # Enum
            n521 = Unbundle By Name(w1448) -> ("source"=w1459:string)
            n522 = call <userlib>:"Get Strings from Enum__ogtk.vi"("Enum"=w1458) -> ("String Value"=w1457:string)  [unwired: 7 in, 3 out]
            n523 = Concatenate Strings(w1457, "    " ("string"), w1459) -> (w1455:string)
            n524 = Bundle By Name(cluster=w1448, "source"=w1455) -> (w1454:errorcluster)
            n525 = call <vilib>:"Clear Errors.vi"("error in (no error)"=w1448, "specific error code to clear (0: all)"=6002) -> ("specific error cleared?"=w1453:bool)  [unwired: 4 in, 1 out]
            n526 = Select(t=w1451, s=w1453, f=w1449) -> (s? t:f=w1450:T1)
          }
        }
        n527 = Or(x=w1426, y=w1431) -> (x .or. y?=w1429:bool)
        n528 = Select(t=w1432, s=w1429, f=w1434) -> (s? t:f=w1435:T1)
        n529 = Unbundle By Name(w1427) -> ("status"=w1428:bool)
        n530 = Not(x=w1428) -> (.not. x?=w1425:bool)
        n531 = global write "Global 1.vi" "PLC 7"(w1425) -> ()
      }
    }
  }
  n532 = disable-structure shown="Enabled" {
    disable-tunnel: w71 -> [w1694 w1819]
    disable-tunnel: w9 -> [w1687 w1818]
    disable-tunnel: [w1682 w1817] -> w4
    frame Disabled {
      w1684 = TRUE  # Use Rack/Slot for S71200/1500
      w1685 = u8 1  # Slot S7 300/400
      w1686 = u8 0  # Rack S7 300/400
      w1693 = i32[] [0, 0]  # DINT input array
      # "Reset Search and save \nbit on software start"
      n533 = call <vilib>:"connect.vi"("Use Rack/Slot for S71200/1500"=w1684, "Slot S7 300/400"=w1685, "PLC Type"=PLC_Type."S7 1200" ("PLC Type 2"), "error in (no error)"=w1687, "Rack S7 300/400"=w1686, "timeout [ms]"=1000 ("timeout [ms] 2"), "IP address"=w1694) -> ("error out"=w1689:errorcluster, "S7 Connection out"=w1688:T5)  [unwired: 3 in]
      n534 = call-poly <vilib>:"write DB.vi"("DINT input array"=w1693, "error in (no error)"=w1689, "Data Block #"=u16 56, "S7 Connection in"=w1688) -> ("error out"=w1690:errorcluster, "S7 Connection out"=w1691:T5)  [unwired: 4 in, 2 out]
      n535 = while {
        shift-right: [w1701] -> w1698
        shift-left: w1691 -> [w1711]
        shift-right: [w1709] -> w1697
        shift-left: w1690 -> [w1710]
        tunnel: w1694 -> [w1700]
        stop <- w1703 stop-if-true
        # "OP 50"
        n536 = flat-sequence {
          tunnel: [w1714] -> w1707
          tunnel: [w1712] -> w1702
          tunnel: w1710 -> [w1762]
          tunnel: w1711 -> [w1761]
          tunnel: w1700 -> [w1749]
          tunnel: [w1749] -> w1699
          tunnel: [w1790] -> w1709
          tunnel: [w1789] -> w1701
          tunnel: w1707 -> [w1792]
          tunnel: w1702 -> [w1791]
          tunnel: w1699 -> [w1788]
          frame #0 {
            w1732 = u16 57 ("Data Block #")
            w1740 = u16 56 ("Data Block #")
            # "AUTO WRITE"
            n537 = global read "DATA LOG.vi" "OP 50 Outputs"() -> (w1760:bool)
            n538 = case shown="True" w1760 {
              tunnel: w1761 -> [w1773 w1786]
              tunnel: [w1774 w1775] -> w1748
              tunnel: [w1773 w1778] -> w1747
              tunnel: w1762 -> [w1774 w1783]
              frame False {
              }
              frame True {
                w1787 = u16 57  # Data Block #
                n539 = call "PADMINI_AUTO_BARCODE_STATUS 50.vi"("Enum"=enum16{"Read", "Write"}."Read", "error in (no error)"=w1783) -> ("error out"=w1782:errorcluster, "O/P"=w1784:i32[])  [unwired: 8 in]
                n540 = global write "DATA LOG.vi" "OP 50 Outputs"(FALSE) -> ()
                n541 = call-poly <vilib>:"write DB.vi"("DINT input array"=w1784, "error in (no error)"=w1782, "Data Block #"=w1787, "S7 Connection in"=w1786) -> ("error out"=w1776:errorcluster, "S7 Connection out"=w1777:T5)  [unwired: 4 in, 2 out]
                n542 = call-poly <vilib>:"write DB.vi"("DINT input array"=i32[] [0] ("Data Byte"), "error in (no error)"=w1776, "Data Block #"=u16 56, "S7 Connection in"=w1777) -> ("error out"=w1775:errorcluster, "S7 Connection out"=w1778:T5)  [unwired: 4 in, 2 out]
              }
            }
            n543 = global read "DATA LOG.vi" "OP 50 reset"() -> (w1746:bool)
            n544 = global read "DATA LOG.vi" "Auto Cycle On"() -> (w1723:bool)
            n545 = case shown="True" w1746 {
              tunnel: w1748 -> [w1763 w1772]
              tunnel: [w1763 w1771] -> w1725
              tunnel: w1747 -> [w1764 w1770]
              tunnel: [w1764 w1769] -> w1728
              frame False {
              }
              frame True {
                n546 = global write "DATA LOG.vi" "OP 50 reset"(FALSE) -> ()
                n547 = call-poly <vilib>:"write DB.vi"("Item offset [byte]"=u16 4 ("Data Block #"), "DINT input array"=i32[] [0], "error in (no error)"=w1772, "Data Block #"=u16 56, "S7 Connection in"=w1770) -> ("error out"=w1771:errorcluster, "S7 Connection out"=w1769:T5)  [unwired: 3 in, 2 out]
              }
            }
            n548 = Boolean To (0,1)(Boolean=w1723) -> (0, 1=w1722:i16)
            n549 = Build Array(w1722) -> (w1721:i16[])
            n550 = global read "Global 1.vi" "Filtered BARCODE selected"() -> (w1729:string[])
            n551 = call-poly <vilib>:"write DB.vi"("Item offset [byte]"=u32 20, "DINT input array"=w1721, "error in (no error)"=w1725, "Data Block #"=w1732, "S7 Connection in"=w1728) -> ("error out"=w1734:errorcluster, "S7 Connection out"=w1735:T5)  [unwired: 3 in, 2 out]
            n552 = call-poly <vilib>:"write DB.vi"("Item offset [byte]"=u32 24, "Input STRINGS"=w1729, "error in (no error)"=w1734, "String length reserved in DB (default=254)"=u16 15, "Data Block #"=w1732, "S7 Connection in"=w1735) -> ("error out"=w1726:errorcluster, "S7 Connection out"=w1727:T5)  [unwired: 2 in, 2 out]
            n553 = call-poly <vilib>:"read DB.vi"("Item offset [byte]"=u32 8, "error in (no error)"=w1726, "items #"=u16 3 ("Items # [byte]"), "Data Block #"=w1740, "S7 Connection in"=w1727) -> ("error out"=w1752:errorcluster, "REAL result array"=w1750:sgl[], "S7 Connection out"=w1758:T5)  [unwired: 4 in]
            n554 = call "PADMINI_AUTO_CYCLE VALUE 50.vi"("Enum"=enum16{"Read", "Write"}."Write", "error in (no error)"=w1752, "Input"=w1750) -> ("error out"=w1751:errorcluster)  [unwired: 7 in, 1 out]
            n555 = call-poly <vilib>:"read DB.vi"("Item offset [byte]"=u32 20, "String length reserved in DB (default=254)"=u16 50, "error in (no error)"=w1751, "items #"=u16 1 ("Items # [byte]"), "Data Block #"=w1740, "S7 Connection in"=w1758) -> ("error out"=w1742:errorcluster, "STRING result Array"=w1739:string[], "S7 Connection out"=w1741:T5)  [unwired: 2 in, 1 out]
            n556 = call-poly <vilib>:"read DB.vi"("Item offset [byte]"=u32 72, "String length reserved in DB (default=254)"=u16 10, "error in (no error)"=w1742, "items #"=u16 5 ("Items # [byte]"), "Data Block #"=w1740, "S7 Connection in"=w1741) -> ("error out"=w1743:errorcluster, "STRING result Array"=w1738:string[], "S7 Connection out"=w1715:T5)  [unwired: 2 in, 1 out]
            n557 = Build Array (concatenate)(w1739, w1738) -> (w1737:string[])
            n558 = call "PADMINI_AUTO_BARCODE_STRING 50.vi"("Enum"=enum16{"Read", "Write"}."Write", "error in (no error)"=w1743, "Input"=w1737) -> ("error out"=w1713:errorcluster)  [unwired: 7 in, 1 out]
            n559 = call-poly <vilib>:"read DB.vi"("error in (no error)"=w1713, "items #"=u16 2 ("Items # [byte]"), "Data Block #"=u16 56, "S7 Connection in"=w1715) -> ("error out"=w1717:errorcluster, "DINT result array"=w1719:i32[], "S7 Connection out"=w1714:T5)  [unwired: 5 in]
            n560 = call "PADMINI_AUTO_CYCLE STATE 50.vi"("Enum"=enum16{"Read", "Write"}."Write", "error in (no error)"=w1717, "Input"=w1719) -> ("error out"=w1712:errorcluster)  [unwired: 7 in, 1 out]
          }
          frame #1 {
            # "RECONNECT"
            n561 = case shown="Error" w1791 {
              selector: w1791 -> [w1796 w1797]
              tunnel: [w1795 w1801] -> w1789
              tunnel: [w1796 w1802] -> w1790
              tunnel: w1792 -> [w1795 w1800]
              tunnel: w1788 -> [_ w1799]
              frame No Error {
              }
              frame Error {
                n562 = Unbundle By Name(w1797) -> ("code"=w1798:i32)
                n563 = call <vilib>:"Clear Errors.vi"("error in (no error)"=w1797) -> ("error out"=w1803:errorcluster)  [unwired: 5 in, 1 out]
                n564 = case shown="1, 66" w1798 {
                  tunnel: w1803 -> [w1805 w1816]
                  tunnel: [w1805 w1814] -> w1802
                  tunnel: [w1806 w1813] -> w1801
                  tunnel: w1800 -> [w1806 w1810]
                  tunnel: w1799 -> [_ w1809]
                  tunnel: w1797 -> [w1804 _]
                  frame 0, Default {
                    n565 = global write "Global 1.vi" "PLC4 error"(w1804) -> ()
                  }
                  frame 1, 66 {
                    n566 = call <vilib>:"disconnect.vi"("error in (no error)"=w1816, "S7 Connection in"=w1810) -> ("error out"=w1815:errorcluster)  [unwired: 8 in, 1 out]
                    n567 = call <vilib>:"Clear Errors.vi"("error in (no error)"=w1815) -> ("error out"=w1812:errorcluster)  [unwired: 5 in, 1 out]
                    n568 = call <vilib>:"connect.vi"("Use Rack/Slot for S71200/1500"=TRUE, "Slot S7 300/400"=u8 1, "PLC Type"=PLC_Type."S7 1200" ("PLC Type 2"), "error in (no error)"=w1812, "IP address"=w1809) -> ("error out"=w1814:errorcluster, "S7 Connection out"=w1813:T5)  [unwired: 5 in]
                  }
                }
              }
            }
            n569 = Unbundle By Name(w1791) -> ("status"=w1794:bool)
            n570 = Not(x=w1794) -> (.not. x?=w1793:bool)
            "PLC 4" <- w1793
            n571 = global write "Global 1.vi" "PLC 4"(w1793) -> ()
          }
        }
        n572 = call "PADMINI_STOP_ALL.vi"("Enum"=enum16{"Read", "Write"}."Read") -> ("Boolean 2"=w1705:bool)  [unwired: 9 in, 1 out]
        n573 = local read "stop"() -> (w1704:bool)
        n574 = Or(x=w1704, y=w1705) -> (x .or. y?=w1703:bool)
        n575 = Wait (ms)(milliseconds to wait=u32 1200) -> ()  [unwired: 1 out]
      }
      n576 = call <vilib>:"Clear Errors.vi"("error in (no error)"=w1697) -> ("error out"=w1683:errorcluster)  [unwired: 5 in, 1 out]
      n577 = call <vilib>:"disconnect.vi"("error in (no error)"=w1683, "S7 Connection in"=w1698) -> ("error out"=w1682:errorcluster)  [unwired: 8 in, 1 out]
    }
    frame Enabled {
      w1820 = PLC_Comm_State."Int"  # Enum
      n578 = while {
        shift-right: [w1832] -> _
        shift-left: w1820 -> [w1840]
        shift-right: [w1824] -> w1817
        shift-left: w1818 -> [w1839]
        shift-right: [w1835] -> _
        shift-left: _ -> [w1838]
        tunnel: w1819 -> [w1821]
        stop <- w1833 stop-if-true
        w1829 = PLC_Comm_State."Disconnect"  # Enum
        w1837 = u32 800  # milliseconds to wait
        # "Int-->Write-->Read---if--Error-->reconnect\n               ^------v                                       v\n                ^------------------------------v"
        # "OP 50"
        n579 = case shown="\"Error\"" w1840 {
          selector: w1840 -> [w1860 w1877 w1915 w1968 w1980 w1983 _ _ _ _]
          tunnel: [w1865 w1879 w1895 w1943 w1979 w1988 w1990 w1993 w1995 w1997] -> w1841
          tunnel: [w1866 w1878 w1894 w1942 w1981 w1985 w1991 w1992 w1994 w1996] -> w1834
          tunnel: w1839 -> [w1863 w1873 w1896 w1944 w1979 w1986 w1990 w1993 w1995 w1997]
          tunnel: w1838 -> [w1861 _ w1897 w1941 w1981 w1987 w1991 w1992 w1994 w1996]
          tunnel: [w1859 w1876 w1914 w1967 w1978 w1982 _ _ _ _] -> w1836
          tunnel: [_ _ _ _ _ TRUE _ _ _ _] -> w1833
          tunnel: [w1860 w1877 w1915 w1968 w1980 w1983 _ _ _ _] -> w1830
          tunnel: w1821 -> [w1858 w1875 _ _ _ _ _ _ _ _]
          frame "Connect" {
            w1859 = PLC_Comm_State."Write"  # Enum
            w1871 = TRUE  # Use Rack/Slot for S71200/1500
            w1870 = u8 1  # Slot S7 300/400
            w1868 = u8 0  # Rack S7 300/400
            # "Reconect"
            n580 = call <vilib>:"disconnect.vi"("error in (no error)"=w1863, "S7 Connection in"=w1861) -> ("error out"=w1864:errorcluster)  [unwired: 8 in, 1 out]
            n581 = call <vilib>:"Clear Errors.vi"("error in (no error)"=w1864) -> ("error out"=w1862:errorcluster)  [unwired: 5 in, 1 out]
            n582 = call <vilib>:"connect.vi"("Use Rack/Slot for S71200/1500"=w1871, "Slot S7 300/400"=w1870, "PLC Type"=PLC_Type."S7 1200" ("PLC Type 2"), "error in (no error)"=w1862, "Rack S7 300/400"=w1868, "timeout [ms]"=1000 ("timeout [ms] 2"), "IP address"=w1858) -> ("error out"=w1865:errorcluster, "S7 Connection out"=w1866:T5)  [unwired: 3 in]
          }
          frame "Int" {
            w1876 = PLC_Comm_State."Write"  # Enum
            w1880 = TRUE  # Use Rack/Slot for S71200/1500
            w1881 = u8 1  # Slot S7 300/400
            w1882 = u8 0  # Rack S7 300/400
            w1883 = u16[] [56]  # Data Block #
            # "Initialize and set first bits"
            n583 = call "Stall Data Flow.vim"("value in"=w1873, "milliseconds to wait"=u32 387) -> ("value out"=w1872:errorcluster)  [unwired: 1 out]
            n584 = call <vilib>:"connect.vi"("Use Rack/Slot for S71200/1500"=w1880, "Slot S7 300/400"=w1881, "PLC Type"=PLC_Type."S7 1200" ("PLC Type 2"), "error in (no error)"=w1872, "Rack S7 300/400"=w1882, "timeout [ms]"=1000 ("timeout [ms] 2"), "IP address"=w1875) -> ("error out"=w1885:errorcluster, "S7 Connection out"=w1884:T5)  [unwired: 3 in]
            n585 = for {
              tunnel: w1883 -> [w1893] mode=indexing
              shift-right: [w1891] -> w1878
              shift-left: w1884 -> [w1889]
              tunnel: w1885 -> [w1890]
              tunnel: [w1888] -> w1879
              w1892 = i32[] [0, 0]  # DINT input array
              # "Reset Search and save \nbit on software start"
              n586 = call-poly <vilib>:"write DB.vi"("DINT input array"=w1892, "error in (no error)"=w1890, "Data Block #"=w1893, "S7 Connection in"=w1889) -> ("error out"=w1888:errorcluster, "S7 Connection out"=w1891:T5)  [unwired: 4 in, 2 out]
            }
          }
          frame "Write" {
            w1899 = u16 57 ("Data Block #")
            w1914 = PLC_Comm_State."Read"  # Enum
            n587 = global read "DATA LOG.vi" "OP 50 Outputs"() -> (w1913:bool)
            n588 = case shown="True" w1913 {
              tunnel: w1897 -> [w1926 w1939]
              tunnel: [w1927 w1929] -> w1912
              tunnel: [w1926 w1932] -> w1911
              tunnel: w1896 -> [w1927 w1936]
              frame False {
              }
              frame True {
                w1940 = u16 57  # Data Block #
                n589 = call "PADMINI_AUTO_BARCODE_STATUS 50.vi"("Enum"=enum16{"Read", "Write"}."Read", "error in (no error)"=w1936) -> ("error out"=w1935:errorcluster, "O/P"=w1937:i32[])  [unwired: 8 in]
                n590 = call-poly <vilib>:"write DB.vi"("DINT input array"=w1937, "error in (no error)"=w1935, "Data Block #"=w1940, "S7 Connection in"=w1939) -> ("error out"=w1930:errorcluster, "S7 Connection out"=w1931:T5)  [unwired: 4 in, 2 out]
                n591 = call-poly <vilib>:"write DB.vi"("DINT input array"=i32[] [0] ("Data Byte"), "error in (no error)"=w1930, "Data Block #"=u16 56, "S7 Connection in"=w1931) -> ("error out"=w1929:errorcluster, "S7 Connection out"=w1932:T5)  [unwired: 4 in, 2 out]
                n592 = Unbundle By Name(w1929) -> ("status"=w1928:bool)
                n593 = global write "DATA LOG.vi" "OP 50 Outputs"(w1928) -> ()
              }
            }
            n594 = global read "DATA LOG.vi" "OP 50 reset"() -> (w1910:bool)
            n595 = case shown="True" w1910 {
              tunnel: w1912 -> [w1916 w1925]
              tunnel: [w1916 w1919] -> w1905
              tunnel: w1911 -> [w1917 w1924]
              tunnel: [w1917 w1923] -> w1906
              frame False {
              }
              frame True {
                n596 = call-poly <vilib>:"write DB.vi"("Item offset [byte]"=u16 4 ("Data Block #"), "DINT input array"=i32[] [0], "error in (no error)"=w1925, "Data Block #"=u16 56, "S7 Connection in"=w1924) -> ("error out"=w1919:errorcluster, "S7 Connection out"=w1923:T5)  [unwired: 3 in, 2 out]
                n597 = Unbundle By Name(w1919) -> ("status"=w1918:bool)
                n598 = global write "DATA LOG.vi" "OP 50 reset"(w1918) -> ()
              }
            }
            n599 = global read "DATA LOG.vi" "Auto Cycle On"() -> (w1904:bool)
            n600 = global read "Global 1.vi" "Filtered BARCODE selected"() -> (w1907:string[])
            n601 = Boolean To (0,1)(Boolean=w1904) -> (0, 1=w1903:i16)
            n602 = Build Array(w1903) -> (w1902:i16[])
            n603 = call-poly <vilib>:"write DB.vi"("Item offset [byte]"=u32 20, "DINT input array"=w1902, "error in (no error)"=w1905, "Data Block #"=w1899, "S7 Connection in"=w1906) -> ("error out"=w1908:errorcluster, "S7 Connection out"=w1909:T5)  [unwired: 3 in, 2 out]
            n604 = call-poly <vilib>:"write DB.vi"("Item offset [byte]"=u32 24, "Input STRINGS"=w1907, "error in (no error)"=w1908, "String length reserved in DB (default=254)"=u16 15, "Data Block #"=w1899, "S7 Connection in"=w1909) -> ("error out"=w1895:errorcluster, "S7 Connection out"=w1894:T5)  [unwired: 2 in, 2 out]
          }
          frame "Read" {
            w1953 = u16 56 ("Data Block #")
            w1967 = PLC_Comm_State."Write"  # Enum
            # "OP 50 Read"
            n605 = call-poly <vilib>:"read DB.vi"("error in (no error)"=w1944, "items #"=u16 2 ("Items # [byte]"), "Data Block #"=w1953, "S7 Connection in"=w1941) -> ("error out"=w1965:errorcluster, "DINT result array"=w1961:i32[], "S7 Connection out"=w1964:T5)  [unwired: 5 in]
            n606 = call-poly <vilib>:"read DB.vi"("Item offset [byte]"=u32 8, "error in (no error)"=w1965, "items #"=u16 3 ("Items # [byte]"), "Data Block #"=w1953, "S7 Connection in"=w1964) -> ("error out"=w1959:errorcluster, "REAL result array"=w1963:sgl[], "S7 Connection out"=w1960:T5)  [unwired: 4 in]
            n607 = call-poly <vilib>:"read DB.vi"("Item offset [byte]"=u32 20, "String length reserved in DB (default=254)"=u16 50, "error in (no error)"=w1959, "items #"=u16 1 ("Items # [byte]"), "Data Block #"=w1953, "S7 Connection in"=w1960) -> ("error out"=w1958:errorcluster, "STRING result Array"=w1956:string[], "S7 Connection out"=w1957:T5)  [unwired: 2 in, 1 out]
            n608 = call-poly <vilib>:"read DB.vi"("Item offset [byte]"=u32 72, "String length reserved in DB (default=254)"=u16 10, "error in (no error)"=w1958, "items #"=u16 5 ("Items # [byte]"), "Data Block #"=w1953, "S7 Connection in"=w1957) -> ("error out"=w1966:errorcluster, "STRING result Array"=w1955:string[], "S7 Connection out"=w1942:T5)  [unwired: 2 in, 1 out]
            n609 = Build Array (concatenate)(w1956, w1955) -> (w1962:string[])
            n610 = case shown="No Error" w1966 {
              selector: w1966 -> [w1972 w1977]
              tunnel: w1961 -> [w1976 _]
              tunnel: w1962 -> [w1974 _]
              tunnel: w1963 -> [w1971 _]
              tunnel: [w1970 w1977] -> w1943
              frame No Error {
                w1969 = enum16{"Read", "Write"}."Write" ("Enum")
                n611 = call "PADMINI_AUTO_CYCLE VALUE 50.vi"("Enum"=w1969, "error in (no error)"=w1972, "Input"=w1971) -> ("error out"=w1973:errorcluster)  [unwired: 7 in, 1 out]
                n612 = call "PADMINI_AUTO_BARCODE_STRING 50.vi"("Enum"=w1969, "error in (no error)"=w1973, "Input"=w1974) -> ("error out"=w1975:errorcluster)  [unwired: 7 in, 1 out]
                n613 = call "PADMINI_AUTO_CYCLE STATE 50.vi"("Enum"=w1969, "error in (no error)"=w1975, "Input"=w1976) -> ("error out"=w1970:errorcluster)  [unwired: 7 in, 1 out]
              }
              frame Error {
              }
            }
          }
          frame "Error" {
            w1978 = PLC_Comm_State."Write"  # Enum
            n614 = global write "Global 1.vi" "PLC4 error"(w1979) -> ()
          }
          frame "Disconnect" {
            w1982 = PLC_Comm_State."Disconnect"  # Enum
            w1985 = T5 {"TCP Connection Ref"=refnum, "IP address"="", "timeout ms"=5000, "Connected?"=FALSE, "PLC Type"=enum."S7 1200", "Rack S7 400"=0, "Slot S7 400"=0, "PDU Size"=0, "connection semaphore"=refnum}  # S7 Connection out
            n615 = call <vilib>:"Clear Errors.vi"("error in (no error)"=w1986) -> ("error out"=w1989:errorcluster)  [unwired: 5 in, 1 out]
            n616 = call <vilib>:"disconnect.vi"("error in (no error)"=w1989, "S7 Connection in"=w1987) -> ("error out"=w1988:errorcluster)  [unwired: 8 in, 1 out]
          }
          frame "Write2" {
            # "No Use"
          }
          frame "Write3" {
            # "No Use"
          }
          frame "Read2" {
            # "No Use"
          }
          frame "Read3" {
            # "No Use"
          }
        }
        n617 = Wait (ms)(milliseconds to wait=w1837) -> ()  [unwired: 1 out]
        n618 = call "PADMINI_STOP_ALL.vi"("Enum"=enum16{"Read", "Write"}."Read") -> ("Boolean 2"=w1828:bool)  [unwired: 9 in, 1 out]
        n619 = local read "stop"() -> (w1823:bool)
        n620 = case shown="Error" w1841 {
          selector: w1841 -> [w1844 w1848]
          tunnel: [w1844 w1851] -> w1824
          tunnel: [w1843 w1845] -> w1831
          tunnel: w1836 -> [w1843 _]
          tunnel: [w1842 w1857] -> w1835
          tunnel: w1834 -> [w1842 w1857]
          tunnel: w1830 -> [_ w1855]
          frame No Error {
          }
          frame Error {
            w1846 = PLC_Comm_State."Connect"  # Enum
            w1847 = PLC_Comm_State."Error"  # Enum
            n621 = Unbundle By Name(w1848) -> ("source"=w1856:string)
            n622 = call <userlib>:"Get Strings from Enum__ogtk.vi"("Enum"=w1855) -> ("String Value"=w1854:string)  [unwired: 7 in, 3 out]
            n623 = Concatenate Strings(w1854, "    " ("string"), w1856) -> (w1852:string)
            n624 = Bundle By Name(cluster=w1848, "source"=w1852) -> (w1851:errorcluster)
            n625 = call <vilib>:"Clear Errors.vi"("error in (no error)"=w1848, "specific error code to clear (0: all)"=6002) -> ("specific error cleared?"=w1850:bool)  [unwired: 4 in, 1 out]
            n626 = Select(t=w1846, s=w1850, f=w1847) -> (s? t:f=w1845:T1)
          }
        }
        n627 = Or(x=w1823, y=w1828) -> (x .or. y?=w1826:bool)
        n628 = Select(t=w1829, s=w1826, f=w1831) -> (s? t:f=w1832:T1)
        n629 = Unbundle By Name(w1824) -> ("status"=w1825:bool)
        n630 = Not(x=w1825) -> (.not. x?=w1822:bool)
        n631 = global write "Global 1.vi" "PLC 4"(w1822) -> ()
      }
    }
  }
  n632 = disable-structure shown="Enabled" {
    disable-tunnel: w61 -> [w2010 w2135]
    disable-tunnel: w9 -> [w2003 w2134]
    disable-tunnel: [w1998 w2133] -> w6
    frame Disabled {
      w2000 = TRUE  # Use Rack/Slot for S71200/1500
      w2001 = u8 1  # Slot S7 300/400
      w2002 = u8 0  # Rack S7 300/400
      w2008 = i32[] [0, 0]  # DINT input array
      # "Reset Search and save \nbit on software start"
      n633 = call <vilib>:"connect.vi"("Use Rack/Slot for S71200/1500"=w2000, "Slot S7 300/400"=w2001, "PLC Type"=PLC_Type."S7 1200" ("PLC Type 2"), "error in (no error)"=w2003, "Rack S7 300/400"=w2002, "timeout [ms]"=1000 ("timeout [ms] 2"), "IP address"=w2010) -> ("error out"=w2004:errorcluster, "S7 Connection out"=w2005:T5)  [unwired: 3 in]
      n634 = call-poly <vilib>:"write DB.vi"("DINT input array"=w2008, "error in (no error)"=w2004, "Data Block #"=u16 43, "S7 Connection in"=w2005) -> ("error out"=w2007:errorcluster, "S7 Connection out"=w2006:T5)  [unwired: 4 in, 2 out]
      n635 = while {
        shift-right: [w2017] -> w2011
        shift-left: w2006 -> [w2027]
        shift-right: [w2025] -> w2012
        shift-left: w2007 -> [w2026]
        tunnel: w2010 -> [w2016]
        stop <- w2019 stop-if-true
        # "OP 60"
        n636 = flat-sequence {
          tunnel: [w2030] -> w2023
          tunnel: [w2028] -> w2018
          tunnel: w2026 -> [w2078]
          tunnel: w2027 -> [w2077]
          tunnel: w2016 -> [w2065]
          tunnel: [w2065] -> w2015
          tunnel: [w2106] -> w2025
          tunnel: [w2105] -> w2017
          tunnel: w2023 -> [w2108]
          tunnel: w2018 -> [w2107]
          tunnel: w2015 -> [w2104]
          frame #0 {
            w2061 = u16 44 ("Data Block #")
            w2042 = u16 43 ("Data Block #")
            # "AUTO WRITE"
            n637 = global read "DATA LOG.vi" "OP 60 Outputs"() -> (w2076:bool)
            n638 = case shown="True" w2076 {
              tunnel: w2077 -> [w2089 w2102]
              tunnel: [w2090 w2091] -> w2053
              tunnel: [w2089 w2094] -> w2052
              tunnel: w2078 -> [w2090 w2099]
              frame False {
              }
              frame True {
                w2103 = u16 44  # Data Block #
                n639 = call "PADMINI_AUTO_BARCODE_STATUS 60.vi"("Enum"=enum16{"Read", "Write"}."Read", "error in (no error)"=w2099) -> ("error out"=w2098:errorcluster, "O/P"=w2100:i32[])  [unwired: 8 in]
                n640 = global write "DATA LOG.vi" "OP 60 Outputs"(FALSE) -> ()
                n641 = call-poly <vilib>:"write DB.vi"("DINT input array"=w2100, "error in (no error)"=w2098, "Data Block #"=w2103, "S7 Connection in"=w2102) -> ("error out"=w2092:errorcluster, "S7 Connection out"=w2093:T5)  [unwired: 4 in, 2 out]
                n642 = call-poly <vilib>:"write DB.vi"("DINT input array"=i32[] [0] ("Data Byte"), "error in (no error)"=w2092, "Data Block #"=u16 43, "S7 Connection in"=w2093) -> ("error out"=w2091:errorcluster, "S7 Connection out"=w2094:T5)  [unwired: 4 in, 2 out]
              }
            }
            n643 = global read "DATA LOG.vi" "OP 60 reset"() -> (w2051:bool)
            n644 = global read "DATA LOG.vi" "Auto Cycle On"() -> (w2039:bool)
            n645 = case shown="True" w2051 {
              tunnel: w2053 -> [w2079 w2088]
              tunnel: [w2079 w2087] -> w2054
              tunnel: w2052 -> [w2080 w2086]
              tunnel: [w2080 w2085] -> w2055
              frame False {
              }
              frame True {
                n646 = global write "DATA LOG.vi" "OP 60 reset"(FALSE) -> ()
                n647 = call-poly <vilib>:"write DB.vi"("Item offset [byte]"=u16 4 ("Data Block #"), "DINT input array"=i32[] [0], "error in (no error)"=w2088, "Data Block #"=u16 43, "S7 Connection in"=w2086) -> ("error out"=w2087:errorcluster, "S7 Connection out"=w2085:T5)  [unwired: 3 in, 2 out]
              }
            }
            n648 = Boolean To (0,1)(Boolean=w2039) -> (0, 1=w2038:i16)
            n649 = Build Array(w2038) -> (w2037:i16[])
            n650 = global read "Global 1.vi" "Filtered BARCODE selected"() -> (w2064:string[])
            n651 = call-poly <vilib>:"write DB.vi"("Item offset [byte]"=u32 20, "DINT input array"=w2037, "error in (no error)"=w2054, "Data Block #"=w2061, "S7 Connection in"=w2055) -> ("error out"=w2059:errorcluster, "S7 Connection out"=w2058:T5)  [unwired: 3 in, 2 out]
            n652 = call-poly <vilib>:"write DB.vi"("Item offset [byte]"=u32 24, "Input STRINGS"=w2064, "error in (no error)"=w2059, "String length reserved in DB (default=254)"=u16 15, "Data Block #"=w2061, "S7 Connection in"=w2058) -> ("error out"=w2056:errorcluster, "S7 Connection out"=w2057:T5)  [unwired: 2 in, 2 out]
            n653 = call-poly <vilib>:"read DB.vi"("Item offset [byte]"=u32 8, "error in (no error)"=w2056, "items #"=u16 6 ("Items # [byte]"), "Data Block #"=w2042, "S7 Connection in"=w2057) -> ("error out"=w2068:errorcluster, "REAL result array"=w2066:sgl[], "S7 Connection out"=w2074:T5)  [unwired: 4 in]
            n654 = call "PADMINI_AUTO_CYCLE VALUE 60.vi"("Enum"=enum16{"Read", "Write"}."Write", "error in (no error)"=w2068, "Input"=w2066) -> ("error out"=w2067:errorcluster)  [unwired: 7 in, 1 out]
            n655 = call-poly <vilib>:"read DB.vi"("Item offset [byte]"=u32 32, "String length reserved in DB (default=254)"=u16 50, "error in (no error)"=w2067, "items #"=u16 1 ("Items # [byte]"), "Data Block #"=w2042, "S7 Connection in"=w2074) -> ("error out"=w2046:errorcluster, "STRING result Array"=w2044:string[], "S7 Connection out"=w2045:T5)  [unwired: 2 in, 1 out]
            n656 = call-poly <vilib>:"read DB.vi"("Item offset [byte]"=u32 84, "String length reserved in DB (default=254)"=u16 10, "error in (no error)"=w2046, "items #"=u16 7 ("Items # [byte]"), "Data Block #"=w2042, "S7 Connection in"=w2045) -> ("error out"=w2047:errorcluster, "STRING result Array"=w2050:string[], "S7 Connection out"=w2031:T5)  [unwired: 2 in, 1 out]
            n657 = Build Array (concatenate)(w2044, w2050) -> (w2043:string[])
            n658 = call "PADMINI_AUTO_BARCODE_STRING 60.vi"("Enum"=enum16{"Read", "Write"}."Write", "error in (no error)"=w2047, "Input"=w2043) -> ("error out"=w2029:errorcluster)  [unwired: 7 in, 1 out]
            n659 = call-poly <vilib>:"read DB.vi"("error in (no error)"=w2029, "items #"=u16 2 ("Items # [byte]"), "Data Block #"=u16 43, "S7 Connection in"=w2031) -> ("error out"=w2036:errorcluster, "DINT result array"=w2034:i32[], "S7 Connection out"=w2030:T5)  [unwired: 5 in]
            n660 = call "PADMINI_AUTO_CYCLE STATE 60.vi"("Enum"=enum16{"Read", "Write"}."Write", "error in (no error)"=w2036, "Input"=w2034) -> ("error out"=w2028:errorcluster)  [unwired: 7 in, 1 out]
          }
          frame #1 {
            # "RECONNECT"
            n661 = case shown="Error" w2107 {
              selector: w2107 -> [w2112 w2113]
              tunnel: [w2111 w2117] -> w2105
              tunnel: [w2112 w2118] -> w2106
              tunnel: w2108 -> [w2111 w2116]
              tunnel: w2104 -> [_ w2115]
              frame No Error {
              }
              frame Error {
                n662 = Unbundle By Name(w2113) -> ("code"=w2114:i32)
                n663 = call <vilib>:"Clear Errors.vi"("error in (no error)"=w2113) -> ("error out"=w2119:errorcluster)  [unwired: 5 in, 1 out]
                n664 = case shown="0, Default" w2114 {
                  tunnel: w2119 -> [w2121 w2132]
                  tunnel: [w2121 w2130] -> w2118
                  tunnel: [w2122 w2129] -> w2117
                  tunnel: w2116 -> [w2122 w2126]
                  tunnel: w2115 -> [_ w2125]
                  tunnel: w2113 -> [w2120 _]
                  frame 0, Default {
                    n665 = global write "Global 1.vi" "PLC5 error"(w2120) -> ()
                  }
                  frame 1, 66 {
                    n666 = call <vilib>:"disconnect.vi"("error in (no error)"=w2132, "S7 Connection in"=w2126) -> ("error out"=w2131:errorcluster)  [unwired: 8 in, 1 out]
                    n667 = call <vilib>:"Clear Errors.vi"("error in (no error)"=w2131) -> ("error out"=w2128:errorcluster)  [unwired: 5 in, 1 out]
                    n668 = call <vilib>:"connect.vi"("Use Rack/Slot for S71200/1500"=TRUE, "Slot S7 300/400"=u8 1, "PLC Type"=PLC_Type."S7 1200" ("PLC Type 2"), "error in (no error)"=w2128, "IP address"=w2125) -> ("error out"=w2130:errorcluster, "S7 Connection out"=w2129:T5)  [unwired: 5 in]
                  }
                }
              }
            }
            n669 = Unbundle By Name(w2107) -> ("status"=w2110:bool)
            n670 = Not(x=w2110) -> (.not. x?=w2109:bool)
            "PLC 5" <- w2109
            n671 = global write "Global 1.vi" "PLC 5"(w2109) -> ()
          }
        }
        n672 = call "PADMINI_STOP_ALL.vi"("Enum"=enum16{"Read", "Write"}."Read") -> ("Boolean 2"=w2021:bool)  [unwired: 9 in, 1 out]
        n673 = local read "stop"() -> (w2020:bool)
        n674 = Or(x=w2020, y=w2021) -> (x .or. y?=w2019:bool)
        n675 = Wait (ms)(milliseconds to wait=u32 1200) -> ()  [unwired: 1 out]
      }
      n676 = call <vilib>:"Clear Errors.vi"("error in (no error)"=w2012) -> ("error out"=w1999:errorcluster)  [unwired: 5 in, 1 out]
      n677 = call <vilib>:"disconnect.vi"("error in (no error)"=w1999, "S7 Connection in"=w2011) -> ("error out"=w1998:errorcluster)  [unwired: 8 in, 1 out]
    }
    frame Enabled {
      w2136 = PLC_Comm_State."Int"  # Enum
      n678 = while {
        shift-right: [w2148] -> _
        shift-left: w2136 -> [w2156]
        shift-right: [w2140] -> w2133
        shift-left: w2134 -> [w2155]
        shift-right: [w2151] -> _
        shift-left: _ -> [w2154]
        tunnel: w2135 -> [w2137]
        stop <- w2149 stop-if-true
        w2145 = PLC_Comm_State."Disconnect"  # Enum
        w2153 = u32 800  # milliseconds to wait
        # "Int-->Write-->Read---if--Error-->reconnect\n               ^------v                                       v\n                ^------------------------------v"
        # "OP 60"
        n679 = case shown="\"Error\"" w2156 {
          selector: w2156 -> [w2176 w2193 w2231 w2285 w2297 w2301 _ _ _ _]
          tunnel: [w2181 w2195 w2210 w2260 w2298 w2306 w2308 w2311 w2313 w2315] -> w2157
          tunnel: [w2182 w2194 w2213 w2257 w2299 w2303 w2309 w2310 w2312 w2314] -> w2150
          tunnel: w2155 -> [w2179 w2190 w2211 w2259 w2295 w2304 w2308 w2311 w2313 w2315]
          tunnel: w2154 -> [w2177 _ w2212 w2258 w2299 w2305 w2309 w2310 w2312 w2314]
          tunnel: [w2175 w2192 w2230 w2284 w2296 w2300 _ _ _ _] -> w2152
          tunnel: [_ _ _ _ _ TRUE _ _ _ _] -> w2149
          tunnel: [w2176 w2193 w2231 w2285 w2297 w2301 _ _ _ _] -> w2146
          tunnel: w2137 -> [w2174 w2191 _ _ _ _ _ _ _ _]
          frame "Connect" {
            w2175 = PLC_Comm_State."Write"  # Enum
            w2187 = TRUE  # Use Rack/Slot for S71200/1500
            w2186 = u8 1  # Slot S7 300/400
            w2184 = u8 0  # Rack S7 300/400
            # "Reconect"
            n680 = call <vilib>:"disconnect.vi"("error in (no error)"=w2179, "S7 Connection in"=w2177) -> ("error out"=w2180:errorcluster)  [unwired: 8 in, 1 out]
            n681 = call <vilib>:"Clear Errors.vi"("error in (no error)"=w2180) -> ("error out"=w2178:errorcluster)  [unwired: 5 in, 1 out]
            n682 = call <vilib>:"connect.vi"("Use Rack/Slot for S71200/1500"=w2187, "Slot S7 300/400"=w2186, "PLC Type"=PLC_Type."S7 1200" ("PLC Type 2"), "error in (no error)"=w2178, "Rack S7 300/400"=w2184, "timeout [ms]"=1000 ("timeout [ms] 2"), "IP address"=w2174) -> ("error out"=w2181:errorcluster, "S7 Connection out"=w2182:T5)  [unwired: 3 in]
          }
          frame "Int" {
            w2192 = PLC_Comm_State."Write"  # Enum
            w2196 = TRUE  # Use Rack/Slot for S71200/1500
            w2197 = u8 1  # Slot S7 300/400
            w2198 = u8 0  # Rack S7 300/400
            w2199 = u16[] [43]  # Data Block #
            # "Initialize and set first bits"
            n683 = call "Stall Data Flow.vim"("value in"=w2190, "milliseconds to wait"=u32 516) -> ("value out"=w2189:errorcluster)  [unwired: 1 out]
            n684 = call <vilib>:"connect.vi"("Use Rack/Slot for S71200/1500"=w2196, "Slot S7 300/400"=w2197, "PLC Type"=PLC_Type."S7 1200" ("PLC Type 2"), "error in (no error)"=w2189, "Rack S7 300/400"=w2198, "timeout [ms]"=1000 ("timeout [ms] 2"), "IP address"=w2191) -> ("error out"=w2201:errorcluster, "S7 Connection out"=w2200:T5)  [unwired: 3 in]
            n685 = for {
              tunnel: w2199 -> [w2209] mode=indexing
              shift-right: [w2207] -> w2194
              shift-left: w2200 -> [w2205]
              tunnel: w2201 -> [w2206]
              tunnel: [w2204] -> w2195
              w2208 = i32[] [0, 0]  # DINT input array
              # "Reset Search and save \nbit on software start"
              n686 = call-poly <vilib>:"write DB.vi"("DINT input array"=w2208, "error in (no error)"=w2206, "Data Block #"=w2209, "S7 Connection in"=w2205) -> ("error out"=w2204:errorcluster, "S7 Connection out"=w2207:T5)  [unwired: 4 in, 2 out]
            }
          }
          frame "Write" {
            w2215 = u16 44 ("Data Block #")
            w2230 = PLC_Comm_State."Read"  # Enum
            n687 = global read "DATA LOG.vi" "OP 60 Outputs"() -> (w2229:bool)
            n688 = case shown="True" w2229 {
              tunnel: w2212 -> [w2242 w2255]
              tunnel: [w2243 w2245] -> w2223
              tunnel: [w2242 w2248] -> w2222
              tunnel: w2211 -> [w2243 w2252]
              frame False {
              }
              frame True {
                w2256 = u16 44  # Data Block #
                n689 = call "PADMINI_AUTO_BARCODE_STATUS 60.vi"("Enum"=enum16{"Read", "Write"}."Read", "error in (no error)"=w2252) -> ("error out"=w2251:errorcluster, "O/P"=w2253:i32[])  [unwired: 8 in]
                n690 = call-poly <vilib>:"write DB.vi"("DINT input array"=w2253, "error in (no error)"=w2251, "Data Block #"=w2256, "S7 Connection in"=w2255) -> ("error out"=w2246:errorcluster, "S7 Connection out"=w2247:T5)  [unwired: 4 in, 2 out]
                n691 = call-poly <vilib>:"write DB.vi"("DINT input array"=i32[] [0] ("Data Byte"), "error in (no error)"=w2246, "Data Block #"=u16 43, "S7 Connection in"=w2247) -> ("error out"=w2245:errorcluster, "S7 Connection out"=w2248:T5)  [unwired: 4 in, 2 out]
                n692 = Unbundle By Name(w2245) -> ("status"=w2244:bool)
                n693 = global write "DATA LOG.vi" "OP 60 Outputs"(w2244) -> ()
              }
            }
            n694 = global read "DATA LOG.vi" "OP 60 reset"() -> (w2221:bool)
            n695 = global read "DATA LOG.vi" "Auto Cycle On"() -> (w2220:bool)
            n696 = case shown="True" w2221 {
              tunnel: w2223 -> [w2232 w2241]
              tunnel: [w2232 w2235] -> w2224
              tunnel: w2222 -> [w2233 w2240]
              tunnel: [w2233 w2239] -> w2225
              frame False {
              }
              frame True {
                n697 = call-poly <vilib>:"write DB.vi"("Item offset [byte]"=u16 4 ("Data Block #"), "DINT input array"=i32[] [0], "error in (no error)"=w2241, "Data Block #"=u16 43, "S7 Connection in"=w2240) -> ("error out"=w2235:errorcluster, "S7 Connection out"=w2239:T5)  [unwired: 3 in, 2 out]
                n698 = Unbundle By Name(w2235) -> ("status"=w2234:bool)
                n699 = global write "DATA LOG.vi" "OP 60 reset"(w2234) -> ()
              }
            }
            n700 = Boolean To (0,1)(Boolean=w2220) -> (0, 1=w2219:i16)
            n701 = Build Array(w2219) -> (w2218:i16[])
            n702 = global read "Global 1.vi" "Filtered BARCODE selected"() -> (w2228:string[])
            n703 = call-poly <vilib>:"write DB.vi"("Item offset [byte]"=u32 20, "DINT input array"=w2218, "error in (no error)"=w2224, "Data Block #"=w2215, "S7 Connection in"=w2225) -> ("error out"=w2227:errorcluster, "S7 Connection out"=w2226:T5)  [unwired: 3 in, 2 out]
            n704 = call-poly <vilib>:"write DB.vi"("Item offset [byte]"=u32 24, "Input STRINGS"=w2228, "error in (no error)"=w2227, "String length reserved in DB (default=254)"=u16 15, "Data Block #"=w2215, "S7 Connection in"=w2226) -> ("error out"=w2210:errorcluster, "S7 Connection out"=w2213:T5)  [unwired: 2 in, 2 out]
          }
          frame "Read" {
            w2266 = u16 43 ("Data Block #")
            w2284 = PLC_Comm_State."Write"  # Enum
            n705 = call-poly <vilib>:"read DB.vi"("Item offset [byte]"=u32 8, "error in (no error)"=w2259, "items #"=u16 6 ("Items # [byte]"), "Data Block #"=w2266, "S7 Connection in"=w2258) -> ("error out"=w2280:errorcluster, "REAL result array"=w2283:sgl[], "S7 Connection out"=w2281:T5)  [unwired: 4 in]
            n706 = call-poly <vilib>:"read DB.vi"("Item offset [byte]"=u32 32, "String length reserved in DB (default=254)"=u16 50, "error in (no error)"=w2280, "items #"=u16 1 ("Items # [byte]"), "Data Block #"=w2266, "S7 Connection in"=w2281) -> ("error out"=w2277:errorcluster, "STRING result Array"=w2275:string[], "S7 Connection out"=w2276:T5)  [unwired: 2 in, 1 out]
            n707 = call-poly <vilib>:"read DB.vi"("Item offset [byte]"=u32 84, "String length reserved in DB (default=254)"=u16 10, "error in (no error)"=w2277, "items #"=u16 7 ("Items # [byte]"), "Data Block #"=w2266, "S7 Connection in"=w2276) -> ("error out"=w2278:errorcluster, "STRING result Array"=w2279:string[], "S7 Connection out"=w2272:T5)  [unwired: 2 in, 1 out]
            n708 = Build Array (concatenate)(w2275, w2279) -> (w2282:string[])
            n709 = call-poly <vilib>:"read DB.vi"("error in (no error)"=w2278, "items #"=u16 2 ("Items # [byte]"), "Data Block #"=u16 43, "S7 Connection in"=w2272) -> ("error out"=w2274:errorcluster, "DINT result array"=w2273:i32[], "S7 Connection out"=w2257:T5)  [unwired: 5 in]
            n710 = case shown="No Error" w2274 {
              selector: w2274 -> [w2287 w2294]
              tunnel: w2273 -> [w2286 _]
              tunnel: w2282 -> [w2293 _]
              tunnel: w2283 -> [w2291 _]
              tunnel: [w2288 w2294] -> w2260
              frame No Error {
                w2292 = enum16{"Read", "Write"}."Write" ("Enum")
                n711 = call "PADMINI_AUTO_BARCODE_STRING 60.vi"("Enum"=w2292, "error in (no error)"=w2287, "Input"=w2293) -> ("error out"=w2290:errorcluster)  [unwired: 7 in, 1 out]
                n712 = call "PADMINI_AUTO_CYCLE VALUE 60.vi"("Enum"=w2292, "error in (no error)"=w2290, "Input"=w2291) -> ("error out"=w2289:errorcluster)  [unwired: 7 in, 1 out]
                n713 = call "PADMINI_AUTO_CYCLE STATE 60.vi"("Enum"=w2292, "error in (no error)"=w2289, "Input"=w2286) -> ("error out"=w2288:errorcluster)  [unwired: 7 in, 1 out]
              }
              frame Error {
              }
            }
          }
          frame "Error" {
            w2296 = PLC_Comm_State."Write"  # Enum
            n714 = global write "Global 1.vi" "PLC5 error"(w2295) -> ()
            n715 = call <vilib>:"Clear Errors.vi"("error in (no error)"=w2295) -> ("error out"=w2298:errorcluster)  [unwired: 5 in, 1 out]
          }
          frame "Disconnect" {
            w2300 = PLC_Comm_State."Disconnect"  # Enum
            w2303 = T5 {"TCP Connection Ref"=refnum, "IP address"="", "timeout ms"=5000, "Connected?"=FALSE, "PLC Type"=enum."S7 1200", "Rack S7 400"=0, "Slot S7 400"=0, "PDU Size"=0, "connection semaphore"=refnum}  # S7 Connection out
            n716 = call <vilib>:"Clear Errors.vi"("error in (no error)"=w2304) -> ("error out"=w2307:errorcluster)  [unwired: 5 in, 1 out]
            n717 = call <vilib>:"disconnect.vi"("error in (no error)"=w2307, "S7 Connection in"=w2305) -> ("error out"=w2306:errorcluster)  [unwired: 8 in, 1 out]
          }
          frame "Write2" {
            # "No Use"
          }
          frame "Write3" {
            # "No Use"
          }
          frame "Read2" {
            # "No Use"
          }
          frame "Read3" {
            # "No Use"
          }
        }
        n718 = Wait (ms)(milliseconds to wait=w2153) -> ()  [unwired: 1 out]
        n719 = call "PADMINI_STOP_ALL.vi"("Enum"=enum16{"Read", "Write"}."Read") -> ("Boolean 2"=w2144:bool)  [unwired: 9 in, 1 out]
        n720 = local read "stop"() -> (w2139:bool)
        n721 = case shown="Error" w2157 {
          selector: w2157 -> [w2160 w2163]
          tunnel: [w2160 w2167] -> w2140
          tunnel: [w2159 w2162] -> w2147
          tunnel: w2152 -> [w2159 _]
          tunnel: [w2158 w2173] -> w2151
          tunnel: w2150 -> [w2158 w2173]
          tunnel: w2146 -> [_ w2171]
          frame No Error {
          }
          frame Error {
            w2164 = PLC_Comm_State."Connect"  # Enum
            w2161 = PLC_Comm_State."Error"  # Enum
            n722 = Unbundle By Name(w2163) -> ("source"=w2172:string)
            n723 = call <userlib>:"Get Strings from Enum__ogtk.vi"("Enum"=w2171) -> ("String Value"=w2170:string)  [unwired: 7 in, 3 out]
            n724 = Concatenate Strings(w2170, "    " ("string"), w2172) -> (w2168:string)
            n725 = Bundle By Name(cluster=w2163, "source"=w2168) -> (w2167:errorcluster)
            n726 = call <vilib>:"Clear Errors.vi"("error in (no error)"=w2163, "specific error code to clear (0: all)"=6002) -> ("specific error cleared?"=w2166:bool)  [unwired: 4 in, 1 out]
            n727 = Select(t=w2164, s=w2166, f=w2161) -> (s? t:f=w2162:T1)
          }
        }
        n728 = Or(x=w2139, y=w2144) -> (x .or. y?=w2142:bool)
        n729 = Select(t=w2145, s=w2142, f=w2147) -> (s? t:f=w2148:T1)
        n730 = Unbundle By Name(w2140) -> ("status"=w2141:bool)
        n731 = Not(x=w2141) -> (.not. x?=w2138:bool)
        n732 = global write "Global 1.vi" "PLC 5"(w2138) -> ()
      }
    }
  }
  n733 = disable-structure shown="Enabled" {
    disable-tunnel: [w2329 _] -> w117
    disable-tunnel: [w2326 _] -> w106
    disable-tunnel: w82 -> [w2325 w2391]
    disable-tunnel: w9 -> [w2319 w2390]
    frame Disabled {
      n734 = call <vilib>:"connect.vi"("Use Rack/Slot for S71200/1500"=TRUE, "Slot S7 300/400"=u8 1, "PLC Type"=PLC_Type."S7 1200" ("PLC Type 2"), "error in (no error)"=w2319, "Rack S7 300/400"=u8 0, "timeout [ms]"=1000, "IP address"=w2325) -> ("error out"=w2321:errorcluster, "S7 Connection out"=w2320:T5)  [unwired: 3 in]
      n735 = for {
        tunnel: u16[] [83, 94] ("Data Block #") -> [w2335] mode=indexing
        shift-right: [w2333] -> w2323
        shift-left: w2320 -> [w2330]
        tunnel: w2321 -> [w2331]
        tunnel: [w2332] -> w2322
        w2334 = i32[] [0, 0]  # DINT input array
        # "Reset Search and save \nbit on software start"
        n736 = call-poly <vilib>:"write DB.vi"("DINT input array"=w2334, "error in (no error)"=w2331, "Data Block #"=w2335, "S7 Connection in"=w2330) -> ("error out"=w2332:errorcluster, "S7 Connection out"=w2333:T5)  [unwired: 4 in, 2 out]
      }
      n737 = while {
        shift-right: [w2338] -> w2326
        shift-left: w2323 -> [w2348]
        shift-right: [w2346] -> w2329
        shift-left: w2322 -> [w2347]
        tunnel: w2325 -> [w2336]
        stop <- w2341 stop-if-true
        # "OP 10 AND 20"
        n738 = flat-sequence {
          tunnel: [w2351] -> w2340
          tunnel: [w2357] -> w2339
          tunnel: w2347 -> [w2358]
          tunnel: w2348 -> [w2359]
          tunnel: [w2356] -> w2337
          tunnel: w2336 -> [w2356]
          tunnel: [w2363] -> w2346
          tunnel: [w2362] -> w2338
          tunnel: w2340 -> [w2364]
          tunnel: w2339 -> [w2360]
          tunnel: w2337 -> [w2361]
          frame #0 {
            # "NEW CHANGES"
            n739 = call "PLC_OP10_Write.vi"("error in (no error)"=w2358, "S7 Connection in"=w2359) -> ("error out"=w2354:errorcluster, "S7 Connection out"=w2355:T5)  [unwired: 8 in]
            n740 = call "PLC_OP10_Read.vi"("error in (no error)"=w2354, "S7 Connection in"=w2355) -> ("error out"=w2353:errorcluster, "S7 Connection out"=w2352:T5)  [unwired: 8 in]
            n741 = call "PLC_OP20_Write.vi"("error in (no error)"=w2353, "S7 Connection in"=w2352) -> ("error out"=w2349:errorcluster, "S7 Connection out"=w2350:T5)  [unwired: 8 in]
            n742 = call "PLC_OP20_Read.vi"("error in (no error)"=w2349, "S7 Connection in"=w2350) -> ("error out"=w2357:errorcluster, "S7 Connection out 2"=w2351:T5)  [unwired: 8 in]
          }
          frame #1 {
            # "RECONNECT"
            n743 = case shown="Error" w2360 {
              selector: w2360 -> [w2368 w2370]
              tunnel: [w2367 w2373] -> w2362
              tunnel: [w2368 w2374] -> w2363
              tunnel: w2364 -> [w2367 w2372]
              tunnel: w2361 -> [_ w2371]
              frame No Error {
              }
              frame Error {
                n744 = Unbundle By Name(w2370) -> ("code"=w2369:i32)
                n745 = case shown="1, 66" w2369 {
                  tunnel: w2370 -> [w2375 w2388]
                  tunnel: [w2376 w2386] -> w2374
                  tunnel: [w2377 w2385] -> w2373
                  tunnel: w2372 -> [w2377 w2382]
                  tunnel: w2371 -> [_ w2381]
                  frame 0, Default {
                    n746 = call <vilib>:"Clear Errors.vi"("error in (no error)"=w2375) -> ("error out"=w2376:errorcluster)  [unwired: 5 in, 1 out]
                    n747 = global write "Global 1.vi" "PLC1 error"(w2375) -> ()
                  }
                  frame 1, 66 {
                    w2380 = 1000  # timeout [ms]
                    n748 = call <vilib>:"Clear Errors.vi"("error in (no error)"=w2388) -> ("error out"=w2389:errorcluster)  [unwired: 5 in, 1 out]
                    n749 = call <vilib>:"disconnect.vi"("error in (no error)"=w2389, "S7 Connection in"=w2382) -> ("error out"=w2387:errorcluster)  [unwired: 8 in, 1 out]
                    n750 = call <vilib>:"Clear Errors.vi"("error in (no error)"=w2387) -> ("error out"=w2384:errorcluster)  [unwired: 5 in, 1 out]
                    n751 = call <vilib>:"connect.vi"("Use Rack/Slot for S71200/1500"=TRUE, "Slot S7 300/400"=u8 1, "PLC Type"=PLC_Type."S7 1200" ("PLC Type 2"), "error in (no error)"=w2384, "timeout [ms]"=w2380, "IP address"=w2381) -> ("error out"=w2386:errorcluster, "S7 Connection out"=w2385:T5)  [unwired: 4 in]
                  }
                }
              }
            }
            n752 = Unbundle By Name(w2360) -> ("status"=w2366:bool)
            n753 = Not(x=w2366) -> (.not. x?=w2365:bool)
            "PLC 1" <- w2365
            n754 = global write "Global 1.vi" "PLC 1"(w2365) -> ()
          }
        }
        n755 = call "PADMINI_STOP_ALL.vi"("Enum"=enum16{"Read", "Write"}."Read") -> ("Boolean 2"=w2343:bool)  [unwired: 9 in, 1 out]
        n756 = Wait (ms)(milliseconds to wait=u32 1200) -> ()  [unwired: 1 out]
        n757 = Or(x="stop", y=w2343) -> (x .or. y?=w2341:bool)
      }
    }
    frame Enabled {
      w2392 = PLC_Comm_State."Int"  # Enum
      n758 = while {
        shift-right: [w2404] -> _
        shift-left: w2392 -> [w2412]
        shift-right: [w2396] -> _
        shift-left: w2390 -> [w2411]
        shift-right: [w2407] -> _
        shift-left: _ -> [w2410]
        tunnel: w2391 -> [w2393]
        stop <- w2405 stop-if-true
        w2401 = PLC_Comm_State."Disconnect"  # Enum
        w2409 = u32 800  # milliseconds to wait
        # "Int-->Write-->Read---if--Error-->reconnect\n               ^------v                                       v\n                ^------------------------------v"
        # "OP 10-20"
        n759 = case shown="\"Connect\"" w2412 {
          selector: w2412 -> [w2432 w2447 w2469 w2474 w2481 w2486 w2490 w2494 _ _]
          tunnel: [w2437 w2450 w2466 w2470 w2478 w2484 w2491 w2499 w2502 w2504] -> w2413
          tunnel: [w2438 w2449 w2464 w2472 w2476 w2482 w2492 w2496 w2501 w2503] -> w2406
          tunnel: w2411 -> [w2435 w2448 w2467 w2471 w2479 w2485 w2488 w2497 w2502 w2504]
          tunnel: w2410 -> [w2433 _ w2465 w2473 w2477 w2483 w2492 w2498 w2501 w2503]
          tunnel: [w2431 w2446 w2468 w2475 w2480 w2487 w2489 w2493 _ _] -> w2408
          tunnel: [_ _ _ _ _ _ _ TRUE _ _] -> w2405
          tunnel: [w2432 w2447 w2469 w2474 w2481 w2486 w2490 w2494 _ _] -> w2402
          tunnel: w2393 -> [w2430 w2445 _ _ _ _ _ _ _ _]
          frame "Connect" {
            w2431 = PLC_Comm_State."Write"  # Enum
            w2443 = TRUE  # Use Rack/Slot for S71200/1500
            w2442 = u8 1  # Slot S7 300/400
            w2440 = u8 0  # Rack S7 300/400
            # "Reconect"
            n760 = call <vilib>:"disconnect.vi"("error in (no error)"=w2435, "S7 Connection in"=w2433) -> ("error out"=w2436:errorcluster)  [unwired: 8 in, 1 out]
            n761 = call <vilib>:"Clear Errors.vi"("error in (no error)"=w2436) -> ("error out"=w2434:errorcluster)  [unwired: 5 in, 1 out]
            n762 = call <vilib>:"connect.vi"("Use Rack/Slot for S71200/1500"=w2443, "Slot S7 300/400"=w2442, "PLC Type"=PLC_Type."S7 1200" ("PLC Type 2"), "error in (no error)"=w2434, "Rack S7 300/400"=w2440, "timeout [ms]"=1000 ("timeout [ms] 2"), "IP address"=w2430) -> ("error out"=w2437:errorcluster, "S7 Connection out"=w2438:T5)  [unwired: 3 in]
          }
          frame "Int" {
            w2446 = PLC_Comm_State."Write"  # Enum
            w2451 = TRUE  # Use Rack/Slot for S71200/1500
            w2452 = u8 1  # Slot S7 300/400
            w2453 = u8 0  # Rack S7 300/400
            # "Initialize and set first bits"
            n763 = call <vilib>:"connect.vi"("Use Rack/Slot for S71200/1500"=w2451, "Slot S7 300/400"=w2452, "PLC Type"=PLC_Type."S7 1200" ("PLC Type 2"), "error in (no error)"=w2448, "Rack S7 300/400"=w2453, "timeout [ms]"=1000 ("timeout [ms] 2"), "IP address"=w2445) -> ("error out"=w2455:errorcluster, "S7 Connection out"=w2454:T5)  [unwired: 3 in]
            n764 = for {
              tunnel: u16[] [83, 94] ("Data Block #") -> [w2463] mode=indexing
              shift-right: [w2461] -> w2449
              shift-left: w2454 -> [w2459]
              tunnel: w2455 -> [w2460]
              tunnel: [w2458] -> w2450
              w2462 = i32[] [0, 0]  # DINT input array
              # "Reset Search and save \nbit on software start"
              n765 = call-poly <vilib>:"write DB.vi"("DINT input array"=w2462, "error in (no error)"=w2460, "Data Block #"=w2463, "S7 Connection in"=w2459) -> ("error out"=w2458:errorcluster, "S7 Connection out"=w2461:T5)  [unwired: 4 in, 2 out]
            }
          }
          frame "Write" {
            w2468 = PLC_Comm_State."Write2"  # Enum
            # "OP 10 Write"
            n766 = call "PLC_OP10_Write.vi"("S7 Connection in"=w2465, "error in (no error)"=w2467) -> ("S7 Connection out"=w2464:T5, "error out"=w2466:errorcluster)  [unwired: 12 in]
          }
          frame "Write2" {
            w2475 = PLC_Comm_State."Read"  # Enum
            # "op 20 wirte 2"
            n767 = call "PLC_OP20_Write.vi"("S7 Connection in"=w2473, "error in (no error)"=w2471) -> ("S7 Connection out"=w2472:T5, "error out"=w2470:errorcluster)  [unwired: 7 in]
          }
          frame "Read" {
            w2480 = PLC_Comm_State."Read2"  # Enum
            # "OP10 read"
            n768 = call "PLC_OP10_Read.vi"("error in (no error)"=w2479, "S7 Connection in"=w2477) -> ("error out"=w2478:errorcluster, "S7 Connection out"=w2476:T5)  [unwired: 8 in]
          }
          frame "Read2" {
            w2487 = PLC_Comm_State."Write"  # Enum
            # "Op20 Read2"
            n769 = call "PLC_OP20_Read.vi"("error in (no error)"=w2485, "S7 Connection in"=w2483) -> ("error out"=w2484:errorcluster, "S7 Connection out 2"=w2482:T5)  [unwired: 8 in]
          }
          frame "Error" {
            w2489 = PLC_Comm_State."Write"  # Enum
            n770 = global write "Global 1.vi" "PLC1 error"(w2488) -> ()
            n771 = call <vilib>:"Clear Errors.vi"("error in (no error)"=w2488) -> ("error out"=w2491:errorcluster)  [unwired: 5 in, 1 out]
          }
          frame "Disconnect" {
            w2493 = PLC_Comm_State."Disconnect"  # Enum
            w2496 = T5 {"TCP Connection Ref"=refnum, "IP address"="", "timeout ms"=5000, "Connected?"=FALSE, "PLC Type"=enum."S7 1200", "Rack S7 400"=0, "Slot S7 400"=0, "PDU Size"=0, "connection semaphore"=refnum}  # S7 Connection out
            n772 = call <vilib>:"Clear Errors.vi"("error in (no error)"=w2497) -> ("error out"=w2500:errorcluster)  [unwired: 5 in, 1 out]
            n773 = call <vilib>:"disconnect.vi"("error in (no error)"=w2500, "S7 Connection in"=w2498) -> ("error out"=w2499:errorcluster)  [unwired: 8 in, 1 out]
          }
          frame "Write3" {
            # "No Use"
          }
          frame "Read3" {
            # "No Use"
          }
        }
        n774 = Wait (ms)(milliseconds to wait=w2409) -> ()  [unwired: 1 out]
        n775 = call "PADMINI_STOP_ALL.vi"("Enum"=enum16{"Read", "Write"}."Read") -> ("Boolean 2"=w2400:bool)  [unwired: 9 in, 1 out]
        n776 = local read "stop"() -> (w2395:bool)
        n777 = case shown="Error" w2413 {
          selector: w2413 -> [w2416 w2421]
          tunnel: [w2416 w2423] -> w2396
          tunnel: [w2415 w2417] -> w2403
          tunnel: w2408 -> [w2415 _]
          tunnel: [w2414 w2429] -> w2407
          tunnel: w2406 -> [w2414 w2429]
          tunnel: w2402 -> [_ w2427]
          frame No Error {
          }
          frame Error {
            w2419 = PLC_Comm_State."Connect"  # Enum
            w2418 = PLC_Comm_State."Error"  # Enum
            n778 = Unbundle By Name(w2421) -> ("source"=w2428:string)
            n779 = call <userlib>:"Get Strings from Enum__ogtk.vi"("Enum"=w2427) -> ("String Value"=w2426:string)  [unwired: 7 in, 3 out]
            n780 = call <vilib>:"Clear Errors.vi"("error in (no error)"=w2421, "specific error code to clear (0: all)"=6002) -> ("specific error cleared?"=w2420:bool)  [unwired: 4 in, 1 out]
            n781 = Concatenate Strings(w2426, "    " ("string"), w2428) -> (w2424:string)
            n782 = Bundle By Name(cluster=w2421, "source"=w2424) -> (w2423:errorcluster)
            n783 = Select(t=w2419, s=w2420, f=w2418) -> (s? t:f=w2417:T1)
          }
        }
        n784 = Or(x=w2395, y=w2400) -> (x .or. y?=w2398:bool)
        n785 = Select(t=w2401, s=w2398, f=w2403) -> (s? t:f=w2404:T1)
        n786 = Unbundle By Name(w2396) -> ("status"=w2397:bool)
        n787 = Not(x=w2397) -> (.not. x?=w2394:bool)
        n788 = global write "Global 1.vi" "PLC 1"(w2394) -> ()
      }
    }
  }
  n789 = while {
    shift-right: [w2515] -> _
    shift-left: w1 -> [w2524]
    shift-right: [w2505] -> w84
    shift-left: w9 -> [w2523]
    shift-right: [w2518] -> _
    shift-left: _ -> [w2522]
    tunnel: w83 -> [w2521]
    stop <- w2516 stop-if-true
    w2512 = PLC_Comm_State."Disconnect"  # Enum
    w2520 = u32 800  # milliseconds to wait
    # "Int-->Write-->Read---if--Error-->reconnect\n               ^------v                                       v\n                ^------------------------------v"
    # "OP 30"
    n790 = case shown="\"Error\"" w2524 {
      selector: w2524 -> [w2543 w2559 w2583 w2589 w2592 w2596 _ _ _ _]
      tunnel: [w2548 w2563 w2578 w2585 w2593 w2601 w2603 w2606 w2608 w2610] -> w2525
      tunnel: [w2549 w2562 w2580 w2586 w2594 w2598 w2604 w2605 w2607 w2609] -> w2517
      tunnel: w2523 -> [w2546 w2561 w2579 w2584 w2590 w2599 w2603 w2606 w2608 w2610]
      tunnel: w2522 -> [w2544 _ w2581 w2587 w2594 w2600 w2604 w2605 w2607 w2609]
      tunnel: w2521 -> [w2550 w2560 _ _ _ _ _ _ _ _]
      tunnel: [w2542 w2558 w2582 w2588 w2591 w2595 _ _ _ _] -> w2519
      tunnel: [_ _ _ _ _ TRUE _ _ _ _] -> w2516
      tunnel: [w2543 w2559 w2583 w2589 w2592 w2596 _ _ _ _] -> w2513
      frame "Connect" {
        w2542 = PLC_Comm_State."Write"  # Enum
        w2555 = TRUE  # Use Rack/Slot for S71200/1500
        w2554 = u8 1  # Slot S7 300/400
        w2552 = u8 0  # Rack S7 300/400
        # "Reconect"
        n791 = call <vilib>:"disconnect.vi"("error in (no error)"=w2546, "S7 Connection in"=w2544) -> ("error out"=w2547:errorcluster)  [unwired: 8 in, 1 out]
        n792 = call <vilib>:"Clear Errors.vi"("error in (no error)"=w2547) -> ("error out"=w2545:errorcluster)  [unwired: 5 in, 1 out]
        n793 = call <vilib>:"connect.vi"("Use Rack/Slot for S71200/1500"=w2555, "Slot S7 300/400"=w2554, "PLC Type"=PLC_Type."S7 1200" ("PLC Type 2"), "error in (no error)"=w2545, "Rack S7 300/400"=w2552, "timeout [ms]"=1000 ("timeout [ms] 2"), "IP address"=w2550) -> ("error out"=w2548:errorcluster, "S7 Connection out"=w2549:T5)  [unwired: 3 in]
      }
      frame "Int" {
        w2558 = PLC_Comm_State."Write"  # Enum
        w2564 = TRUE  # Use Rack/Slot for S71200/1500
        w2565 = u8 1  # Slot S7 300/400
        w2566 = u8 0  # Rack S7 300/400
        w2567 = u16[] [37]  # Data Block #
        n794 = call "Stall Data Flow.vim"("value in"=w2561, "milliseconds to wait"=u32 129) -> ("value out"=w2557:errorcluster)  [unwired: 1 out]
        n795 = call <vilib>:"connect.vi"("Use Rack/Slot for S71200/1500"=w2564, "Slot S7 300/400"=w2565, "PLC Type"=PLC_Type."S7 1200" ("PLC Type 2"), "error in (no error)"=w2557, "Rack S7 300/400"=w2566, "timeout [ms]"=1000 ("timeout [ms] 2"), "IP address"=w2560) -> ("error out"=w2569:errorcluster, "S7 Connection out"=w2568:T5)  [unwired: 3 in]
        n796 = for {
          tunnel: w2567 -> [w2577] mode=indexing
          shift-right: [w2575] -> w2562
          shift-left: w2568 -> [w2573]
          tunnel: w2569 -> [w2574]
          tunnel: [w2572] -> w2563
          w2576 = i32[] [0, 0]  # DINT input array
          # "Reset Search and save \nbit on software start"
          n797 = call-poly <vilib>:"write DB.vi"("DINT input array"=w2576, "error in (no error)"=w2574, "Data Block #"=w2577, "S7 Connection in"=w2573) -> ("error out"=w2572:errorcluster, "S7 Connection out"=w2575:T5)  [unwired: 4 in, 2 out]
        }
      }
      frame "Write" {
        w2582 = PLC_Comm_State."Read"  # Enum
        n798 = call "PLC_OP30_Write.vi"("error in (no error)"=w2579, "S7 Connection in"=w2581) -> ("error out"=w2578:errorcluster, "S7 Connection out"=w2580:T5)  [unwired: 8 in]
      }
      frame "Read" {
        w2588 = PLC_Comm_State."Write"  # Enum
        # "OP100 OK\nOP 100 NG"
        n799 = call "PLC_OP30_Read.vi"("error in (no error)"=w2584, "S7 Connection in"=w2587) -> ("error out"=w2585:errorcluster, "S7 Connection out 2"=w2586:T5)  [unwired: 8 in]
      }
      frame "Error" {
        w2591 = PLC_Comm_State."Write"  # Enum
        n800 = global write "Global 1.vi" "PLC2 error"(w2590) -> ()
        n801 = call <vilib>:"Clear Errors.vi"("error in (no error)"=w2590) -> ("error out"=w2593:errorcluster)  [unwired: 5 in, 1 out]
      }
      frame "Disconnect" {
        w2595 = PLC_Comm_State."Disconnect"  # Enum
        w2598 = T5 {"TCP Connection Ref"=refnum, "IP address"="", "timeout ms"=5000, "Connected?"=FALSE, "PLC Type"=enum."S7 1200", "Rack S7 400"=0, "Slot S7 400"=0, "PDU Size"=0, "connection semaphore"=refnum}  # S7 Connection out
        n802 = call <vilib>:"Clear Errors.vi"("error in (no error)"=w2599) -> ("error out"=w2602:errorcluster)  [unwired: 5 in, 1 out]
        n803 = call <vilib>:"disconnect.vi"("error in (no error)"=w2602, "S7 Connection in"=w2600) -> ("error out"=w2601:errorcluster)  [unwired: 8 in, 1 out]
      }
      frame "Write2" {
        # "SPARE"
      }
      frame "Write3" {
        # "No Use"
      }
      frame "Read2" {
        # "No Use"
      }
      frame "Read3" {
        # "No Use"
      }
    }
    n804 = Wait (ms)(milliseconds to wait=w2520) -> ()  [unwired: 1 out]
    n805 = call "PADMINI_STOP_ALL.vi"("Enum"=enum16{"Read", "Write"}."Read") -> ("Boolean 2"=w2511:bool)  [unwired: 9 in, 1 out]
    n806 = local read "stop"() -> (w2510:bool)
    n807 = case shown="Error" w2525 {
      selector: w2525 -> [w2528 w2531]
      tunnel: [w2528 w2535] -> w2505
      tunnel: [w2527 w2530] -> w2514
      tunnel: w2519 -> [w2527 _]
      tunnel: [w2526 w2541] -> w2518
      tunnel: w2517 -> [w2526 w2541]
      tunnel: w2513 -> [_ w2539]
      frame No Error {
      }
      frame Error {
        w2532 = PLC_Comm_State."Connect"  # Enum
        w2529 = PLC_Comm_State."Error"  # Enum
        n808 = Unbundle By Name(w2531) -> ("source"=w2540:string)
        n809 = call <userlib>:"Get Strings from Enum__ogtk.vi"("Enum"=w2539) -> ("String Value"=w2538:string)  [unwired: 7 in, 3 out]
        n810 = Concatenate Strings(w2538, "    " ("string"), w2540) -> (w2536:string)
        n811 = Bundle By Name(cluster=w2531, "source"=w2536) -> (w2535:errorcluster)
        n812 = call <vilib>:"Clear Errors.vi"("error in (no error)"=w2531, "specific error code to clear (0: all)"=6002) -> ("specific error cleared?"=w2534:bool)  [unwired: 4 in, 1 out]
        n813 = Select(t=w2532, s=w2534, f=w2529) -> (s? t:f=w2530:T1)
      }
    }
    n814 = Or(x=w2510, y=w2511) -> (x .or. y?=w2508:bool)
    n815 = Select(t=w2512, s=w2508, f=w2514) -> (s? t:f=w2515:T1)
    n816 = Unbundle By Name(w2505) -> ("status"=w2507:bool)
    n817 = Not(x=w2507) -> (.not. x?=w2506:bool)
    n818 = global write "Global 1.vi" "PLC 2"(w2506) -> ()
  }
  n819 = Merge Errors(w84, w3, w4, w6) -> (w80:errorcluster)
  n820 = call <vilib>:"Clear Errors.vi"("error in (no error)"=w117) -> ("error out"=w107:errorcluster)  [unwired: 5 in, 1 out]
  n821 = call <vilib>:"disconnect.vi"("error in (no error)"=w107, "S7 Connection in"=w106) -> ("error out"=w105:errorcluster)  [unwired: 8 in, 1 out]
  n822 = Merge Errors(w5, w2, w7) -> (w28:errorcluster)
  n823 = Merge Errors(w105, w80, w28) -> (w122:errorcluster)
  n824 = call <vilib>:"Simple Error Handler.vi"("type of dialog (OK msg:1)"=w10, "error in (no error)"=w122) -> ("error out"=w121:errorcluster)  [unwired: 3 in, 4 out]
  n825 = control-ref of="This VI"() -> (w11:refnum<vi>)
  n826 = call <vilib>:"Clear Errors.vi"("error in (no error)"=w121) -> ("error out"=w120:errorcluster)  [unwired: 5 in, 1 out]
  n827 = invoke class="VI" method="FP.Close"(reference=w11, error in=w120) -> (error out=→"error out":errorcluster)  [unwired: 1 in, 2 out]
